vi "数据采集传输系统.vi"() -> ()   [LabVIEW 2016, in "数据传输系统.lvlib"]
uses:
  <vilib>/Utility/miscctls.llb/LVPointTypeDef.ctl
  <vilib>/Utility/config.llb/Read Key (String).vi
  <vilib>/Utility/config.llb/Read Key (Boolean).vi
  <vilib>/Utility/config.llb/Read Key (I32).vi
  <vilib>/Utility/config.llb/Write Key (String).vi
  <vilib>/Utility/config.llb/Write Key (U32).vi
  <vilib>/Utility/config.llb/Write Key (I32).vi
  <vilib>/Utility/config.llb/Write Key (Boolean).vi
  <vilib>/Utility/config.llb/NI_LVConfig.lvlib
  data/FreeMem.dll
  <vilib>/ptbypt/NI_PtbyPt.lvlib
panel:
  in  "实时数据发送时间间隔/min":i32=1
  in  "数据组合发送":bool
  in  "日志、参数发送":bool
  in  "2011发送":bool
  in  "判断数据反馈":bool
  in  "数据发送协议":enum16{"2005-212协议", "2017-212协议"}(ring)=enum."2017-212协议"
  in  "数据发送通道":enum16{"TCP", "VISA"}(ring)
  in  "baud rate":u32=9600 caption="波特率"
  in  "VISA resource name":refnum<visa-resource-name> caption="VISA资源名称"
  in  "查询质控数据起始时间":bool
  in  "返回主界面":bool
  out "零点核查索引起始时间":string
  out "跨度核查索引起始时间":string
  out "加标回收索引起始时间":string
  out "标样核查索引起始时间":string
  out "数据接收超时指示灯":bool
  in  "重发时间":T1(ring)
  in  "重发日期":T2(ring)
  in  "锁":bool
  in  "开机启动":bool
  in  "确定更改起始时间":bool
  in  "更改起始时间":bool
  in  "数据发送起始时间":timestamp format="%<%.3X\n%Y/%m/%d>T"
  in  "每周自动重发":bool=TRUE
  in  "确定":bool
  in  "返回":bool
  in  "PW":string
  in  "MN":string
  in  "PORT":string
  in  "IP":string
  in  "站点设备":string
  in  "站点名称":string
  out "设置超时时间/min":i32=1
  out "空闲时间/s":string
  out "状态信息":T3={"1st Error to Convert "=63, "步骤 "=enum."打开连接", "元素"="实时数据", "TCP服务端掉线计数"=4, "TCP掉线时间节点"="2019/05/08 15:24:17"} {"1st Error to Convert" items=["无错误", "参数错误", "内存已满", "超出区域", "文件结束", "文件已打开", "一般文件IO错误", "未找到文件", "文件权限错误", "磁盘已满", "路径副本", "打开过多文件", "未启用", "未找到资源文件", "无法添加资源", "未找到资源", "未找到图像", "图像内存错误", "画笔不存在", "配置错误类型", "配置未找到解析段", "配置解析错误", "配置内存错误", "错误外部代码格式", "错误外部代码偏移量", "外部代码不存在", "空窗口", "销毁窗口错误", "空菜单", "打印已中止", "错误打印记录", "打印驱动程序错误", "打印时窗口错误", "打印时内存错误", "打印对话框错误", "一般打印错误", "无效设备引用句柄", "设备未找到", "设备参数错误", "设备单位错误", "无法打开设备", "设备调用已中止", "一般错误", "用户已取消", "对象ID过低", "对象ID过高", "对象不在堆中", "未知的堆", "错误DefProc ID", "DefProc不在表格中", "范围外信息", "空方法", "未知信息", "不支持管理器调用", "错误地址", "连接过程中", "连接超时", "连接过程中", "不支持网络属性", "网络错误", "正在使用的地址", "系统缺少内存", "连接已中止", "连接已拒绝", "连接未建立", "连接已建立", "连接已关闭", "初始化错误（交互应用程序管理器）", "错误事件发生", "等待无约束事件发生处理程序", "事件发生队列溢出", "错误路径", "未发出信号量", "未识别类型（交互应用程序管理器）"]}
  out "系统时间":string
  out "实时小时数据上传":bool
  out "系统状态改变":bool
  out "软件版本":string
  out "掉线指示":bool
  out "核查数据上传":bool
  out "通信状态":bool
  out "配置信息":T4
  in  "参数配置":bool
  out "查询数据发送":bool
  out "读取报文显示":string
  out "发送报文显示":string
  out "心跳包":bool
  in  "参数数值":T5={"CODMn"=TRUE, "CODCr"=TRUE, "DO"=TRUE, "铜"=TRUE, "PH"=TRUE, "氨氮"=TRUE, "比电导率"=TRUE, "水温"=TRUE, "盐度(海水)"=TRUE, "浊度"=TRUE, "总氮"=TRUE, "总磷"=TRUE, "叶绿素a"=TRUE, "藻密度"=TRUE, "水位"=TRUE, "流速"=TRUE, "瞬时流量"=TRUE, "累积流量"=TRUE}
  in  "系统编码选择框":string(combo)="地表水质量监测"
  out "主队列输出":refnum<queue>
  in  "TCP掉线时间节点":string
  out "TCP服务端掉线计数":i32
  out "元素":string
  out "步骤":T6(ring)
  out "1st Error to Convert":i32(ring)=56 items=["无错误", "参数错误", "内存已满", "超出区域", "文件结束", "文件已打开", "一般文件IO错误", "未找到文件", "文件权限错误", "磁盘已满", "路径副本", "打开过多文件", "未启用", "未找到资源文件", "无法添加资源", "未找到资源", "未找到图像", "图像内存错误", "画笔不存在", "配置错误类型", "配置未找到解析段", "配置解析错误", "配置内存错误", "错误外部代码格式", "错误外部代码偏移量", "外部代码不存在", "空窗口", "销毁窗口错误", "空菜单", "打印已中止", "错误打印记录", "打印驱动程序错误", "打印时窗口错误", "打印时内存错误", "打印对话框错误", "一般打印错误", "无效设备引用句柄", "设备未找到", "设备参数错误", "设备单位错误", "无法打开设备", "设备调用已中止", "一般错误", "用户已取消", "对象ID过低", "对象ID过高", "对象不在堆中", "未知的堆", "错误DefProc ID", "DefProc不在表格中", "范围外信息", "空方法", "未知信息", "不支持管理器调用", "错误地址", "连接过程中", "连接超时", "连接过程中", "不支持网络属性", "网络错误", "正在使用的地址", "系统缺少内存", "连接已中止", "连接已拒绝", "连接未建立", "连接已建立", "连接已关闭", "初始化错误（交互应用程序管理器）", "错误事件发生", "等待无约束事件发生处理程序", "事件发生队列溢出", "错误路径", "未发出信号量", "未识别类型（交互应用程序管理器）"]
  out "QN":string
  out "时间QN":string
  out "系统编码ST":string
  out "命令编码CN":string
  out "密码PW":string
  out "设备编码MN":string
  out "拆分包及应答Flag":string
  out "数据":string
  in  "实时数据参数选择框":T7={"水样测量数据"=FALSE, "零点核查数据"=TRUE, "跨度核查数据"=TRUE, "加标回收数据"=TRUE, "平行样数据"=FALSE, "标样核查"=TRUE, "集成干预测试"=TRUE}
  out "数据输出":string
  in  "table元素":string
  out "空闲时间":dbl
  out "错误输出":errorcluster
  # "数 据 采 集 传 输 系 统"
  # "读取的参数区"
  # "水样测量数据"
  # "空白测试数据"
  # "跨度核查数据"
  # "加标回收数据"
  # "平行样数据"
  # "标样核查"
  # "集成干预测试"
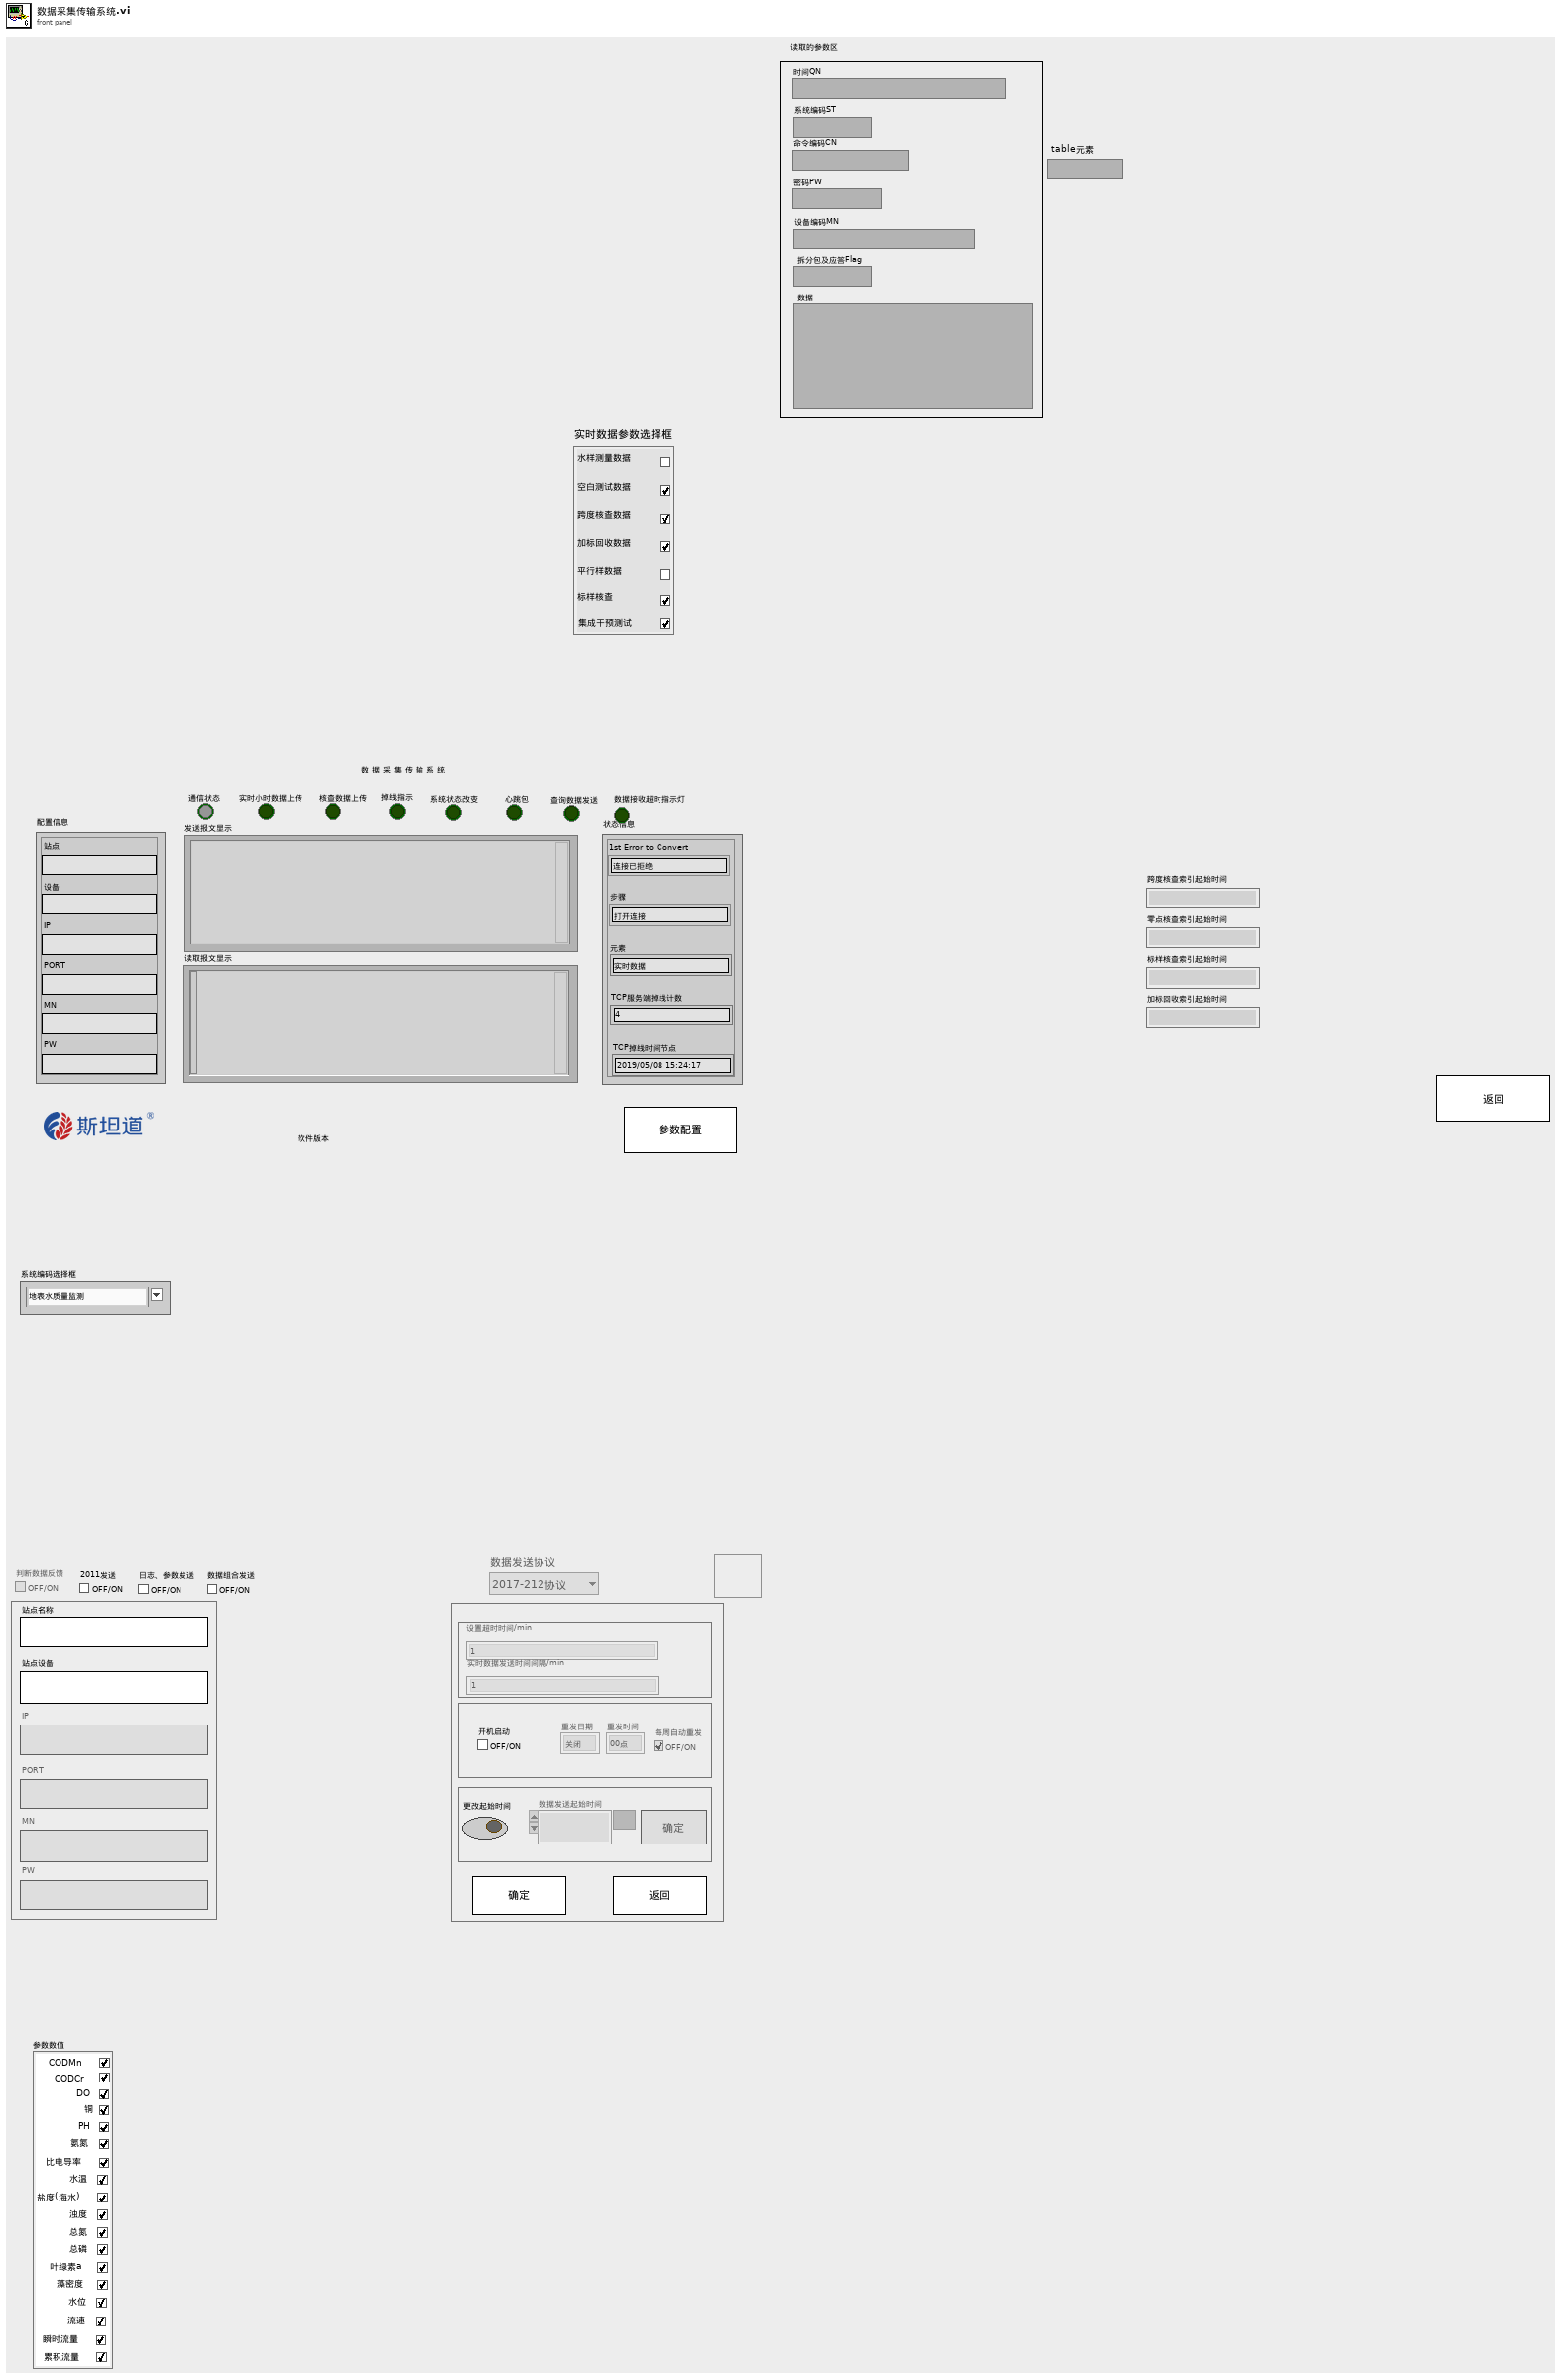
[diagram p1: front panel]
types:
  T1 = enum16{"00点", "01点", "02点", "03点", "04点", "05点", "06点", "07点", "08点", "09点", "10点", "11点", "12点", "13点", "14点", "15点", "16点", "17点", "18点", "19点", "20点", "21点", "22点", "23点"}
  T2 = enum16{"关闭", "星期日", "星期一", "星期二", "星期三", "星期四", "星期五", "星期六"}
  T3 = cluster{"1st Error to Convert ":i32, "步骤 ":enum16{"初始化", "打开连接", "表格比对", "发送数据", "读取数据", "数据处理"}, "元素":string, "TCP服务端掉线计数":i32, "TCP掉线时间节点":string}
  T4 = cluster{"站点":string, "设备":string, "IP":string, "PORT":string, "MN":string, "PW":string}
  T5 = cluster{"CODMn":bool, "CODCr":bool, "DO":bool, "铜":bool, "PH":bool, "氨氮":bool, "比电导率":bool, "水温":bool, "盐度(海水)":bool, "浊度":bool, "总氮":bool, "总磷":bool, "叶绿素a":bool, "藻密度":bool, "水位":bool, "流速":bool, "瞬时流量":bool, "累积流量":bool}
  T6 = enum16{"初始化", "打开连接", "表格比对", "发送数据", "读取数据", "数据处理"}
  T7 = cluster{"水样测量数据":bool, "零点核查数据":bool, "跨度核查数据":bool, "加标回收数据":bool, "平行样数据":bool, "标样核查":bool, "集成干预测试":bool}
  T8 = typedef "NI_LVConfig.lvlib/Config Data RefNum.ctl" = refnum<k1>
  T9 = typedef "LVDateTimeRec.ctl" = cluster{"秒数的小数部分":dbl, "秒":i32, "分":i32, "时":i32, "日":i32, "月":i32, "年":i32, "天数（周）":i32, "天数（年）":i32, "DST":i32}
  T10 = cluster{"PH":string[][], "CODCr":string[][], "氨氮":string[][], "CODMn":string[][], "总氮":string[][], "总磷":string[][], "电导率":string[][], "水温":string[][], "DO":string[][], "浊度":string[][], "叶绿素":string[][], "藻密度":string[][], "铜":string[][], "盐度":string[][], "水位":string[][], "流速":string[][], "瞬时流量":string[][], "累积流量":string[][]}
  T11 = typedef "LVPointTypeDef.ctl" = cluster{"Horizontal":i16, "Vertical":i16}
  T12 = enum8{"Enabled", "Disabled", "Disabled and Grayed Out"}
  T13 = enum16{"水样测试", "小时数据", "日志信息", "报警信息", "零点核查", "标样核查", "平行样", "加标回收"}
  T14 = typedef "imagedata.ctl" = cluster{"image type":i32, "image depth":i32, "image":u8[], "mask":u8[], "colors":u32[], "Rectangle":cluster{"left":i16, "top":i16, "right":i16, "bottom":i16}}
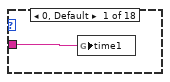
[diagram p6: hidden frame]
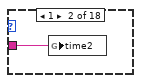
[diagram p7: hidden frame]
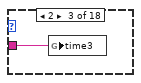
[diagram p8: hidden frame]
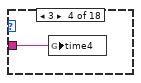
[diagram p9: hidden frame]
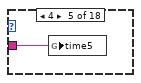
[diagram p10: hidden frame]
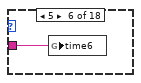
[diagram p11: hidden frame]
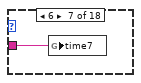
[diagram p12: hidden frame]
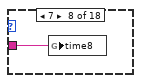
[diagram p13: hidden frame]
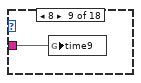
[diagram p14: hidden frame]
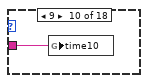
[diagram p15: hidden frame]
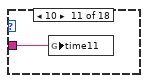
[diagram p16: hidden frame]
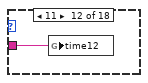
[diagram p17: hidden frame]
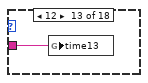
[diagram p18: hidden frame]
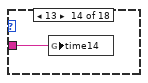
[diagram p19: hidden frame]
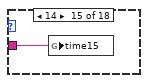
[diagram p20: hidden frame]
diagram:
  w27 = 0 ("索引")
  # "上传本地时间点的实时数据"
  # "目前时间太短，如果掉线了，数据存不了临时表格"
  n1 = Cluster To Array(cluster="参数数值") -> (array=w38:bool[])
  n2 = for {
    tunnel: w38 -> [_] mode=indexing
    tunnel: [w72] -> w37
    i -> [w72]
    w61 = "线程一数据重发功能" ("section")
    # "初始化水样搜索起始时间"
    n3 = case shown="3" w72 {
      tunnel: [w103 w105 w107 w109 w111 w113 w115 w117 w119 w121 w123 w125 w127 w129 w131 w133 w135 w137] -> w76
      frame 0, Default {
        n4 = control-ref of="CODMn"() -> (w104:refnum<vi>)
        n5 = property class="Bool (严格)"(reference=w104) -> ("Label.Text"=w103:string)  [unwired: 1 in, 2 out]
      }
      frame 1 {
        n6 = control-ref of="CODCr"() -> (w106:refnum<vi>)
        n7 = property class="Bool (严格)"(reference=w106) -> ("Label.Text"=w105:string)  [unwired: 1 in, 2 out]
      }
      frame 2 {
        n8 = control-ref of="DO"() -> (w108:refnum<vi>)
        n9 = property class="Bool (严格)"(reference=w108) -> ("Label.Text"=w107:string)  [unwired: 1 in, 2 out]
      }
      frame 3 {
        n10 = control-ref of="铜"() -> (w110:refnum<vi>)
        n11 = property class="Bool (严格)"(reference=w110) -> ("Label.Text"=w109:string)  [unwired: 1 in, 2 out]
      }
      frame 4 {
        n12 = control-ref of="PH"() -> (w112:refnum<vi>)
        n13 = property class="Bool (严格)"(reference=w112) -> ("Label.Text"=w111:string)  [unwired: 1 in, 2 out]
      }
      frame 5 {
        n14 = control-ref of="氨氮"() -> (w114:refnum<vi>)
        n15 = property class="Bool (严格)"(reference=w114) -> ("Label.Text"=w113:string)  [unwired: 1 in, 2 out]
      }
      frame 6 {
        n16 = control-ref of="比电导率"() -> (w116:refnum<vi>)
        n17 = property class="Bool (严格)"(reference=w116) -> ("Label.Text"=w115:string)  [unwired: 1 in, 2 out]
      }
      frame 7 {
        n18 = control-ref of="水温"() -> (w118:refnum<vi>)
        n19 = property class="Bool (严格)"(reference=w118) -> ("Label.Text"=w117:string)  [unwired: 1 in, 2 out]
      }
      frame 8 {
        n20 = control-ref of="盐度(海水)"() -> (w120:refnum<vi>)
        n21 = property class="Bool (严格)"(reference=w120) -> ("Label.Text"=w119:string)  [unwired: 1 in, 2 out]
      }
      frame 9 {
        n22 = control-ref of="浊度"() -> (w122:refnum<vi>)
        n23 = property class="Bool (严格)"(reference=w122) -> ("Label.Text"=w121:string)  [unwired: 1 in, 2 out]
      }
      frame 10 {
        n24 = control-ref of="总氮"() -> (w124:refnum<vi>)
        n25 = property class="Bool (严格)"(reference=w124) -> ("Label.Text"=w123:string)  [unwired: 1 in, 2 out]
      }
      frame 11 {
        n26 = control-ref of="总磷"() -> (w126:refnum<vi>)
        n27 = property class="Bool (严格)"(reference=w126) -> ("Label.Text"=w125:string)  [unwired: 1 in, 2 out]
      }
      frame 12 {
        n28 = control-ref of="叶绿素a"() -> (w128:refnum<vi>)
        n29 = property class="Bool (严格)"(reference=w128) -> ("Label.Text"=w127:string)  [unwired: 1 in, 2 out]
      }
      frame 13 {
        n30 = control-ref of="藻密度"() -> (w130:refnum<vi>)
        n31 = property class="Bool (严格)"(reference=w130) -> ("Label.Text"=w129:string)  [unwired: 1 in, 2 out]
      }
      frame 14 {
        n32 = control-ref of="水位"() -> (w132:refnum<vi>)
        n33 = property class="Bool (严格)"(reference=w132) -> ("Label.Text"=w131:string)  [unwired: 1 in, 2 out]
      }
      frame 15 {
        n34 = control-ref of="流速"() -> (w134:refnum<vi>)
        n35 = property class="Bool (严格)"(reference=w134) -> ("Label.Text"=w133:string)  [unwired: 1 in, 2 out]
      }
      frame 16 {
        n36 = control-ref of="瞬时流量"() -> (w136:refnum<vi>)
        n37 = property class="Bool (严格)"(reference=w136) -> ("Label.Text"=w135:string)  [unwired: 1 in, 2 out]
      }
      frame 17 {
        n38 = control-ref of="累积流量"() -> (w138:refnum<vi>)
        n39 = property class="Bool (严格)"(reference=w138) -> ("Label.Text"=w137:string)  [unwired: 1 in, 2 out]
      }
    }
    n40 = call <vilib>:"Application Directory.vi"() -> ("Application Directory"=w82:path)
    n41 = Build Path(base path=w82, name or relative path="data\\Set.ini" ("名称或相对路径")) -> (appended path=w80:path)
    n42 = call <vilib>:"Open Config Data.vi"("configuration file path"=w80) -> ("error out"=w78:errorcluster, "refnum"=w79:T8)  [unwired: 8 in, 1 out]
    n43 = call-poly <vilib>:"Read Key.vi"("section"="线程一数据搜索起始时间", "error in (no error)"=w78, "key"=w76, "refnum"=w79) -> ("error out"=w70:errorcluster, "value"=w73:string, "refnum out"=w71:T8)  [unwired: 4 in, 1 out]
    n44 = Empty String/Path?(string/path=w73) -> (empty?=w75:bool)
    n45 = case shown="真" w75 {
      tunnel: [w83 "1904/01/01 00:00:00"] -> w74
      tunnel: w73 -> [w83 _]
      frame False {
      }
      frame True {
      }
    }
    n46 = call-poly <vilib>:"Read Key.vi"("section"=w61, "error in (no error)"=w70, "key"="重发功能", "refnum"=w71) -> ("error out"=w64:errorcluster, "value"=w68:bool, "refnum out"=w65:T8)  [unwired: 4 in, 1 out]
    n47 = local write "每周自动重发"(w68) -> ()
    n48 = call-poly <vilib>:"Read Key.vi"("section"=w61, "error in (no error)"=w64, "key"="重发日期", "refnum"=w65) -> ("error out"=w62:errorcluster, "value"=w58:i32, "refnum out"=w63:T8)  [unwired: 4 in, 1 out]
    n49 = local write "重发日期"(w58) -> ()
    n50 = case shown="3" w72 {
      tunnel: w74 -> [w85 w86 w87 w88 w89 w90 w91 w92 w93 w94 w95 w96 w97 w98 w99 w100 w101 w102]
      frame 0, Default {
        n51 = global write "全局 水样时间.vi" "time1"(w85) -> ()
      }
      frame 1 {
        n52 = global write "全局 水样时间.vi" "time2"(w86) -> ()
      }
      frame 2 {
        n53 = global write "全局 水样时间.vi" "time3"(w87) -> ()
      }
      frame 3 {
        n54 = global write "全局 水样时间.vi" "time4"(w88) -> ()
      }
      frame 4 {
        n55 = global write "全局 水样时间.vi" "time5"(w89) -> ()
      }
      frame 5 {
        n56 = global write "全局 水样时间.vi" "time6"(w90) -> ()
      }
      frame 6 {
        n57 = global write "全局 水样时间.vi" "time7"(w91) -> ()
      }
      frame 7 {
        n58 = global write "全局 水样时间.vi" "time8"(w92) -> ()
      }
      frame 8 {
        n59 = global write "全局 水样时间.vi" "time9"(w93) -> ()
      }
      frame 9 {
        n60 = global write "全局 水样时间.vi" "time10"(w94) -> ()
      }
      frame 10 {
        n61 = global write "全局 水样时间.vi" "time11"(w95) -> ()
      }
      frame 11 {
        n62 = global write "全局 水样时间.vi" "time12"(w96) -> ()
      }
      frame 12 {
        n63 = global write "全局 水样时间.vi" "time13"(w97) -> ()
      }
      frame 13 {
        n64 = global write "全局 水样时间.vi" "time14"(w98) -> ()
      }
      frame 14 {
        n65 = global write "全局 水样时间.vi" "time15"(w99) -> ()
      }
      frame 15 {
        n66 = global write "全局 水样时间.vi" "time16"(w100) -> ()
      }
      frame 16 {
        n67 = global write "全局 水样时间.vi" "time17"(w101) -> ()
      }
      frame 17 {
        n68 = global write "全局 水样时间.vi" "time18"(w102) -> ()
      }
    }
    n69 = call-poly <vilib>:"Read Key.vi"("section"=w61, "error in (no error)"=w62, "key"="重发时间", "refnum"=w63) -> ("error out"=w59:errorcluster, "value"=w57:i32, "refnum out"=w60:T8)  [unwired: 4 in, 1 out]
    n70 = local write "重发时间"(w57) -> ()
    n71 = call <vilib>:"Close Config Data.vi"("error in (no error)"=w59, "refnum"=w60) -> ()  [unwired: 8 in, 2 out]
  }
  n72 = vi-ref "数据传输系统.lvlib:主动上传工控机周期和模式 (子VI).vi"() -> (w18:refnum<vi>)
  n73 = property class="VI"(reference=w18) -> ("Name"=w19:string)  [unwired: 1 in, 2 out]
  n74 = vi-ref "数据传输系统.lvlib:核查数据和日志信息入发送队列 (子VI).vi"() -> (w9:refnum<vi>)
  n75 = local read "实时小时数据上传"() -> (w5:bool)
  n76 = Open VI Reference(type specifier VI Refnum (for type only)=refnum<vi> refnum, vi path=w19, options=128 ("选项")) -> (vi reference=w21:refnum<vi>, error out=w23:errorcluster)  [unwired: 3 in]
  n77 = local read "核查数据上传"() -> (w8:bool)
  n78 = local read "查询数据发送"() -> (w7:bool)
  n79 = local read "日志、参数发送"() -> (w3:bool)
  n80 = property class="VI"(reference=w9) -> ("Name"=w16:string)  [unwired: 1 in, 2 out]
  n81 = local read "步骤"() -> (w6:T6)
  n82 = call-by-ref "?"(reference=w21, error in=w23) -> (reference out=w25:refnum<vi>, error out=w24:errorcluster, "系统状态改变"=→"系统状态改变":bool)  [unwired: 11 in]
  n83 = local read "数据发送协议"() -> (w4:enum16{"2005-212协议", "2017-212协议"})
  n84 = Close Reference(reference=w25, error in (no error)=w24) -> ()  [unwired: 1 out]
  n85 = Open VI Reference(type specifier VI Refnum (for type only)=refnum<vi> refnum, vi path=w16, options=128 ("选项")) -> (vi reference=w14:refnum<vi>, error out=w12:errorcluster)  [unwired: 3 in]
  n86 = call-by-ref "?"(reference=w14, error in=w12, "实时数据参数选择框"="实时数据参数选择框", "实时数据发送时间间隔/min"="实时数据发送时间间隔/min", "日志、参数发送输入"=w3, "数据发送协议输入"=w4, "实时小时数据上传输入"=w5, "步骤输入"=w6, "查询数据发送输入"=w7, "核查数据上传输入"=w8) -> (reference out=w10:refnum<vi>, error out=w11:errorcluster)  [unwired: 4 in]
  n87 = Obtain Queue(name (unnamed)="数据发送" ("名称（未命名）"), element data type="") -> (queue out=w26:refnum<queue>, error out=w41:errorcluster)  [unwired: 3 in, 1 out]
  n88 = Obtain Queue(name (unnamed)="实时数据参数选择" ("名称（未命名）"), element data type="") -> (queue out=w42:refnum<queue>, error out=w40:errorcluster)  [unwired: 3 in, 1 out]
  n89 = Close Reference(reference=w10, error in (no error)=w11) -> ()  [unwired: 1 out]
  n90 = while "While循环" {
    tunnel: w26 -> [w149]
    tunnel: w42 -> [w153]
    tunnel: w41 -> [w152]
    tunnel: w40 -> [w151]
    stop <- FALSE stop-if-true
    # "判定数据发送时要发送实时数据"
    # "所有的主动上传数据都是有数据才会上传"
    n91 = Get Queue Status(queue=w149) -> (# elements in queue=w141:i32)  [unwired: 2 in, 7 out]
    n92 = local read "查询数据发送"() -> (w147:bool)
    n93 = global read "全局 数据发送重叠.vi" "主动上报数据中"() -> (w139:bool)
    n94 = Not Equal To 0?(x=w141) -> (x != 0?=w148:bool)
    n95 = And(x=w148, y=w147) -> (x .and. y?=w140:bool)
    n96 = call <vilib>:"Boolean Crossing PtByPt.vi"("direction"=enum16{"either", "false-true", "true-false"}."false-true", "input"=w140) -> ("crossing"=w146:bool)  [unwired: 1 in]
    n97 = Not(x=w139) -> (.not. x?=w143:bool)
    n98 = Not(x=w147) -> (.not. x?=w144:bool)
    n99 = case shown="真" w146 {
      frame False {
      }
      frame True {
        n100 = Get Date/Time In Seconds() -> (seconds since 1Jan1904=w159:timestamp)
        n101 = Seconds To Date/Time(time stamp (now)=w159) -> (date time rec=w156:T9)  [unwired: 1 in]
        n102 = Date/Time To Seconds(2:w156) -> (0:w158:timestamp)  [unwired: 1 in]
        n103 = Format Date/Time String(time format string (%c)="%Y/%m/%d %H:%M:%S" ("时间格式字符串(%c)"), seconds (now)=w158) -> (date/time string=w155:string)  [unwired: 1 in]
        n104 = global write "全局 数据发送重叠.vi" "数据发送重叠开始时间戳"(w155) -> ()
      }
    }
    n105 = Compound Arithmetic op=AND ("复合运算")(w144, w143) -> (w142:bool)
    n106 = Wait (ms)(milliseconds to wait=u32 1000 ("等待时间（毫秒）")) -> ()  [unwired: 1 out]
    n107 = case shown="真" w142 {
      tunnel: w149 -> [_ w169]
      tunnel: w153 -> [_ w168]
      tunnel: w152 -> [_ w167]
      tunnel: w151 -> [_ w166]
      tunnel: w141 -> [_ w162]
      tunnel: w140 -> [_ w161]
      frame False {
        n108 = local write "核查数据上传"(FALSE ("数据上传")) -> ()
      }
      frame True {
        n109 = Equal To 0?(x=w162) -> (x = 0?=w163:bool)
        n110 = global write "全局 数据发送重叠.vi" "数据发送重叠"(w161) -> ()
        n111 = Not(x=w163) -> (.not. x?=w164:bool)
        n112 = local write "核查数据上传"(w164) -> ()
        n113 = Dequeue Element(queue=w169, error in (no error)=w167) -> (element=w165:string)  [unwired: 1 in, 3 out]
        n114 = case shown="\"send\"" w165 {
          tunnel: w168 -> [_ w171 _ _ _ _ _ _ _ _ _]
          tunnel: w166 -> [_ w170 _ _ _ _ _ _ _ _ _]
          frame "假", Default {
          }
          frame "send" {
            # "间隔时间上传"
            n115 = while {
              tunnel: w171 -> [w175]
              tunnel: w170 -> [w172]
              stop <- w176 stop-if-true
              n116 = Dequeue Element(queue=w175, error in (no error)=w172) -> (queue out=w174:refnum<queue>, element=w177:string)  [unwired: 1 in, 2 out]
              n117 = case shown="\"空白测试\"" w177 {
                tunnel: [_ _ _ w343 _ _ _ w550] -> w176
                tunnel: w174 -> [_ _ _ _ _ _ _ w553]
                frame "水样测试" {
                  n118 = flat-sequence {
                    frame #0 {
                      n119 = global write "全局 小时数据发送次数.vi" "小时数据发送次数"(0 ("小时数据发送次数")) -> ()
                      n120 = global write "全局 实时数据参数.vi" "实时数据参数"("水样测试") -> ()
                      n121 = global write "全局1.vi" "枚举"(enum16{"返回请求应答", "上传数据", "返回执行结果"}."上传数据" ("枚举")) -> ()
                    }
                    frame #1 {
                      n122 = call "从数据库获取数据通用可配置(子VI).vi"("table输入"="实时数据" ("新元素/子数组"), "列队名（唯一）"="a") -> ()  [unwired: 8 in, 2 out]
                    }
                    frame #2 {
                      n123 = call "实时小时数据处理整合 (子VI).vi"("枚举"=enum16{"实时数据排序", "小时数据排序"}."实时数据排序") -> ("已排序的数组"=w184:string[])  [unwired: 10 in]
                      n124 = Array Size(array=w184) -> (size(s)=w185:i32)
                      n125 = global write "全局 数据数组大小.vi" "数据数组大小"(w185) -> ()
                    }
                    frame #3 {
                      n126 = while {
                        stop <- w190 stop-if-true
                        n127 = property on="TCP服务端掉线计数" class="DigNum (严格)"() -> ("Value"=w193:i32)  [unwired: 2 in, 2 out]
                        n128 = Greater Or Equal?(x=w193, y=1) -> (x >= y?=w192:bool)
                        n129 = case shown="假" w192 {
                          frame False {
                            n130 = global read "全局 数据数组大小.vi" "数据数组大小"() -> (w195:i32)
                            n131 = Greater Than 0?(x=w195) -> (x > 0?=w196:bool)
                            n132 = case shown="真" w196 {
                              frame False {
                              }
                              frame True {
                                n133 = local read "MN"() -> (w202:string)
                                n134 = local read "PW"() -> (w201:string)
                                n135 = local read "数据发送通道"() -> (w200:enum16{"TCP", "VISA"})
                                n136 = call "数据编码.vi"("table输入"="实时数据" ("新元素/子数组"), "MN"=w202, "PW"=w201) -> ("通讯包字符串"=w197:string)  [unwired: 11 in, 1 out]
                                n137 = local write "发送报文显示"(w197) -> ()
                                n138 = call "VISATCP组合选择发送.vi"("数据发送通道"=w200, "命令"="write", "写入缓冲区"=w197) -> ("错误输出"=→"错误输出":errorcluster)  [unwired: 9 in, 3 out]
                                n139 = Build Array(w197) -> (w204:string[])
                                n140 = call "发送数据记录到文档(子VI).vi"("数组"=w204) -> ()  [unwired: 9 in, 1 out]
                                "核查数据上传" <- TRUE ("主动数据上传")
                              }
                            }
                          }
                          frame True {
                          }
                        }
                        n141 = Wait (ms)(milliseconds to wait=u32 500 ("等待时间（毫秒）")) -> ()  [unwired: 1 out]
                        n142 = global read "全局 数据数组大小.vi" "数据数组大小"() -> (w187:i32)
                        n143 = global read "全局 小时数据发送次数.vi" "小时数据发送次数"() -> (w191:i32)
                        n144 = Decrement(x=w187) -> (x-1=w186:i32)
                        n145 = Greater Or Equal?(x=w191, y=w186) -> (x >= y?=w189:bool)
                        n146 = Compound Arithmetic op=OR ("复合运算")(w189) -> (w190:bool)
                      }
                    }
                  }
                }
                frame "空白测试" {
                  n147 = flat-sequence {
                    frame #0 {
                      n148 = global write "全局 小时数据发送次数.vi" "小时数据发送次数"(0 ("小时数据发送次数")) -> ()
                      n149 = global write "全局 实时数据参数.vi" "实时数据参数"("空白测试") -> ()
                      n150 = global write "全局1.vi" "枚举"(enum16{"返回请求应答", "上传数据", "返回执行结果"}."上传数据" ("枚举")) -> ()
                    }
                    frame #1 {
                      n151 = call "从数据库获取数据通用可配置(子VI).vi"("table输入"="实时数据" ("新元素/子数组"), "列队名（唯一）"="b") -> ()  [unwired: 8 in, 2 out]
                    }
                    frame #2 {
                      n152 = for {
                        N: 5 -> [_]
                        i -> [w213]
                        # "行数大于零"
                        n153 = case shown="3" w213 {
                          tunnel: [w217 w218 w219 w220 w221] -> w212
                          frame 0, Default {
                            n154 = global read "全局 所有参数.vi" "氨氮"() -> (w217:string[][])
                          }
                          frame 1 {
                            n155 = global read "全局 所有参数.vi" "总氮"() -> (w218:string[][])
                          }
                          frame 2 {
                            n156 = global read "全局 所有参数.vi" "总磷"() -> (w219:string[][])
                          }
                          frame 3 {
                            n157 = global read "全局 所有参数.vi" "CODMn"() -> (w220:string[][])
                          }
                          frame 4 {
                            n158 = global read "全局 所有参数.vi" "CODCr"() -> (w221:string[][])
                          }
                        }
                        n159 = Array Size(array=w212) -> (size(s)=w215:i32[])
                        n160 = Index Array(array=w215) -> (element=w214:i32)  [unwired: 1 in]
                        n161 = Greater Than 0?(x=w214) -> (x > 0?=w216:bool)
                        n162 = case shown="真" w216 {
                          tunnel: w213 -> [_ w227]
                          tunnel: w214 -> [_ _]
                          tunnel: w212 -> [_ w225]
                          frame False {
                          }
                          frame True {
                            # "最新时间戳加1分钟"
                            n163 = Index Array(array=w225, index (row)=0 ("禁用的索引 (行)"), index (col)=0 ("禁用的索引 (列)")) -> (element=w224:string)
                            n164 = call "日期时间字符串转换分钟数加一.vi"("data[0]"=w224) -> ("日期/时间字符串"=w223:string)  [unwired: 10 in]
                            n165 = case shown="0, 默认" w227 {
                              tunnel: w223 -> [w228 w229 w230 w231 w232]
                              frame 0, Default {
                                n166 = global write "全局 时间2.vi" "氨氮零点核查索引起始时间"(w228) -> ()
                              }
                              frame 1 {
                                n167 = global write "全局 时间2.vi" "总氮零点核查索引起始时间"(w229) -> ()
                              }
                              frame 2 {
                                n168 = global write "全局 时间2.vi" "总磷零点核查索引起始时间"(w230) -> ()
                              }
                              frame 3 {
                                n169 = global write "全局 时间2.vi" "CODMn零点核查索引起始时间"(w231) -> ()
                              }
                              frame 4 {
                                n170 = global write "全局 时间2.vi" "CODCr零点核查索引起始时间"(w232) -> ()
                              }
                            }
                          }
                        }
                      }
                    }
                    frame #3 {
                      n171 = call <vilib>:"Application Directory.vi"() -> ("Application Directory"=w246:path)
                      n172 = Build Path(base path=w246, name or relative path="data\\hecha.ini" ("名称或相对路径")) -> (appended path=w244:path)
                      n173 = call <vilib>:"Open Config Data.vi"("configuration file path"=w244) -> ("error out"=w240:errorcluster, "refnum"=w243:T8)  [unwired: 8 in, 1 out]
                      n174 = call "数据处理整合 (子VI).vi"("枚举"=enum16{"实时数据排序", "小时数据排序"}."实时数据排序") -> ("已排序的数组"=w249:string[])  [unwired: 10 in]
                      n175 = vi-ref "全局 时间2.vi"() -> (w242:refnum<vi>)
                      n176 = Array Size(array=w249) -> (size(s)=w248:i32)
                      n177 = call <userlib>:"Write Panel to INI__ogtk.vi"("error in (no error)"=w240, "VI ref"=w242, "refnum"=w243) -> ("error out"=w239:errorcluster, "refnum out"=w241:T8)  [unwired: 7 in]
                      n178 = call <vilib>:"Close Config Data.vi"("error in (no error)"=w239, "refnum"=w241) -> ("error out"=w234:errorcluster, "file path"=w233:path)  [unwired: 8 in]
                      n179 = global write "全局 数据数组大小.vi" "数据数组大小"(w248) -> ()
                      n180 = Open/Create/Replace File(file path (use dialog)=w233, error in=w234) -> (refnum out=w237:refnum<file>, error out=w238:errorcluster)  [unwired: 4 in, 1 out]
                      n181 = Flush File(refnum=w237, error in=w238) -> (refnum out=w236:refnum<file>, error out=w235:errorcluster)
                      n182 = Close File(refnum=w236, error in=w235) -> ()  [unwired: 2 out]
                    }
                    frame #4 {
                      n183 = while {
                        stop <- w252 stop-if-true
                        n184 = property on="TCP服务端掉线计数" class="DigNum (严格)"() -> ("Value"=w256:i32)  [unwired: 2 in, 2 out]
                        n185 = Greater Or Equal?(x=w256, y=1) -> (x >= y?=w255:bool)
                        n186 = case shown="假" w255 {
                          frame False {
                            n187 = global read "全局 数据数组大小.vi" "数据数组大小"() -> (w259:i32)
                            n188 = Greater Than 0?(x=w259) -> (x > 0?=w258:bool)
                            n189 = case shown="真" w258 {
                              frame False {
                              }
                              frame True {
                                w260 = 0 ("禁用的索引 (列)")
                                n190 = global read "插值后的新数组.vi" "插值后的数组元素"() -> (w270:T10)
                                n191 = local read "MN"() -> (w266:string)
                                n192 = local read "PW"() -> (w265:string)
                                n193 = local read "数据发送通道"() -> (w264:enum16{"TCP", "VISA"})
                                n194 = call "数据编码.vi"("table输入"="实时数据" ("新元素/子数组"), "MN"=w266, "PW"=w265) -> ("通讯包字符串"=w262:string)  [unwired: 11 in, 1 out]
                                n195 = Unbundle By Name(w270) -> ("氨氮"=w269:string[][])
                                n196 = local write "发送报文显示"(w262) -> ()
                                n197 = Build Array(w262) -> (w272:string[])
                                n198 = call "VISATCP组合选择发送.vi"("数据发送通道"=w264, "命令"="write", "写入缓冲区"=w262) -> ("错误输出"=w261:errorcluster)  [unwired: 9 in, 3 out]
                                n199 = Index Array(array=w269, index (row)=w260, index (col)=w260) -> (element=w268:string)
                                n200 = call "发送数据记录到文档(子VI).vi"("数组"=w272) -> ()  [unwired: 9 in, 1 out]
                                n201 = local write "错误输出"(w261) -> ()
                                n202 = call "日期时间字符串转换分钟数加一.vi"("data[0]"=w268) -> ("日期/时间字符串"=w267:string)  [unwired: 10 in]
                                n203 = global write "全局 时间2.vi" "零点核查索引起始时间"(w267) -> ()
                                n204 = local write "核查数据上传"(TRUE ("数据上传")) -> ()
                              }
                            }
                          }
                          frame True {
                          }
                        }
                        n205 = Wait (ms)(milliseconds to wait=u32 500 ("等待时间（毫秒）")) -> ()  [unwired: 1 out]
                        n206 = global read "全局 数据数组大小.vi" "数据数组大小"() -> (w250:i32)
                        n207 = global read "全局 小时数据发送次数.vi" "小时数据发送次数"() -> (w254:i32)
                        n208 = Greater Or Equal?(x=w254, y=w250) -> (x >= y?=w253:bool)
                        n209 = Compound Arithmetic op=OR ("复合运算")(w253) -> (w252:bool)
                      }
                    }
                  }
                }
                frame "跨度核查" {
                  n210 = flat-sequence {
                    frame #0 {
                      n211 = global write "全局 小时数据发送次数.vi" "小时数据发送次数"(0 ("小时数据发送次数")) -> ()
                      n212 = global write "全局 实时数据参数.vi" "实时数据参数"("跨度核查") -> ()
                      n213 = global write "全局1.vi" "枚举"(enum16{"返回请求应答", "上传数据", "返回执行结果"}."上传数据" ("枚举")) -> ()
                    }
                    frame #1 {
                      n214 = call "从数据库获取数据通用可配置(子VI).vi"("table输入"="实时数据" ("新元素/子数组"), "列队名（唯一）"="c") -> ()  [unwired: 8 in, 2 out]
                    }
                    frame #2 {
                      n215 = for {
                        N: 5 -> [_]
                        i -> [w280]
                        # "行数大于零"
                        n216 = case shown="3" w280 {
                          tunnel: [w285 w286 w287 w288 w289] -> w281
                          frame 0, Default {
                            n217 = global read "全局 所有参数.vi" "氨氮"() -> (w285:string[][])
                          }
                          frame 1 {
                            n218 = global read "全局 所有参数.vi" "总氮"() -> (w286:string[][])
                          }
                          frame 2 {
                            n219 = global read "全局 所有参数.vi" "总磷"() -> (w287:string[][])
                          }
                          frame 3 {
                            n220 = global read "全局 所有参数.vi" "CODMn"() -> (w288:string[][])
                          }
                          frame 4 {
                            n221 = global read "全局 所有参数.vi" "CODCr"() -> (w289:string[][])
                          }
                        }
                        n222 = Array Size(array=w281) -> (size(s)=w283:i32[])
                        n223 = Index Array(array=w283) -> (element=w282:i32)  [unwired: 1 in]
                        n224 = Greater Than 0?(x=w282) -> (x > 0?=w284:bool)
                        n225 = case shown="真" w284 {
                          tunnel: w280 -> [_ w295]
                          tunnel: w282 -> [_ _]
                          tunnel: w281 -> [_ w293]
                          frame False {
                          }
                          frame True {
                            # "最新时间戳加1分钟"
                            n226 = Index Array(array=w293, index (row)=0 ("禁用的索引 (行)"), index (col)=0 ("禁用的索引 (列)")) -> (element=w292:string)
                            n227 = call "日期时间字符串转换分钟数加一.vi"("data[0]"=w292) -> ("日期/时间字符串"=w291:string)  [unwired: 10 in]
                            n228 = case shown="3" w295 {
                              tunnel: w291 -> [w296 w297 w298 w299 w300]
                              frame 0, Default {
                                n229 = global write "全局 时间2.vi" "氨氮跨度核查索引起始时间"(w296) -> ()
                              }
                              frame 1 {
                                n230 = global write "全局 时间2.vi" "总氮跨度核查索引起始时间"(w297) -> ()
                              }
                              frame 2 {
                                n231 = global write "全局 时间2.vi" "总磷跨度核查索引起始时间"(w298) -> ()
                              }
                              frame 3 {
                                n232 = global write "全局 时间2.vi" "CODMn跨度核查索引起始时间"(w299) -> ()
                              }
                              frame 4 {
                                n233 = global write "全局 时间2.vi" "CODCr跨度核查索引起始时间"(w300) -> ()
                              }
                            }
                          }
                        }
                      }
                    }
                    frame #3 {
                      n234 = call <vilib>:"Application Directory.vi"() -> ("Application Directory"=w314:path)
                      n235 = call "数据处理整合 (子VI).vi"("枚举"=enum16{"实时数据排序", "小时数据排序"}."实时数据排序") -> ("已排序的数组"=w317:string[])  [unwired: 10 in]
                      n236 = Build Path(base path=w314, name or relative path="data\\hecha.ini" ("名称或相对路径")) -> (appended path=w312:path)
                      n237 = call <vilib>:"Open Config Data.vi"("configuration file path"=w312) -> ("error out"=w308:errorcluster, "refnum"=w311:T8)  [unwired: 8 in, 1 out]
                      n238 = Array Size(array=w317) -> (size(s)=w316:i32)
                      n239 = vi-ref "全局 时间2.vi"() -> (w310:refnum<vi>)
                      n240 = global write "全局 数据数组大小.vi" "数据数组大小"(w316) -> ()
                      n241 = call <userlib>:"Write Panel to INI__ogtk.vi"("error in (no error)"=w308, "VI ref"=w310, "refnum"=w311) -> ("error out"=w307:errorcluster, "refnum out"=w309:T8)  [unwired: 7 in]
                      n242 = call <vilib>:"Close Config Data.vi"("error in (no error)"=w307, "refnum"=w309) -> ("error out"=w302:errorcluster, "file path"=w301:path)  [unwired: 8 in]
                      n243 = Open/Create/Replace File(file path (use dialog)=w301, error in=w302) -> (refnum out=w305:refnum<file>, error out=w306:errorcluster)  [unwired: 4 in, 1 out]
                      n244 = Flush File(refnum=w305, error in=w306) -> (refnum out=w304:refnum<file>, error out=w303:errorcluster)
                      n245 = Close File(refnum=w304, error in=w303) -> ()  [unwired: 2 out]
                    }
                    frame #4 {
                      n246 = while {
                        stop <- w320 stop-if-true
                        n247 = property on="TCP服务端掉线计数" class="DigNum (严格)"() -> ("Value"=w324:i32)  [unwired: 2 in, 2 out]
                        n248 = property on="TCP服务端掉线计数" class="DigNum (严格)" props=["Value"]() -> ()  [unwired: 2 in, 3 out]
                        n249 = Greater Or Equal?(x=w324, y=1) -> (x >= y?=w323:bool)
                        n250 = case shown="假" w323 {
                          frame False {
                            n251 = global read "全局 数据数组大小.vi" "数据数组大小"() -> (w327:i32)
                            n252 = Greater Than 0?(x=w327) -> (x > 0?=w326:bool)
                            n253 = case shown="真" w326 {
                              frame False {
                              }
                              frame True {
                                w328 = 0 ("禁用的索引 (列)")
                                n254 = global read "插值后的新数组.vi" "插值后的数组元素"() -> (w338:T10)
                                n255 = local read "QN"() -> (w341:string)
                                n256 = local read "MN"() -> (w334:string)
                                n257 = local read "PW"() -> (w333:string)
                                n258 = local read "数据发送通道"() -> (w332:enum16{"TCP", "VISA"})
                                n259 = Unbundle By Name(w338) -> ("氨氮"=w337:string[][])
                                n260 = call "数据编码.vi"("table输入"="实时数据" ("新元素/子数组"), "QN"=w341, "MN"=w334, "PW"=w333) -> ("通讯包字符串"=w330:string)  [unwired: 10 in, 1 out]
                                n261 = local write "发送报文显示"(w330) -> ()
                                n262 = Index Array(array=w337, index (row)=w328, index (col)=w328) -> (element=w336:string)
                                n263 = call "VISATCP组合选择发送.vi"("数据发送通道"=w332, "命令"="write", "写入缓冲区"=w330) -> ("错误输出"=w329:errorcluster)  [unwired: 9 in, 3 out]
                                n264 = Build Array(w330) -> (w340:string[])
                                n265 = local write "核查数据上传"(TRUE ("数据上传")) -> ()
                                n266 = call "日期时间字符串转换分钟数加一.vi"("data[0]"=w336) -> ("日期/时间字符串"=w335:string)  [unwired: 10 in]
                                n267 = local write "错误输出"(w329) -> ()
                                n268 = call "发送数据记录到文档(子VI).vi"("数组"=w340) -> ()  [unwired: 9 in, 1 out]
                                n269 = global write "全局 时间2.vi" "跨度核查索引起始时间"(w335) -> ()
                              }
                            }
                          }
                          frame True {
                          }
                        }
                        n270 = Wait (ms)(milliseconds to wait=u32 500 ("等待时间（毫秒）")) -> ()  [unwired: 1 out]
                        n271 = global read "全局 数据数组大小.vi" "数据数组大小"() -> (w318:i32)
                        n272 = global read "全局 小时数据发送次数.vi" "小时数据发送次数"() -> (w322:i32)
                        n273 = Greater Or Equal?(x=w322, y=w318) -> (x >= y?=w321:bool)
                        n274 = Compound Arithmetic op=OR ("复合运算")(w321) -> (w320:bool)
                      }
                    }
                  }
                }
                frame "标样核查" {
                  n275 = flat-sequence {
                    tunnel: [w352] -> w343
                    frame #0 {
                      n276 = global write "全局 小时数据发送次数.vi" "小时数据发送次数"(0 ("小时数据发送次数")) -> ()
                      n277 = global write "全局 实时数据参数.vi" "实时数据参数"("核查数据") -> ()
                      n278 = global write "全局1.vi" "枚举"(enum16{"返回请求应答", "上传数据", "返回执行结果"}."上传数据" ("枚举")) -> ()
                    }
                    frame #1 {
                      n279 = call "从数据库获取数据通用可配置(子VI).vi"("table输入"="实时数据" ("新元素/子数组"), "列队名（唯一）"="n") -> ()  [unwired: 8 in, 2 out]
                    }
                    frame #2 {
                      n280 = call "数据处理整合 (子VI).vi"("枚举"=enum16{"实时数据排序", "小时数据排序"}."实时数据排序") -> ("已排序的数组"=w351:string[])  [unwired: 10 in]
                      n281 = Array Size(array=w351) -> (size(s)=w350:i32)
                      n282 = global write "全局 数据数组大小.vi" "数据数组大小"(w350) -> ()
                    }
                    frame #3 {
                      n283 = while {
                        tunnel: [w353] -> w352
                        stop <- w353 stop-if-true
                        n284 = property on="TCP服务端掉线计数" class="DigNum (严格)"() -> ("Value"=w359:i32)  [unwired: 2 in, 2 out]
                        n285 = property on="TCP服务端掉线计数" class="DigNum (严格)" props=["Value"]() -> ()  [unwired: 2 in, 3 out]
                        n286 = Greater Or Equal?(x=w359, y=1) -> (x >= y?=w358:bool)
                        n287 = case shown="假" w358 {
                          frame False {
                            n288 = global read "全局 数据数组大小.vi" "数据数组大小"() -> (w362:i32)
                            n289 = Greater Than 0?(x=w362) -> (x > 0?=w361:bool)
                            n290 = case shown="真" w361 {
                              frame False {
                              }
                              frame True {
                                w363 = 0 ("禁用的索引 (列)")
                                n291 = global read "插值后的新数组.vi" "插值后的数组元素"() -> (w373:T10)
                                n292 = local read "QN"() -> (w376:string)
                                n293 = local read "MN"() -> (w369:string)
                                n294 = local read "PW"() -> (w368:string)
                                n295 = local read "数据发送通道"() -> (w367:enum16{"TCP", "VISA"})
                                n296 = Unbundle By Name(w373) -> ("氨氮"=w372:string[][])
                                n297 = call "数据编码.vi"("table输入"="实时数据" ("新元素/子数组"), "QN"=w376, "MN"=w369, "PW"=w368) -> ("通讯包字符串"=w365:string)  [unwired: 10 in, 1 out]
                                n298 = local write "发送报文显示"(w365) -> ()
                                n299 = call "VISATCP组合选择发送.vi"("数据发送通道"=w367, "命令"="write", "写入缓冲区"=w365) -> ("错误输出"=w364:errorcluster)  [unwired: 9 in, 3 out]
                                n300 = Index Array(array=w372, index (row)=w363, index (col)=w363) -> (element=w371:string)
                                n301 = Build Array(w365) -> (w375:string[])
                                n302 = local write "核查数据上传"(TRUE ("数据上传")) -> ()
                                n303 = call "日期时间字符串转换分钟数加一.vi"("data[0]"=w371) -> ("日期/时间字符串"=w370:string)  [unwired: 10 in]
                                n304 = local write "错误输出"(w364) -> ()
                                n305 = call "发送数据记录到文档(子VI).vi"("数组"=w375) -> ()  [unwired: 9 in, 1 out]
                                n306 = global write "全局 时间2.vi" "标样核查索引起始时间"(w370) -> ()
                              }
                            }
                          }
                          frame True {
                          }
                        }
                        n307 = Wait (ms)(milliseconds to wait=u32 500 ("等待时间（毫秒）")) -> ()  [unwired: 1 out]
                        n308 = global read "全局 数据数组大小.vi" "数据数组大小"() -> (w354:i32)
                        n309 = global read "全局 小时数据发送次数.vi" "小时数据发送次数"() -> (w357:i32)
                        n310 = Greater Or Equal?(x=w357, y=w354) -> (x >= y?=w356:bool)
                        n311 = Compound Arithmetic op=OR ("复合运算")(w356) -> (w353:bool)
                      }
                    }
                  }
                }
                frame "加标回收" {
                  n312 = flat-sequence {
                    frame #0 {
                      n313 = global write "全局 小时数据发送次数.vi" "小时数据发送次数"(0 ("小时数据发送次数")) -> ()
                      n314 = global write "全局 实时数据参数.vi" "实时数据参数"("加标回收测试") -> ()
                      n315 = global write "全局1.vi" "枚举"(enum16{"返回请求应答", "上传数据", "返回执行结果"}."上传数据" ("枚举")) -> ()
                    }
                    frame #1 {
                      n316 = call "从数据库获取数据通用可配置(子VI).vi"("table输入"="加标回收" ("新元素/子数组"), "列队名（唯一）"="d") -> ()  [unwired: 8 in, 2 out]
                    }
                    frame #2 {
                      n317 = call "加标回收数据处理整合 (子VI).vi"("枚举"=enum16{"实时数据排序", "小时数据排序"}."实时数据排序") -> ("已排序的数组"=w384:string[])  [unwired: 10 in]
                      n318 = Array Size(array=w384) -> (size(s)=w385:i32)
                      n319 = global write "全局 数据数组大小.vi" "数据数组大小"(w385) -> ()
                    }
                    frame #3 {
                      n320 = while {
                        stop <- w388 stop-if-true
                        n321 = property on="TCP服务端掉线计数" class="DigNum (严格)"() -> ("Value"=w393:i32)  [unwired: 2 in, 2 out]
                        n322 = Greater Or Equal?(x=w393, y=1) -> (x >= y?=w391:bool)
                        n323 = case shown="假" w391 {
                          frame False {
                            n324 = global read "全局 数据数组大小.vi" "数据数组大小"() -> (w395:i32)
                            n325 = Greater Than 0?(x=w395) -> (x > 0?=w394:bool)
                            n326 = case shown="真" w394 {
                              frame False {
                              }
                              frame True {
                                n327 = global read "全局 数据数组大小.vi" "数据数组大小"() -> (w405:i32)
                                n328 = global read "插值后的新数组.vi" "插值后的数组元素"() -> (w408:T10)
                                n329 = local read "MN"() -> (w401:string)
                                n330 = local read "PW"() -> (w400:string)
                                n331 = local read "数据发送通道"() -> (w399:enum16{"TCP", "VISA"})
                                n332 = Decrement(x=w405) -> (x-1=w404:i32)
                                n333 = call "数据编码.vi"("table输入"="实时数据" ("新元素/子数组"), "MN"=w401, "PW"=w400) -> ("通讯包字符串"=w397:string)  [unwired: 11 in, 1 out]
                                n334 = Unbundle By Name(w408) -> ("氨氮"=w407:string[][])
                                n335 = local write "发送报文显示"(w397) -> ()
                                n336 = call "VISATCP组合选择发送.vi"("数据发送通道"=w399, "命令"="write", "写入缓冲区"=w397) -> ("错误输出"=w396:errorcluster)  [unwired: 9 in, 3 out]
                                n337 = Index Array(array=w407, index (row)=w404, index (col)=0 ("禁用的索引 (列)")) -> (element=w403:string)
                                n338 = local write "核查数据上传"(TRUE ("数据上传")) -> ()
                                n339 = Build Array(w397) -> (w410:string[])
                                n340 = call "日期时间字符串转换分钟数加一.vi"("data[0]"=w403) -> ("日期/时间字符串"=w402:string)  [unwired: 10 in]
                                n341 = local write "错误输出"(w396) -> ()
                                n342 = call "发送数据记录到文档(子VI).vi"("数组"=w410) -> ()  [unwired: 9 in, 1 out]
                                n343 = global write "全局 时间2.vi" "加标回收索引起始时间"(w402) -> ()
                              }
                            }
                          }
                          frame True {
                          }
                        }
                        n344 = Wait (ms)(milliseconds to wait=u32 500 ("等待时间（毫秒）")) -> ()  [unwired: 1 out]
                        n345 = global read "全局 数据数组大小.vi" "数据数组大小"() -> (w386:i32)
                        n346 = global read "全局 小时数据发送次数.vi" "小时数据发送次数"() -> (w390:i32)
                        n347 = Greater Or Equal?(x=w390, y=w386) -> (x >= y?=w389:bool)
                        n348 = Compound Arithmetic op=OR ("复合运算")(w389) -> (w388:bool)
                      }
                    }
                  }
                }
                frame "平行样" {
                  n349 = flat-sequence {
                    frame #0 {
                      n350 = global write "全局 小时数据发送次数.vi" "小时数据发送次数"(0 ("小时数据发送次数")) -> ()
                      n351 = global write "全局 实时数据参数.vi" "实时数据参数"("平行样测试") -> ()
                      n352 = global write "全局1.vi" "枚举"(enum16{"返回请求应答", "上传数据", "返回执行结果"}."上传数据" ("枚举")) -> ()
                    }
                    frame #1 {
                      n353 = call "从数据库获取数据通用可配置(子VI).vi"("table输入"="平行样测试" ("新元素/子数组"), "列队名（唯一）"="e") -> ()  [unwired: 8 in, 2 out]
                    }
                    frame #2 {
                      n354 = for {
                        N: 5 -> [_]
                        i -> [w418]
                        # "行数大于零"
                        n355 = case shown="3" w418 {
                          tunnel: [w423 w424 w425 w426 w427] -> w419
                          frame 0, Default {
                            n356 = global read "全局 所有参数.vi" "氨氮"() -> (w423:string[][])
                          }
                          frame 1 {
                            n357 = global read "全局 所有参数.vi" "总氮"() -> (w424:string[][])
                          }
                          frame 2 {
                            n358 = global read "全局 所有参数.vi" "总磷"() -> (w425:string[][])
                          }
                          frame 3 {
                            n359 = global read "全局 所有参数.vi" "CODMn"() -> (w426:string[][])
                          }
                          frame 4 {
                            n360 = global read "全局 所有参数.vi" "CODCr"() -> (w427:string[][])
                          }
                        }
                        n361 = Array Size(array=w419) -> (size(s)=w421:i32[])
                        n362 = Index Array(array=w421) -> (element=w420:i32)  [unwired: 1 in]
                        n363 = Greater Than 0?(x=w420) -> (x > 0?=w422:bool)
                        n364 = case shown="真" w422 {
                          tunnel: w418 -> [_ w433]
                          tunnel: w420 -> [_ _]
                          tunnel: w419 -> [_ w431]
                          frame False {
                          }
                          frame True {
                            # "最新时间戳加1分钟"
                            n365 = Index Array(array=w431, index (row)=0 ("禁用的索引 (行)"), index (col)=0 ("禁用的索引 (列)")) -> (element=w430:string)
                            n366 = call "日期时间字符串转换分钟数加一.vi"("data[0]"=w430) -> ("日期/时间字符串"=w429:string)  [unwired: 10 in]
                            n367 = case shown="0, 默认" w433 {
                              tunnel: w429 -> [w434 w435 w436 w437 w438]
                              frame 0, Default {
                                n368 = global write "全局 时间2.vi" "氨氮平行样索引起始时间"(w434) -> ()
                              }
                              frame 1 {
                                n369 = global write "全局 时间2.vi" "总氮平行样索引起始时间"(w435) -> ()
                              }
                              frame 2 {
                                n370 = global write "全局 时间2.vi" "总磷平行样索引起始时间"(w436) -> ()
                              }
                              frame 3 {
                                n371 = global write "全局 时间2.vi" "CODMn平行样索引起始时间"(w437) -> ()
                              }
                              frame 4 {
                                n372 = global write "全局 时间2.vi" "CODCr平行样索引起始时间"(w438) -> ()
                              }
                            }
                          }
                        }
                      }
                    }
                    frame #3 {
                      n373 = call "数据处理整合 (子VI).vi"("枚举"=enum16{"实时数据排序", "小时数据排序"}."实时数据排序") -> ("已排序的数组"=w455:string[])  [unwired: 10 in]
                      n374 = Array Size(array=w455) -> (size(s)=w454:i32)
                      n375 = call <vilib>:"Application Directory.vi"() -> ("Application Directory"=w452:path)
                      n376 = Build Path(base path=w452, name or relative path="data\\hecha.ini" ("名称或相对路径")) -> (appended path=w450:path)
                      n377 = global write "全局 数据数组大小.vi" "数据数组大小"(w454) -> ()
                      n378 = call <vilib>:"Open Config Data.vi"("configuration file path"=w450) -> ("error out"=w446:errorcluster, "refnum"=w449:T8)  [unwired: 8 in, 1 out]
                      n379 = vi-ref "全局 时间2.vi"() -> (w448:refnum<vi>)
                      n380 = call <userlib>:"Write Panel to INI__ogtk.vi"("error in (no error)"=w446, "VI ref"=w448, "refnum"=w449) -> ("error out"=w445:errorcluster, "refnum out"=w447:T8)  [unwired: 7 in]
                      n381 = call <vilib>:"Close Config Data.vi"("error in (no error)"=w445, "refnum"=w447) -> ("error out"=w440:errorcluster, "file path"=w439:path)  [unwired: 8 in]
                      n382 = Open/Create/Replace File(file path (use dialog)=w439, error in=w440) -> (refnum out=w443:refnum<file>, error out=w444:errorcluster)  [unwired: 4 in, 1 out]
                      n383 = Flush File(refnum=w443, error in=w444) -> (refnum out=w442:refnum<file>, error out=w441:errorcluster)
                      n384 = Close File(refnum=w442, error in=w441) -> ()  [unwired: 2 out]
                    }
                    frame #4 {
                      n385 = while {
                        stop <- w458 stop-if-true
                        n386 = property on="TCP服务端掉线计数" class="DigNum (严格)"() -> ("Value"=w464:i32)  [unwired: 2 in, 2 out]
                        n387 = property on="TCP服务端掉线计数" class="DigNum (严格)" props=["Value"]() -> ()  [unwired: 2 in, 3 out]
                        n388 = Greater Or Equal?(x=w464, y=1) -> (x >= y?=w462:bool)
                        n389 = case shown="假" w462 {
                          frame False {
                            n390 = global read "全局 数据数组大小.vi" "数据数组大小"() -> (w466:i32)
                            n391 = Greater Than 0?(x=w466) -> (x > 0?=w465:bool)
                            n392 = case shown="真" w465 {
                              frame False {
                              }
                              frame True {
                                n393 = local read "MN"() -> (w472:string)
                                n394 = local read "PW"() -> (w471:string)
                                n395 = local read "数据发送通道"() -> (w470:enum16{"TCP", "VISA"})
                                n396 = local write "核查数据上传"(TRUE ("数据上传")) -> ()
                                n397 = call "数据编码.vi"("table输入"="实时数据" ("新元素/子数组"), "MN"=w472, "PW"=w471) -> ("通讯包字符串"=w468:string)  [unwired: 11 in, 1 out]
                                n398 = local write "发送报文显示"(w468) -> ()
                                n399 = call "VISATCP组合选择发送.vi"("数据发送通道"=w470, "命令"="write", "写入缓冲区"=w468) -> ("错误输出"=w467:errorcluster)  [unwired: 9 in, 3 out]
                                n400 = Build Array(w468) -> (w474:string[])
                                n401 = call "发送数据记录到文档(子VI).vi"("数组"=w474) -> ()  [unwired: 9 in, 1 out]
                                n402 = local write "错误输出"(w467) -> ()
                              }
                            }
                          }
                          frame True {
                          }
                        }
                        n403 = Wait (ms)(milliseconds to wait=u32 500 ("等待时间（毫秒）")) -> ()  [unwired: 1 out]
                        n404 = global read "全局 数据数组大小.vi" "数据数组大小"() -> (w461:i32)
                        n405 = global read "全局 小时数据发送次数.vi" "小时数据发送次数"() -> (w460:i32)
                        n406 = Decrement(x=w461) -> (x-1=w457:i32)
                        n407 = Greater Or Equal?(x=w460, y=w457) -> (x >= y?=w459:bool)
                        n408 = Compound Arithmetic op=OR ("复合运算")(w459) -> (w458:bool)
                      }
                    }
                  }
                }
                frame "集成干预" {
                  n409 = flat-sequence {
                    frame #0 {
                      n410 = global write "全局 小时数据发送次数.vi" "小时数据发送次数"(0 ("小时数据发送次数")) -> ()
                      n411 = global write "全局 实时数据参数.vi" "实时数据参数"("集成干预测试") -> ()
                      n412 = global write "全局1.vi" "枚举"(enum16{"返回请求应答", "上传数据", "返回执行结果"}."上传数据" ("枚举")) -> ()
                    }
                    frame #1 {
                      n413 = call "从数据库获取数据通用可配置(子VI).vi"("table输入"="集成干预测试" ("新元素/子数组"), "列队名（唯一）"="f") -> ()  [unwired: 8 in, 2 out]
                    }
                    frame #2 {
                      n414 = for {
                        N: 10 -> [_]
                        i -> [w482]
                        # "行数大于零"
                        n415 = case shown="9" w482 {
                          tunnel: [w487 w488 w489 w490 w491 w492 w493 w494 w495 w496] -> w483
                          frame 0, Default {
                            n416 = global read "全局 所有参数.vi" "氨氮"() -> (w487:string[][])
                          }
                          frame 1 {
                            n417 = global read "全局 所有参数.vi" "总氮"() -> (w488:string[][])
                          }
                          frame 2 {
                            n418 = global read "全局 所有参数.vi" "总磷"() -> (w489:string[][])
                          }
                          frame 3 {
                            n419 = global read "全局 所有参数.vi" "CODMn"() -> (w490:string[][])
                          }
                          frame 4 {
                            n420 = global read "全局 所有参数.vi" "CODCr"() -> (w491:string[][])
                          }
                          frame 5 {
                            n421 = global read "全局 所有参数.vi" "DO"() -> (w492:string[][])
                          }
                          frame 6 {
                            n422 = global read "全局 所有参数.vi" "PH"() -> (w493:string[][])
                          }
                          frame 7 {
                            n423 = global read "全局 所有参数.vi" "电导率"() -> (w494:string[][])
                          }
                          frame 8 {
                            n424 = global read "全局 所有参数.vi" "水温"() -> (w495:string[][])
                          }
                          frame 9 {
                            n425 = global read "全局 所有参数.vi" "浊度"() -> (w496:string[][])
                          }
                        }
                        n426 = Array Size(array=w483) -> (size(s)=w485:i32[])
                        n427 = Index Array(array=w485) -> (element=w484:i32)  [unwired: 1 in]
                        n428 = Greater Than 0?(x=w484) -> (x > 0?=w486:bool)
                        n429 = case shown="真" w486 {
                          tunnel: w482 -> [_ w502]
                          tunnel: w484 -> [_ _]
                          tunnel: w483 -> [_ w500]
                          frame False {
                          }
                          frame True {
                            # "最新时间戳加1分钟"
                            n430 = Index Array(array=w500, index (row)=0 ("禁用的索引 (行)"), index (col)=0 ("禁用的索引 (列)")) -> (element=w499:string)
                            n431 = call "日期时间字符串转换分钟数加一.vi"("data[0]"=w499) -> ("日期/时间字符串"=w498:string)  [unwired: 10 in]
                            n432 = case shown="9" w502 {
                              tunnel: w498 -> [w503 w504 w505 w506 w507 w508 w509 w510 w511 w512]
                              frame 0, Default {
                                n433 = global write "全局 时间2.vi" "氨氮集成干预索引起始时间"(w503) -> ()
                              }
                              frame 1 {
                                n434 = global write "全局 时间2.vi" "总氮集成干预索引起始时间"(w504) -> ()
                              }
                              frame 2 {
                                n435 = global write "全局 时间2.vi" "总磷集成干预索引起始时间"(w505) -> ()
                              }
                              frame 3 {
                                n436 = global write "全局 时间2.vi" "CODMn集成干预索引起始时间"(w506) -> ()
                              }
                              frame 4 {
                                n437 = global write "全局 时间2.vi" "CODCr集成干预索引起始时间"(w507) -> ()
                              }
                              frame 5 {
                                n438 = global write "全局 时间2.vi" "DO集成干预索引起始时间"(w508) -> ()
                              }
                              frame 6 {
                                n439 = global write "全局 时间2.vi" "PH集成干预索引起始时间"(w509) -> ()
                              }
                              frame 7 {
                                n440 = global write "全局 时间2.vi" "比电导率集成干预索引起始时间"(w510) -> ()
                              }
                              frame 8 {
                                n441 = global write "全局 时间2.vi" "水温集成干预索引起始时间"(w511) -> ()
                              }
                              frame 9 {
                                n442 = global write "全局 时间2.vi" "浊度集成干预索引起始时间"(w512) -> ()
                              }
                            }
                          }
                        }
                      }
                    }
                    frame #3 {
                      n443 = call "数据处理整合 (子VI).vi"("枚举"=enum16{"实时数据排序", "小时数据排序"}."实时数据排序") -> ("已排序的数组"=w529:string[])  [unwired: 10 in]
                      n444 = Array Size(array=w529) -> (size(s)=w528:i32)
                      n445 = call <vilib>:"Application Directory.vi"() -> ("Application Directory"=w526:path)
                      n446 = Build Path(base path=w526, name or relative path="data\\hecha.ini" ("名称或相对路径")) -> (appended path=w524:path)
                      n447 = global write "全局 数据数组大小.vi" "数据数组大小"(w528) -> ()
                      n448 = call <vilib>:"Open Config Data.vi"("configuration file path"=w524) -> ("error out"=w520:errorcluster, "refnum"=w523:T8)  [unwired: 8 in, 1 out]
                      n449 = vi-ref "全局 时间2.vi"() -> (w522:refnum<vi>)
                      n450 = call <userlib>:"Write Panel to INI__ogtk.vi"("error in (no error)"=w520, "VI ref"=w522, "refnum"=w523) -> ("error out"=w519:errorcluster, "refnum out"=w521:T8)  [unwired: 7 in]
                      n451 = call <vilib>:"Close Config Data.vi"("error in (no error)"=w519, "refnum"=w521) -> ("error out"=w514:errorcluster, "file path"=w513:path)  [unwired: 8 in]
                      n452 = Open/Create/Replace File(file path (use dialog)=w513, error in=w514) -> (refnum out=w517:refnum<file>, error out=w518:errorcluster)  [unwired: 4 in, 1 out]
                      n453 = Flush File(refnum=w517, error in=w518) -> (refnum out=w516:refnum<file>, error out=w515:errorcluster)
                      n454 = Close File(refnum=w516, error in=w515) -> ()  [unwired: 2 out]
                    }
                    frame #4 {
                      n455 = while {
                        stop <- w532 stop-if-true
                        n456 = property on="TCP服务端掉线计数" class="DigNum (严格)"() -> ("Value"=w538:i32)  [unwired: 2 in, 2 out]
                        n457 = property on="TCP服务端掉线计数" class="DigNum (严格)" props=["Value"]() -> ()  [unwired: 2 in, 3 out]
                        n458 = Greater Or Equal?(x=w538, y=1) -> (x >= y?=w536:bool)
                        n459 = case shown="假" w536 {
                          frame False {
                            n460 = global read "全局 数据数组大小.vi" "数据数组大小"() -> (w540:i32)
                            n461 = Greater Than 0?(x=w540) -> (x > 0?=w539:bool)
                            n462 = case shown="真" w539 {
                              frame False {
                              }
                              frame True {
                                n463 = local read "MN"() -> (w546:string)
                                n464 = local read "PW"() -> (w545:string)
                                n465 = local read "数据发送通道"() -> (w544:enum16{"TCP", "VISA"})
                                n466 = local write "核查数据上传"(TRUE ("数据上传")) -> ()
                                n467 = call "数据编码.vi"("table输入"="实时数据" ("新元素/子数组"), "MN"=w546, "PW"=w545) -> ("通讯包字符串"=w542:string)  [unwired: 11 in, 1 out]
                                n468 = local write "发送报文显示"(w542) -> ()
                                n469 = call "VISATCP组合选择发送.vi"("数据发送通道"=w544, "命令"="write", "写入缓冲区"=w542) -> ("错误输出"=w541:errorcluster)  [unwired: 9 in, 3 out]
                                n470 = Build Array(w542) -> (w548:string[])
                                n471 = call "发送数据记录到文档(子VI).vi"("数组"=w548) -> ()  [unwired: 9 in, 1 out]
                                n472 = local write "错误输出"(w541) -> ()
                              }
                            }
                          }
                          frame True {
                          }
                        }
                        n473 = Wait (ms)(milliseconds to wait=u32 500 ("等待时间（毫秒）")) -> ()  [unwired: 1 out]
                        n474 = global read "全局 数据数组大小.vi" "数据数组大小"() -> (w535:i32)
                        n475 = global read "全局 小时数据发送次数.vi" "小时数据发送次数"() -> (w534:i32)
                        n476 = Decrement(x=w535) -> (x-1=w531:i32)
                        n477 = Greater Or Equal?(x=w534, y=w531) -> (x >= y?=w533:bool)
                        n478 = Compound Arithmetic op=OR ("复合运算")(w533) -> (w532:bool)
                      }
                    }
                  }
                }
                frame "", Default {
                  n479 = Get Queue Status(queue=w553) -> (# elements in queue=w552:i32)  [unwired: 2 in, 7 out]
                  n480 = Equal To 0?(x=w552) -> (x = 0?=w551:bool)
                  n481 = case shown="真" w551 {
                    tunnel: [_ TRUE] -> w550
                    frame False {
                    }
                    frame True {
                    }
                  }
                }
              }
              n482 = Wait (ms)(milliseconds to wait=u32 1000 ("等待时间（毫秒）")) -> ()  [unwired: 1 out]
            }
          }
          frame "小时数据" {
            # "间隔时间上传"
            n483 = flat-sequence {
              frame #0 {
                # "发送前2小时的数据"
                n484 = global write "全局 小时数据发送次数.vi" "小时数据发送次数"(1 ("小时数据发送次数")) -> ()
                n485 = global write "全局1.vi" "枚举"(enum16{"返回请求应答", "上传数据", "返回执行结果"}."上传数据" ("枚举")) -> ()
              }
              frame #1 {
                n486 = call "从数据库获取数据通用可配置(子VI).vi"("table输入"="小时数据" ("新元素/子数组"), "列队名（唯一）"="XS" ("名称（未命名）")) -> ()  [unwired: 8 in, 2 out]
              }
              frame #2 {
                n487 = property on="TCP服务端掉线计数" class="DigNum (严格)"() -> ("Value"=w560:i32)  [unwired: 2 in, 2 out]
                n488 = Greater Or Equal?(x=w560, y=1) -> (x >= y?=w559:bool)
                n489 = case shown="假" w559 {
                  frame False {
                    # "数据处理整合"
                    n490 = call "实时小时数据处理整合 (子VI).vi"("枚举"=enum16{"实时数据排序", "小时数据排序"}."小时数据排序") -> ("已排序的数组"=w562:string[])  [unwired: 10 in]
                    n491 = Array Size(array=w562) -> (size(s)=w565:i32)
                    n492 = global write "全局 数据数组大小.vi" "数据数组大小"(1 ("数据数组大小")) -> ()
                    n493 = Greater Than 0?(x=w565) -> (x > 0?=w566:bool)
                    n494 = case shown="真" w566 {
                      frame False {
                      }
                      frame True {
                        n495 = local write "核查数据上传"(TRUE ("数据上传")) -> ()
                        n496 = Get Date/Time In Seconds() -> (seconds since 1Jan1904=w577:timestamp)
                        n497 = Format Date/Time String(time format string (%c)="%Y%m%d%H%M%S%3u" ("时间格式字符串(%c)"), seconds (now)=w577) -> (date/time string=w578:string)  [unwired: 1 in]
                        n498 = local read "MN"() -> (w572:string)
                        n499 = local read "PW"() -> (w571:string)
                        n500 = Search and Replace String(input string=w578, search string="." ("搜索字符串")) -> (result string=w580:string)  [unwired: 6 in, 3 out]
                        n501 = local read "数据发送通道"() -> (w570:enum16{"TCP", "VISA"})
                        n502 = call "数据编码.vi"("table输入"="小时数据" ("新元素/子数组"), "QN"=w580, "MN"=w572, "PW"=w571) -> ("通讯包字符串"=w568:string)  [unwired: 10 in, 1 out]
                        n503 = local write "发送报文显示"(w568) -> ()
                        n504 = call "VISATCP组合选择发送.vi"("数据发送通道"=w570, "命令"="write", "写入缓冲区"=w568) -> ("错误输出"=w567:errorcluster)  [unwired: 9 in, 3 out]
                        n505 = Build Array(w568) -> (w574:string[])
                        n506 = local write "错误输出"(w567) -> ()
                        n507 = call "发送数据记录到文档(子VI).vi"("数组"=w574) -> ()  [unwired: 9 in, 1 out]
                      }
                    }
                  }
                  frame True {
                  }
                }
              }
            }
          }
          frame "操作日志" {
            # "间隔时间上传"
            # "直接1分钟查询 一次,有数据就按数据上传,没数据就不上传,在数据发送那边有做处理"
            n508 = flat-sequence {
              frame #0 {
                # "时间"
                n509 = global read "全局 数据发送重叠.vi" "数据发送重叠开始时间戳"() -> (w582:string)
                n510 = global read "全局 数据发送重叠.vi" "数据发送重叠"() -> (w581:bool)
                n511 = global write "全局 小时数据发送次数.vi" "小时数据发送次数"(0 ("小时数据发送次数")) -> ()
                n512 = global write "全局1.vi" "枚举"(enum16{"返回请求应答", "上传数据", "返回执行结果"}."上传数据" ("枚举")) -> ()
                n513 = call "日志信息主动发送(子VI).vi"("是否正在查询数据"=w581, "查询数据发送时间节点"=w582) -> ()  [unwired: 10 in]
              }
              frame #1 {
                n514 = call "获取操作日志 (子VI).vi"("table输入"="操作日志") -> ()  [unwired: 11 in]
              }
              frame #2 {
                n515 = call "数据处理整合 (子VI).vi"("枚举"=enum16{"实时数据排序", "小时数据排序"}."实时数据排序") -> ("已排序的数组"=w588:string[])  [unwired: 10 in]
                n516 = Array Size(array=w588) -> (size(s)=w587:i32)
                n517 = global write "全局 数据数组大小.vi" "数据数组大小"(w587) -> ()
              }
              frame #3 {
                n518 = while {
                  stop <- w589 stop-if-true
                  # "判定是否存表"
                  n519 = property on="TCP服务端掉线计数" class="DigNum (严格)"() -> ("Value"=w595:i32)  [unwired: 2 in, 2 out]
                  n520 = Greater Or Equal?(x=w595, y=1) -> (x >= y?=w594:bool)
                  n521 = case shown="假" w594 {
                    frame False {
                      n522 = global read "全局 数据数组大小.vi" "数据数组大小"() -> (w597:i32)
                      n523 = Greater Than 0?(x=w597) -> (x > 0?=w598:bool)
                      n524 = case shown="真" w598 {
                        frame False {
                        }
                        frame True {
                          n525 = global read "全局 小时数据发送次数.vi" "小时数据发送次数"() -> (w607:i32)
                          n526 = local write "核查数据上传"(TRUE ("数据上传")) -> ()
                          n527 = Get Date/Time In Seconds() -> (seconds since 1Jan1904=w612:timestamp)
                          n528 = Increment(x=w607) -> (x+1=w606:i32)
                          n529 = Format Date/Time String(time format string (%c)="%Y%m%d%H%M%S%3u" ("时间格式字符串(%c)"), seconds (now)=w612) -> (date/time string=w611:string)  [unwired: 1 in]
                          n530 = global write "全局 小时数据发送次数.vi" "小时数据发送次数"(w606) -> ()
                          n531 = Search and Replace String(input string=w611, search string="." ("搜索字符串")) -> (result string=w609:string)  [unwired: 6 in, 3 out]
                          n532 = local read "MN"() -> (w604:string)
                          n533 = local read "PW"() -> (w603:string)
                          n534 = call "数据编码.vi"("table输入"="操作日志" ("新元素/子数组"), "QN"=w609, "MN"=w604, "PW"=w603) -> ("通讯包字符串"=w600:string)  [unwired: 10 in, 1 out]
                          n535 = local read "数据发送通道"() -> (w602:enum16{"TCP", "VISA"})
                          n536 = local write "发送报文显示"(w600) -> ()
                          n537 = call "VISATCP组合选择发送.vi"("数据发送通道"=w602, "命令"="write", "写入缓冲区"=w600) -> ("错误输出"=w599:errorcluster)  [unwired: 9 in, 3 out]
                          n538 = Build Array(w600) -> (w608:string[])
                          n539 = local write "错误输出"(w599) -> ()
                          n540 = call "发送数据记录到文档(子VI).vi"("数组"=w608) -> ()  [unwired: 9 in, 1 out]
                        }
                      }
                    }
                    frame True {
                    }
                  }
                  n541 = Wait (ms)(milliseconds to wait=u32 500 ("等待时间（毫秒）")) -> ()  [unwired: 1 out]
                  n542 = global read "全局 数据数组大小.vi" "数据数组大小"() -> (w591:i32)
                  n543 = global read "全局 小时数据发送次数.vi" "小时数据发送次数"() -> (w593:i32)
                  n544 = Decrement(x=w591) -> (x-1=w590:i32)
                  n545 = Greater Or Equal?(x=w593, y=w590) -> (x >= y?=w589:bool)
                }
              }
            }
          }
          frame "仪器参数" {
            # "间隔时间上传"
            # "直接1分钟查询 一次,有数据就按数据上传,没数据就不上传,在数据发送那边有做处理"
            n546 = flat-sequence {
              frame #0 {
                # "时间"
                n547 = global read "全局 数据发送重叠.vi" "数据发送重叠开始时间戳"() -> (w616:string)
                n548 = global read "全局 数据发送重叠.vi" "数据发送重叠"() -> (w615:bool)
                n549 = global write "全局 小时数据发送次数.vi" "小时数据发送次数"(0 ("小时数据发送次数")) -> ()
                n550 = global write "全局1.vi" "枚举"(enum16{"返回请求应答", "上传数据", "返回执行结果"}."上传数据" ("枚举")) -> ()
                n551 = call "日志信息主动发送(子VI).vi"("是否正在查询数据"=w615, "查询数据发送时间节点"=w616) -> ()  [unwired: 10 in]
              }
              frame #1 {
                n552 = call "获取操作日志 (子VI).vi"("table输入"="仪器参数") -> ()  [unwired: 11 in]
              }
              frame #2 {
                n553 = call "数据处理整合 (子VI).vi"("枚举"=enum16{"实时数据排序", "小时数据排序"}."实时数据排序") -> ("已排序的数组"=w622:string[])  [unwired: 10 in]
                n554 = Array Size(array=w622) -> (size(s)=w621:i32)
                n555 = global write "全局 数据数组大小.vi" "数据数组大小"(w621) -> ()
              }
              frame #3 {
                n556 = while {
                  stop <- w623 stop-if-true
                  # "判定是否存表"
                  n557 = property on="TCP服务端掉线计数" class="DigNum (严格)"() -> ("Value"=w629:i32)  [unwired: 2 in, 2 out]
                  n558 = Greater Or Equal?(x=w629, y=1) -> (x >= y?=w628:bool)
                  n559 = case shown="假" w628 {
                    frame False {
                      n560 = global read "全局 数据数组大小.vi" "数据数组大小"() -> (w631:i32)
                      n561 = Greater Than 0?(x=w631) -> (x > 0?=w632:bool)
                      n562 = case shown="真" w632 {
                        frame False {
                        }
                        frame True {
                          n563 = global read "全局 小时数据发送次数.vi" "小时数据发送次数"() -> (w641:i32)
                          n564 = local write "核查数据上传"(TRUE ("数据上传")) -> ()
                          n565 = Get Date/Time In Seconds() -> (seconds since 1Jan1904=w646:timestamp)
                          n566 = Increment(x=w641) -> (x+1=w640:i32)
                          n567 = Format Date/Time String(time format string (%c)="%Y%m%d%H%M%S%3u" ("时间格式字符串(%c)"), seconds (now)=w646) -> (date/time string=w645:string)  [unwired: 1 in]
                          n568 = global write "全局 小时数据发送次数.vi" "小时数据发送次数"(w640) -> ()
                          n569 = Search and Replace String(input string=w645, search string="." ("搜索字符串")) -> (result string=w643:string)  [unwired: 6 in, 3 out]
                          n570 = local read "MN"() -> (w638:string)
                          n571 = local read "PW"() -> (w637:string)
                          n572 = call "数据编码.vi"("table输入"="仪器参数" ("新元素/子数组"), "QN"=w643, "MN"=w638, "PW"=w637) -> ("通讯包字符串"=w634:string)  [unwired: 10 in, 1 out]
                          n573 = local read "数据发送通道"() -> (w636:enum16{"TCP", "VISA"})
                          n574 = local write "发送报文显示"(w634) -> ()
                          n575 = call "VISATCP组合选择发送.vi"("数据发送通道"=w636, "命令"="write", "写入缓冲区"=w634) -> ("错误输出"=w633:errorcluster)  [unwired: 9 in, 3 out]
                          n576 = Build Array(w634) -> (w642:string[])
                          n577 = local write "错误输出"(w633) -> ()
                          n578 = call "发送数据记录到文档(子VI).vi"("数组"=w642) -> ()  [unwired: 9 in, 1 out]
                        }
                      }
                    }
                    frame True {
                    }
                  }
                  n579 = Wait (ms)(milliseconds to wait=u32 500 ("等待时间（毫秒）")) -> ()  [unwired: 1 out]
                  n580 = global read "全局 数据数组大小.vi" "数据数组大小"() -> (w625:i32)
                  n581 = global read "全局 小时数据发送次数.vi" "小时数据发送次数"() -> (w627:i32)
                  n582 = Decrement(x=w625) -> (x-1=w624:i32)
                  n583 = Greater Or Equal?(x=w627, y=w624) -> (x >= y?=w623:bool)
                }
              }
            }
          }
          frame "系统状态" {
            # "直接1分钟查询 一次,有变化就按上传,没变化就不上传"
            n584 = flat-sequence {
              frame #0 {
                # "时间"
                n585 = global write "全局 小时数据发送次数.vi" "小时数据发送次数"(0 ("小时数据发送次数")) -> ()
                n586 = global write "全局 数据数组大小.vi" "数据数组大小"(1 ("数据数组大小")) -> ()
                n587 = global write "全局1.vi" "枚举"(enum16{"返回请求应答", "上传数据", "返回执行结果"}."上传数据" ("枚举")) -> ()
              }
              frame #1 {
                # "判定是否存表"
                n588 = property on="TCP服务端掉线计数" class="DigNum (严格)"() -> ("Value"=w653:i32)  [unwired: 2 in, 2 out]
                n589 = Greater Or Equal?(x=w653, y=1) -> (x >= y?=w652:bool)
                n590 = case shown="假" w652 {
                  frame False {
                    n591 = global read "全局 数据数组大小.vi" "数据数组大小"() -> (w655:i32)
                    n592 = Greater Than 0?(x=w655) -> (x > 0?=w656:bool)
                    n593 = case shown="真" w656 {
                      frame False {
                      }
                      frame True {
                        n594 = global read "全局 小时数据发送次数.vi" "小时数据发送次数"() -> (w665:i32)
                        n595 = local write "核查数据上传"(TRUE ("数据上传")) -> ()
                        n596 = Get Date/Time In Seconds() -> (seconds since 1Jan1904=w670:timestamp)
                        n597 = Increment(x=w665) -> (x+1=w664:i32)
                        n598 = Format Date/Time String(time format string (%c)="%Y%m%d%H%M%S%3u" ("时间格式字符串(%c)"), seconds (now)=w670) -> (date/time string=w669:string)  [unwired: 1 in]
                        n599 = global write "全局 小时数据发送次数.vi" "小时数据发送次数"(w664) -> ()
                        n600 = Search and Replace String(input string=w669, search string="." ("搜索字符串")) -> (result string=w667:string)  [unwired: 6 in, 3 out]
                        n601 = local read "MN"() -> (w662:string)
                        n602 = local read "PW"() -> (w661:string)
                        n603 = call "数据编码.vi"("table输入"="系统状态" ("新元素/子数组"), "QN"=w667, "MN"=w662, "PW"=w661) -> ("通讯包字符串"=w658:string)  [unwired: 10 in, 1 out]
                        n604 = local read "数据发送通道"() -> (w660:enum16{"TCP", "VISA"})
                        n605 = local write "发送报文显示"(w658) -> ()
                        n606 = call "VISATCP组合选择发送.vi"("数据发送通道"=w660, "命令"="write", "写入缓冲区"=w658) -> ("错误输出"=w657:errorcluster)  [unwired: 9 in, 3 out]
                        n607 = Build Array(w658) -> (w666:string[])
                        n608 = local write "错误输出"(w657) -> ()
                        n609 = call "发送数据记录到文档(子VI).vi"("数组"=w666) -> ()  [unwired: 9 in, 1 out]
                      }
                    }
                  }
                  frame True {
                  }
                }
              }
            }
          }
          frame "运行模式" {
            # "直接1分钟查询 一次,有变化就按上传,没变化就不上传"
            n610 = flat-sequence {
              frame #0 {
                # "时间"
                n611 = global write "全局 小时数据发送次数.vi" "小时数据发送次数"(0 ("小时数据发送次数")) -> ()
                n612 = global write "全局 数据数组大小.vi" "数据数组大小"(1 ("数据数组大小")) -> ()
                n613 = global write "全局1.vi" "枚举"(enum16{"返回请求应答", "上传数据", "返回执行结果"}."上传数据" ("枚举")) -> ()
              }
              frame #1 {
                # "判定是否存表"
                n614 = property on="TCP服务端掉线计数" class="DigNum (严格)"() -> ("Value"=w677:i32)  [unwired: 2 in, 2 out]
                n615 = Greater Or Equal?(x=w677, y=1) -> (x >= y?=w676:bool)
                n616 = case shown="假" w676 {
                  frame False {
                    n617 = global read "全局 数据数组大小.vi" "数据数组大小"() -> (w679:i32)
                    n618 = Greater Than 0?(x=w679) -> (x > 0?=w680:bool)
                    n619 = case shown="真" w680 {
                      frame False {
                      }
                      frame True {
                        n620 = global read "全局 小时数据发送次数.vi" "小时数据发送次数"() -> (w689:i32)
                        n621 = local write "核查数据上传"(TRUE ("数据上传")) -> ()
                        n622 = Get Date/Time In Seconds() -> (seconds since 1Jan1904=w694:timestamp)
                        n623 = Increment(x=w689) -> (x+1=w688:i32)
                        n624 = Format Date/Time String(time format string (%c)="%Y%m%d%H%M%S%3u" ("时间格式字符串(%c)"), seconds (now)=w694) -> (date/time string=w693:string)  [unwired: 1 in]
                        n625 = global write "全局 小时数据发送次数.vi" "小时数据发送次数"(w688) -> ()
                        n626 = Search and Replace String(input string=w693, search string="." ("搜索字符串")) -> (result string=w691:string)  [unwired: 6 in, 3 out]
                        n627 = local read "MN"() -> (w685:string)
                        n628 = local read "PW"() -> (w686:string)
                        n629 = local read "数据发送通道"() -> (w684:enum16{"TCP", "VISA"})
                        n630 = call "数据编码.vi"("table输入"="运行模式" ("新元素/子数组"), "QN"=w691, "MN"=w685, "PW"=w686) -> ("通讯包字符串"=w681:string)  [unwired: 10 in, 1 out]
                        n631 = local write "发送报文显示"(w681) -> ()
                        n632 = call "VISATCP组合选择发送.vi"("数据发送通道"=w684, "命令"="write", "写入缓冲区"=w681) -> ("错误输出"=w682:errorcluster)  [unwired: 9 in, 3 out]
                        n633 = Build Array(w681) -> (w690:string[])
                        n634 = local write "错误输出"(w682) -> ()
                        n635 = call "发送数据记录到文档(子VI).vi"("数组"=w690) -> ()  [unwired: 9 in, 1 out]
                      }
                    }
                  }
                  frame True {
                  }
                }
              }
            }
          }
          frame "测量周期" {
            # "直接1分钟查询 一次,有变化就按上传,没变化就不上传"
            n636 = flat-sequence {
              frame #0 {
                # "时间"
                n637 = global write "全局 小时数据发送次数.vi" "小时数据发送次数"(0 ("小时数据发送次数")) -> ()
                n638 = global write "全局 数据数组大小.vi" "数据数组大小"(1 ("数据数组大小")) -> ()
                n639 = global write "全局1.vi" "枚举"(enum16{"返回请求应答", "上传数据", "返回执行结果"}."上传数据" ("枚举")) -> ()
              }
              frame #1 {
                # "判定是否存表"
                n640 = property on="TCP服务端掉线计数" class="DigNum (严格)"() -> ("Value"=w701:i32)  [unwired: 2 in, 2 out]
                n641 = Greater Or Equal?(x=w701, y=1) -> (x >= y?=w700:bool)
                n642 = case shown="假" w700 {
                  frame False {
                    n643 = global read "全局 数据数组大小.vi" "数据数组大小"() -> (w703:i32)
                    n644 = Greater Than 0?(x=w703) -> (x > 0?=w704:bool)
                    n645 = case shown="真" w704 {
                      frame False {
                      }
                      frame True {
                        n646 = global read "全局 小时数据发送次数.vi" "小时数据发送次数"() -> (w713:i32)
                        n647 = local write "核查数据上传"(TRUE ("数据上传")) -> ()
                        n648 = Get Date/Time In Seconds() -> (seconds since 1Jan1904=w718:timestamp)
                        n649 = Increment(x=w713) -> (x+1=w712:i32)
                        n650 = Format Date/Time String(time format string (%c)="%Y%m%d%H%M%S%3u" ("时间格式字符串(%c)"), seconds (now)=w718) -> (date/time string=w717:string)  [unwired: 1 in]
                        n651 = global write "全局 小时数据发送次数.vi" "小时数据发送次数"(w712) -> ()
                        n652 = Search and Replace String(input string=w717, search string="." ("搜索字符串")) -> (result string=w715:string)  [unwired: 6 in, 3 out]
                        n653 = local read "MN"() -> (w710:string)
                        n654 = local read "PW"() -> (w709:string)
                        n655 = call "数据编码.vi"("table输入"="测量周期" ("新元素/子数组"), "QN"=w715, "MN"=w710, "PW"=w709) -> ("通讯包字符串"=w706:string)  [unwired: 10 in, 1 out]
                        n656 = local read "数据发送通道"() -> (w708:enum16{"TCP", "VISA"})
                        n657 = local write "发送报文显示"(w706) -> ()
                        n658 = call "VISATCP组合选择发送.vi"("数据发送通道"=w708, "命令"="write", "写入缓冲区"=w706) -> ("错误输出"=w705:errorcluster)  [unwired: 9 in, 3 out]
                        n659 = Build Array(w706) -> (w714:string[])
                        n660 = local write "错误输出"(w705) -> ()
                        n661 = call "发送数据记录到文档(子VI).vi"("数组"=w714) -> ()  [unwired: 9 in, 1 out]
                      }
                    }
                  }
                  frame True {
                  }
                }
              }
            }
          }
          frame "超标留样" {
            # "直接1分钟查询 一次,有变化就按上传,没变化就不上传"
            n662 = flat-sequence {
              frame #0 {
                # "时间"
                n663 = global write "全局 小时数据发送次数.vi" "小时数据发送次数"(0 ("小时数据发送次数")) -> ()
                n664 = global write "全局 数据数组大小.vi" "数据数组大小"(1 ("数据数组大小")) -> ()
                n665 = global write "全局1.vi" "枚举"(enum16{"返回请求应答", "上传数据", "返回执行结果"}."上传数据" ("枚举")) -> ()
              }
              frame #1 {
                # "判定是否存表"
                n666 = property on="TCP服务端掉线计数" class="DigNum (严格)"() -> ("Value"=w725:i32)  [unwired: 2 in, 2 out]
                n667 = Greater Or Equal?(x=w725, y=1) -> (x >= y?=w724:bool)
                n668 = case shown="假" w724 {
                  frame False {
                    n669 = global read "全局 数据数组大小.vi" "数据数组大小"() -> (w727:i32)
                    n670 = Greater Than 0?(x=w727) -> (x > 0?=w728:bool)
                    n671 = case shown="真" w728 {
                      frame False {
                      }
                      frame True {
                        n672 = global read "全局 小时数据发送次数.vi" "小时数据发送次数"() -> (w737:i32)
                        n673 = local write "核查数据上传"(TRUE ("数据上传")) -> ()
                        n674 = Get Date/Time In Seconds() -> (seconds since 1Jan1904=w742:timestamp)
                        n675 = Increment(x=w737) -> (x+1=w736:i32)
                        n676 = Format Date/Time String(time format string (%c)="%Y%m%d%H%M%S%3u" ("时间格式字符串(%c)"), seconds (now)=w742) -> (date/time string=w741:string)  [unwired: 1 in]
                        n677 = global write "全局 小时数据发送次数.vi" "小时数据发送次数"(w736) -> ()
                        n678 = Search and Replace String(input string=w741, search string="." ("搜索字符串")) -> (result string=w739:string)  [unwired: 6 in, 3 out]
                        n679 = local read "MN"() -> (w734:string)
                        n680 = local read "PW"() -> (w733:string)
                        n681 = call "数据编码.vi"("table输入"="超标留样" ("新元素/子数组"), "QN"=w739, "MN"=w734, "PW"=w733) -> ("通讯包字符串"=w730:string)  [unwired: 10 in, 1 out]
                        n682 = local read "数据发送通道"() -> (w732:enum16{"TCP", "VISA"})
                        n683 = local write "发送报文显示"(w730) -> ()
                        n684 = call "VISATCP组合选择发送.vi"("数据发送通道"=w732, "命令"="write", "写入缓冲区"=w730) -> ("错误输出"=w729:errorcluster)  [unwired: 9 in, 3 out]
                        n685 = Build Array(w730) -> (w738:string[])
                        n686 = local write "错误输出"(w729) -> ()
                        n687 = call "发送数据记录到文档(子VI).vi"("数组"=w738) -> ()  [unwired: 9 in, 1 out]
                      }
                    }
                  }
                  frame True {
                  }
                }
              }
            }
          }
          frame "报警信息" {
            # "间隔时间上传"
            # "直接1分钟查询 一次,有数据就按数据上传,没数据为空的不传,在数据发送那边有做处理"
            n688 = flat-sequence {
              frame #0 {
                # "分钟时间间隔"
                n689 = global read "全局 数据发送重叠.vi" "数据发送重叠开始时间戳"() -> (w746:string)
                n690 = global read "全局 数据发送重叠.vi" "数据发送重叠"() -> (w745:bool)
                n691 = global write "全局 小时数据发送次数.vi" "小时数据发送次数"(0 ("小时数据发送次数")) -> ()
                n692 = global write "全局1.vi" "枚举"(enum16{"返回请求应答", "上传数据", "返回执行结果"}."上传数据" ("枚举")) -> ()
                n693 = call "日志信息主动发送(子VI).vi"("是否正在查询数据"=w745, "查询数据发送时间节点"=w746) -> ()  [unwired: 10 in]
              }
              frame #1 {
                n694 = call "获取报警信息 (子VI).vi"() -> ()  [unwired: 12 in]
              }
              frame #2 {
                n695 = call "数据处理整合 (子VI).vi"("枚举"=enum16{"实时数据排序", "小时数据排序"}."实时数据排序") -> ("已排序的数组"=w751:string[])  [unwired: 10 in]
                n696 = Array Size(array=w751) -> (size(s)=w750:i32)
                n697 = global write "全局 数据数组大小.vi" "数据数组大小"(w750) -> ()
              }
              frame #3 {
                n698 = while {
                  stop <- w752 stop-if-true
                  # "判定是否存表"
                  n699 = property on="TCP服务端掉线计数" class="DigNum (严格)"() -> ("Value"=w758:i32)  [unwired: 2 in, 2 out]
                  n700 = Greater Or Equal?(x=w758, y=1) -> (x >= y?=w757:bool)
                  n701 = case shown="假" w757 {
                    frame False {
                      # "判定数据不为空才发"
                      n702 = global read "全局 数据数组大小.vi" "数据数组大小"() -> (w760:i32)
                      n703 = Greater Than 0?(x=w760) -> (x > 0?=w761:bool)
                      n704 = case shown="真" w761 {
                        frame False {
                          n705 = local write "核查数据上传"(FALSE ("数据上传")) -> ()
                        }
                        frame True {
                          n706 = global read "全局 小时数据发送次数.vi" "小时数据发送次数"() -> (w770:i32)
                          n707 = Get Date/Time In Seconds() -> (seconds since 1Jan1904=w775:timestamp)
                          n708 = Increment(x=w770) -> (x+1=w769:i32)
                          n709 = Format Date/Time String(time format string (%c)="%Y%m%d%H%M%S%3u" ("时间格式字符串(%c)"), seconds (now)=w775) -> (date/time string=w774:string)  [unwired: 1 in]
                          n710 = global write "全局 小时数据发送次数.vi" "小时数据发送次数"(w769) -> ()
                          n711 = Search and Replace String(input string=w774, search string="." ("搜索字符串")) -> (result string=w772:string)  [unwired: 6 in, 3 out]
                          n712 = local read "MN"() -> (w768:string)
                          n713 = local read "PW"() -> (w767:string)
                          n714 = local read "数据发送通道"() -> (w766:enum16{"TCP", "VISA"})
                          n715 = call "数据编码.vi"("table输入"="报警信息" ("新元素/子数组"), "QN"=w772, "MN"=w768, "PW"=w767) -> ("通讯包字符串"=w764:string)  [unwired: 10 in, 1 out]
                          n716 = local write "发送报文显示"(w764) -> ()
                          n717 = Build Array(w764) -> (w771:string[])
                          n718 = call "VISATCP组合选择发送.vi"("数据发送通道"=w766, "命令"="write", "写入缓冲区"=w764) -> ("错误输出"=w763:errorcluster)  [unwired: 9 in, 3 out]
                          n719 = local write "错误输出"(w763) -> ()
                          n720 = call "发送数据记录到文档(子VI).vi"("数组"=w771) -> ()  [unwired: 9 in, 1 out]
                        }
                      }
                    }
                    frame True {
                    }
                  }
                  n721 = Wait (ms)(milliseconds to wait=u32 500 ("等待时间（毫秒）")) -> ()  [unwired: 1 out]
                  n722 = global read "全局 数据数组大小.vi" "数据数组大小"() -> (w754:i32)
                  n723 = global read "全局 小时数据发送次数.vi" "小时数据发送次数"() -> (w756:i32)
                  n724 = Decrement(x=w754) -> (x-1=w753:i32)
                  n725 = Greater Or Equal?(x=w756, y=w753) -> (x >= y?=w752:bool)
                }
              }
            }
          }
          frame "环境参数" {
            # "间隔时间上传"
            # "直接1分钟查询 一次,有数据就按数据上传,没数据为空的不传,在数据发送那边有做处理"
            n726 = disable-structure shown="禁用" {
              frame Disabled {
                n727 = flat-sequence {
                  frame #0 {
                    # "分钟时间间隔"
                    n728 = global read "全局 数据发送重叠.vi" "数据发送重叠开始时间戳"() -> (w779:string)
                    n729 = global read "全局 数据发送重叠.vi" "数据发送重叠"() -> (w778:bool)
                    n730 = global write "全局 小时数据发送次数.vi" "小时数据发送次数"(0 ("小时数据发送次数")) -> ()
                    n731 = global write "全局1.vi" "枚举"(enum16{"返回请求应答", "上传数据", "返回执行结果"}."上传数据" ("枚举")) -> ()
                    n732 = call "日志信息主动发送(子VI).vi"("是否正在查询数据"=w778, "查询数据发送时间节点"=w779) -> ()  [unwired: 10 in]
                  }
                  frame #1 {
                    n733 = call "获取环境参数 (子VI).vi"() -> ()  [unwired: 12 in]
                  }
                  frame #2 {
                    n734 = call "数据处理整合 (子VI).vi"("枚举"=enum16{"实时数据排序", "小时数据排序"}."实时数据排序") -> ("已排序的数组"=w784:string[])  [unwired: 10 in]
                    n735 = Array Size(array=w784) -> (size(s)=w783:i32)
                    n736 = global write "全局 数据数组大小.vi" "数据数组大小"(w783) -> ()
                  }
                  frame #3 {
                    n737 = while {
                      stop <- w785 stop-if-true
                      # "判定是否存表"
                      n738 = property on="TCP服务端掉线计数" class="DigNum (严格)"() -> ("Value"=w791:i32)  [unwired: 2 in, 2 out]
                      n739 = Greater Or Equal?(x=w791, y=1) -> (x >= y?=w790:bool)
                      n740 = case shown="假" w790 {
                        frame False {
                          # "判定数据不为空才发"
                          n741 = global read "全局 数据数组大小.vi" "数据数组大小"() -> (w793:i32)
                          n742 = Greater Than 0?(x=w793) -> (x > 0?=w794:bool)
                          n743 = case shown="真" w794 {
                            frame False {
                            }
                            frame True {
                              n744 = global read "全局 小时数据发送次数.vi" "小时数据发送次数"() -> (w801:i32)
                              n745 = local write "核查数据上传"(TRUE ("数据上传")) -> ()
                              n746 = Get Date/Time In Seconds() -> (seconds since 1Jan1904=w806:timestamp)
                              n747 = Increment(x=w801) -> (x+1=w800:i32)
                              n748 = Format Date/Time String(time format string (%c)="%Y%m%d%H%M%S%3u" ("时间格式字符串(%c)"), seconds (now)=w806) -> (date/time string=w805:string)  [unwired: 1 in]
                              n749 = global write "全局 小时数据发送次数.vi" "小时数据发送次数"(w800) -> ()
                              n750 = Search and Replace String(input string=w805, search string="." ("搜索字符串")) -> (result string=w803:string)  [unwired: 6 in, 3 out]
                              n751 = local read "MN"() -> (w809:string)
                              n752 = local read "PW"() -> (w808:string)
                              n753 = local read "数据发送通道"() -> (w797:enum16{"TCP", "VISA"})
                              n754 = call "数据编码.vi"("table输入"="报警信息" ("新元素/子数组"), "QN"=w803, "MN"=w809, "PW"=w808) -> ("通讯包字符串"=w796:string)  [unwired: 10 in, 1 out]
                              n755 = local write "发送报文显示"(w796) -> ()
                              n756 = call "VISATCP组合选择发送.vi"("数据发送通道"=w797, "命令"="write", "写入缓冲区"=w796) -> ("错误输出"=w795:errorcluster)  [unwired: 9 in, 3 out]
                              n757 = Build Array(w796) -> (w802:string[])
                              n758 = local write "错误输出"(w795) -> ()
                              n759 = call "发送数据记录到文档(子VI).vi"("数组"=w802) -> ()  [unwired: 9 in, 1 out]
                            }
                          }
                        }
                        frame True {
                        }
                      }
                      n760 = Wait (ms)(milliseconds to wait=u32 500 ("等待时间（毫秒）")) -> ()  [unwired: 1 out]
                      n761 = global read "全局 数据数组大小.vi" "数据数组大小"() -> (w787:i32)
                      n762 = global read "全局 小时数据发送次数.vi" "小时数据发送次数"() -> (w789:i32)
                      n763 = Decrement(x=w787) -> (x-1=w786:i32)
                      n764 = Greater Or Equal?(x=w789, y=w786) -> (x >= y?=w785:bool)
                    }
                  }
                }
              }
              frame Enabled {
              }
            }
          }
        }
      }
    }
  }
  n765 = while "While循环" {
    tunnel: [w825] -> _
    tunnel: w37 -> [w819]
    stop <- FALSE stop-if-true
    w813 = FALSE ("小时数据上传")
    # "实时、小时数据出数据就上传"
    n766 = property on="TCP服务端掉线计数" class="DigNum (严格)"() -> ("Value"=w822:i32)  [unwired: 2 in, 2 out]
    n767 = local read "查询数据发送"() -> (w815:bool)
    n768 = local read "核查数据上传"() -> (w814:bool)
    n769 = local read "步骤"() -> (w824:T6)
    n770 = local write "实时小时数据上传"(w813) -> ()
    n771 = global write "全局 数据发送重叠.vi" "主动上报数据中"(w813) -> ()
    n772 = Greater Or Equal?(x=w819, y=17) -> (x >= y?=w818:bool)
    n773 = Equal To 0?(x=w822) -> (x = 0?=w820:bool)
    n774 = Not(x=w815) -> (.not. x?=w812:bool)
    n775 = Not(x=w814) -> (.not. x?=w811:bool)
    n776 = Equal?(x=w824, y=T6."读取数据" ("步骤")) -> (x = y?=w821:bool)
    n777 = Wait (ms)(milliseconds to wait=u32 75430 ("等待时间（毫秒）")) -> ()  [unwired: 1 out]
    n778 = Compound Arithmetic op=AND ("复合运算")(w821, w820, w818, w812, w811) -> (w816:bool)
    n779 = case shown="真" w816 {
      tunnel: [_ w830] -> w825
      frame False {
        w828 = FALSE ("小时数据上传")
        n780 = local write "实时小时数据上传"(w828) -> ()
        n781 = global write "全局 数据发送重叠.vi" "主动上报数据中"(w828) -> ()
      }
      frame True {
        n782 = global read "断电保存全局.vi" "数据组合发送"() -> (w829:bool)
        n783 = case shown="假" w829 {
          tunnel: [w831 _] -> w830
          frame False {
            # "数据非整点触发，而是实时触发，分条发送"
            n784 = flat-sequence {
              tunnel: [w835] -> w832
              tunnel: [w1201] -> w831
              tunnel: w832 -> [w1201]
              frame #0 {
                w833 = TRUE ("小时数据上传")
                n785 = global write "全局 数据发送重叠.vi" "主动上报数据中"(w833) -> ()
                n786 = local read "数据发送协议"() -> (w834:enum16{"2005-212协议", "2017-212协议"})
                n787 = case shown="\"2017-212协议\", 默认" w834 {
                  tunnel: [_ w971] -> w835
                  frame "2005-212协议" {
                    n788 = local read "参数数值"() -> (w839:T5)
                    n789 = Cluster To Array(cluster=w839) -> (array=w838:bool[])
                    n790 = for {
                      tunnel: w838 -> [_] mode=indexing
                      tunnel: [w883] -> w837
                      i -> [w877]
                      w878 = "1904/01/01 00:00:00"
                      (unwired) " where 时间 between #"
                      w881 = "database1.mdb" ("database")
                      (unwired) "'and 数据类型 ='N' and 时间 between "
                      w885 = 0 ("索引 (行)")
                      n791 = case shown="12" w877 {
                        tunnel: [w935 w937 w939 w941 w943 w945 w947 w949 w951 w953 w955 w957 w959 w961 w963 w965 w967 w969] -> w880
                        frame 0, Default {
                          n792 = control-ref of="CODMn"() -> (w936:refnum<vi>)
                          n793 = property class="Bool (严格)"(reference=w936) -> ("Label.Text"=w935:string)  [unwired: 1 in, 2 out]
                        }
                        frame 1 {
                          n794 = control-ref of="CODCr"() -> (w938:refnum<vi>)
                          n795 = property class="Bool (严格)"(reference=w938) -> ("Label.Text"=w937:string)  [unwired: 1 in, 2 out]
                        }
                        frame 2 {
                          n796 = control-ref of="DO"() -> (w940:refnum<vi>)
                          n797 = property class="Bool (严格)"(reference=w940) -> ("Label.Text"=w939:string)  [unwired: 1 in, 2 out]
                        }
                        frame 3 {
                          n798 = control-ref of="铜"() -> (w942:refnum<vi>)
                          n799 = property class="Bool (严格)"(reference=w942) -> ("Label.Text"=w941:string)  [unwired: 1 in, 2 out]
                        }
                        frame 4 {
                          n800 = control-ref of="PH"() -> (w944:refnum<vi>)
                          n801 = property class="Bool (严格)"(reference=w944) -> ("Label.Text"=w943:string)  [unwired: 1 in, 2 out]
                        }
                        frame 5 {
                          n802 = control-ref of="氨氮"() -> (w946:refnum<vi>)
                          n803 = property class="Bool (严格)"(reference=w946) -> ("Label.Text"=w945:string)  [unwired: 1 in, 2 out]
                        }
                        frame 6 {
                          n804 = control-ref of="比电导率"() -> (w948:refnum<vi>)
                          n805 = property class="Bool (严格)"(reference=w948) -> ("Label.Text"=w947:string)  [unwired: 1 in, 2 out]
                        }
                        frame 7 {
                          n806 = control-ref of="水温"() -> (w950:refnum<vi>)
                          n807 = property class="Bool (严格)"(reference=w950) -> ("Label.Text"=w949:string)  [unwired: 1 in, 2 out]
                        }
                        frame 8 {
                          n808 = control-ref of="盐度(海水)"() -> (w952:refnum<vi>)
                          n809 = property class="Bool (严格)"(reference=w952) -> ("Label.Text"=w951:string)  [unwired: 1 in, 2 out]
                        }
                        frame 9 {
                          n810 = control-ref of="浊度"() -> (w954:refnum<vi>)
                          n811 = property class="Bool (严格)"(reference=w954) -> ("Label.Text"=w953:string)  [unwired: 1 in, 2 out]
                        }
                        frame 10 {
                          n812 = control-ref of="总氮"() -> (w956:refnum<vi>)
                          n813 = property class="Bool (严格)"(reference=w956) -> ("Label.Text"=w955:string)  [unwired: 1 in, 2 out]
                        }
                        frame 11 {
                          n814 = control-ref of="总磷"() -> (w958:refnum<vi>)
                          n815 = property class="Bool (严格)"(reference=w958) -> ("Label.Text"=w957:string)  [unwired: 1 in, 2 out]
                        }
                        frame 12 {
                          n816 = control-ref of="叶绿素a"() -> (w960:refnum<vi>)
                          n817 = property class="Bool (严格)"(reference=w960) -> ("Label.Text"=w959:string)  [unwired: 1 in, 2 out]
                        }
                        frame 13 {
                          n818 = control-ref of="藻密度"() -> (w962:refnum<vi>)
                          n819 = property class="Bool (严格)"(reference=w962) -> ("Label.Text"=w961:string)  [unwired: 1 in, 2 out]
                        }
                        frame 14 {
                          n820 = control-ref of="水位"() -> (w964:refnum<vi>)
                          n821 = property class="Bool (严格)"(reference=w964) -> ("Label.Text"=w963:string)  [unwired: 1 in, 2 out]
                        }
                        frame 15 {
                          n822 = control-ref of="流速"() -> (w966:refnum<vi>)
                          n823 = property class="Bool (严格)"(reference=w966) -> ("Label.Text"=w965:string)  [unwired: 1 in, 2 out]
                        }
                        frame 16 {
                          n824 = control-ref of="瞬时流量"() -> (w968:refnum<vi>)
                          n825 = property class="Bool (严格)"(reference=w968) -> ("Label.Text"=w967:string)  [unwired: 1 in, 2 out]
                        }
                        frame 17 {
                          n826 = control-ref of="累积流量"() -> (w970:refnum<vi>)
                          n827 = property class="Bool (严格)"(reference=w970) -> ("Label.Text"=w969:string)  [unwired: 1 in, 2 out]
                        }
                      }
                      n828 = Get Date/Time In Seconds() -> (seconds since 1Jan1904=w889:timestamp)
                      n829 = Format Date/Time String(time format string (%c)="%Y/%m/%d %H:%M:%S" ("时间格式字符串(%c)"), seconds (now)=w889) -> (date/time string=w879:string)  [unwired: 1 in]
                      n830 = Format Into String(format string="#%s#" ("初始字符串"), w878) -> (resulting string=w887:string)  [unwired: 2 in, 1 out]
                      n831 = Format Into String(format string="#%s#" ("初始字符串"), w879) -> (resulting string=w882:string)  [unwired: 2 in, 1 out]
                      n832 = case shown="0, 默认" w877 {
                        selector: w877 -> [_ w921]
                        tunnel: w887 -> [w916 w926]
                        tunnel: [w915 w927] -> w886
                        tunnel: w882 -> [w912 w925]
                        tunnel: w881 -> [_ w924]
                        tunnel: w880 -> [_ w923]
                        tunnel: w878 -> [_ w918]
                        tunnel: w879 -> [_ w920]
                        frame 0, Default {
                          n833 = Concatenate Strings("where 测量模式 ='水样测试" ("condition"), "'and 时间 between ", w916, "and" ("字符串"), w912, " order by 时间 desc" ("字符串")) -> (w915:string)
                        }
                        frame 14..17 {
                          n834 = call "流量数据规范小时时间戳.vi"("字符串"=w918) -> ("result string"=w917:string)  [unwired: 10 in]
                          n835 = call "database1查询.vi"("时间2"=w920, "table"=w923, "时间1"=w917, "database"=w924) -> ("error out"=w919:errorcluster, "data"=w922:string[][])  [unwired: 4 in, 1 out]
                          n836 = call <vilib>:"Clear Errors.vi"("error in (no error)"=w919) -> ()  [unwired: 5 in, 2 out]
                          n837 = case shown="14" w921 {
                            tunnel: w922 -> [_ w931 w932 w933 w934]
                            frame 0, Default {
                            }
                            frame 14 {
                              n838 = global write "全局流量数据小时.vi" "水位"(w931) -> ()
                            }
                            frame 15 {
                              n839 = global write "全局流量数据小时.vi" "流速"(w932) -> ()
                            }
                            frame 16 {
                              n840 = global write "全局流量数据小时.vi" "瞬时流量"(w933) -> ()
                            }
                            frame 17 {
                              n841 = global write "全局流量数据小时.vi" "累积流量"(w934) -> ()
                            }
                          }
                          n842 = Concatenate Strings(" where 时间 between ", w926, "and" ("字符串"), w925, " order by 时间 desc" ("字符串")) -> (w927:string)
                        }
                      }
                      n843 = call "SQL查询.vi"("condition"=w886, "table输入"=w880, "database"=w881) -> ("error out"=w883:errorcluster, "data"=w876:string[][])  [unwired: 7 in]
                      n844 = call "短日期时间转长日期格式.vi"("data"=w876) -> ("输出数组"=w884:string[][])  [unwired: 10 in]
                      n845 = case shown="3" w877 {
                        tunnel: w876 -> [w892 w893 w894 w895 w896 w897 w898 w899 w900 w901 w902 w903 w904 w905 w906 w907 w908 w909]
                        frame 0, Default {
                          n846 = global write "全局 所有参数.vi" "CODMn"(w892) -> ()
                        }
                        frame 1 {
                          n847 = global write "全局 所有参数.vi" "CODCr"(w893) -> ()
                        }
                        frame 2 {
                          n848 = global write "全局 所有参数.vi" "DO"(w894) -> ()
                        }
                        frame 3 {
                          n849 = global write "全局 所有参数.vi" "铜"(w895) -> ()
                        }
                        frame 4 {
                          n850 = global write "全局 所有参数.vi" "PH"(w896) -> ()
                        }
                        frame 5 {
                          n851 = global write "全局 所有参数.vi" "氨氮"(w897) -> ()
                        }
                        frame 6 {
                          n852 = global write "全局 所有参数.vi" "电导率"(w898) -> ()
                        }
                        frame 7 {
                          n853 = global write "全局 所有参数.vi" "水温"(w899) -> ()
                        }
                        frame 8 {
                          n854 = global write "全局 所有参数.vi" "盐度"(w900) -> ()
                        }
                        frame 9 {
                          n855 = global write "全局 所有参数.vi" "浊度"(w901) -> ()
                        }
                        frame 10 {
                          n856 = global write "全局 所有参数.vi" "总氮"(w902) -> ()
                        }
                        frame 11 {
                          n857 = global write "全局 所有参数.vi" "总磷"(w903) -> ()
                        }
                        frame 12 {
                          n858 = global write "全局 所有参数.vi" "叶绿素"(w904) -> ()
                        }
                        frame 13 {
                          n859 = global write "全局 所有参数.vi" "藻密度"(w905) -> ()
                        }
                        frame 14 {
                          n860 = global write "全局 所有参数.vi" "水位"(w906) -> ()
                        }
                        frame 15 {
                          n861 = global write "全局 所有参数.vi" "流速"(w907) -> ()
                        }
                        frame 16 {
                          n862 = global write "全局 所有参数.vi" "瞬时流量"(w908) -> ()
                        }
                        frame 17 {
                          n863 = global write "全局 所有参数.vi" "累积流量"(w909) -> ()
                        }
                      }
                      n864 = Index Array(array=w884, index (row)=w885, index (col)=w885) -> ()  [unwired: 1 out]
                    }
                    n865 = flat-sequence {
                      tunnel: w837 -> [w840]
                      tunnel: [w840] -> w836
                      tunnel: w836 -> [w846]
                      tunnel: [w845] -> _
                      frame #0 {
                        n866 = global write "全局 小时数据发送次数.vi" "小时数据发送次数"(0 ("小时数据发送次数")) -> ()
                        n867 = call "数据处理直接插入整合 (子VI).vi"() -> ()  [unwired: 12 in]
                        n868 = global write "全局1.vi" "枚举"(enum16{"返回请求应答", "上传数据", "返回执行结果"}."上传数据" ("枚举")) -> ()
                        n869 = global write "全局 实时数据参数.vi" "实时数据参数"("水样测试" ("实时数据参数")) -> ()
                        n870 = global write "全局 水样时间.vi" "选择发送的参数"("氨氮" ("选择发送的参数")) -> ()
                      }
                      frame #1 {
                        # "实时数据的大小"
                        n871 = flat-sequence {
                          tunnel: [w852] -> w849
                          tunnel: [w851] -> w847
                          tunnel: w846 -> [w850]
                          tunnel: w849 -> [_]
                          tunnel: [w865] -> w848
                          tunnel: w847 -> [w865]
                          tunnel: w848 -> [w873]
                          tunnel: [w867] -> w845
                          frame #0 {
                            n872 = Get Date/Time In Seconds() -> (seconds since 1Jan1904=w860:timestamp)
                            n873 = Format Date/Time String(time format string (%c)="%Y%m%d%H%M%S%3u" ("时间格式字符串(%c)"), seconds (now)=w860) -> (date/time string=w861:string)  [unwired: 1 in]
                            n874 = Search and Replace String(input string=w861, search string="." ("搜索字符串")) -> (result string=w863:string)  [unwired: 6 in, 3 out]
                            n875 = local read "MN"() -> (w856:string)
                            n876 = local read "PW"() -> (w855:string)
                            n877 = local read "数据发送通道"() -> (w854:enum16{"TCP", "VISA"})
                            n878 = call "数据编码.vi"("table输入"="小时数据" ("新元素/子数组"), "QN"=w863, "MN"=w856, "PW"=w855) -> ("通讯包字符串"=w852:string)  [unwired: 10 in, 1 out]
                            n879 = Build Array(w852) -> (w857:string[])
                            n880 = local write "发送报文显示"(w852) -> ()
                            n881 = call "VISATCP组合选择发送.vi"("数据发送通道"=w854, "命令"="write", "写入缓冲区"=w852) -> ()  [unwired: 9 in, 4 out]
                            n882 = call "发送数据记录到文档(子VI).vi"("错误输入"=w850, "数组"=w857) -> ("错误输出"=w851:errorcluster)  [unwired: 8 in]
                          }
                          frame #1 {
                            n883 = global write "全局 小时数据发送次数.vi" "小时数据发送次数"(0 ("小时数据发送次数")) -> ()
                            n884 = Wait (ms)(milliseconds to wait=u32 500 ("等待时间（毫秒）")) -> ()  [unwired: 1 out]
                          }
                          frame #2 {
                            n885 = local read "MN"() -> (w872:string)
                            n886 = local read "PW"() -> (w871:string)
                            n887 = call "数据编码.vi"("table输入"="实时数据" ("新元素/子数组"), "错误常量 2"=w873, "MN"=w872, "PW"=w871) -> ("通讯包字符串"=w868:string)  [unwired: 10 in, 1 out]
                            n888 = Build Array(w868) -> (w875:string[])
                            n889 = local read "数据发送通道"() -> (w870:enum16{"TCP", "VISA"})
                            n890 = local write "发送报文显示"(w868) -> ()
                            n891 = call "发送数据记录到文档(子VI).vi"("数组"=w875) -> ()  [unwired: 9 in, 1 out]
                            n892 = call "VISATCP组合选择发送.vi"("数据发送通道"=w870, "命令"="write", "写入缓冲区"=w868) -> ("错误输出"=w867:errorcluster)  [unwired: 9 in, 3 out]
                          }
                        }
                      }
                    }
                  }
                  frame "2017-212协议", Default {
                    n893 = local read "参数数值"() -> (w973:T5)
                    n894 = Cluster To Array(cluster=w973) -> (array=w972:bool[])
                    n895 = for {
                      tunnel: w972 -> [_] mode=indexing
                      tunnel: [w980] -> w971 mode=indexing
                      tunnel: [w980] -> _
                      i -> [w978]
                      (unwired) " where 时间 between #"
                      w977 = "database1.mdb" ("database")
                      (unwired) "'and 数据类型 ='N' and 时间 between "
                      w994 = 0 ("索引 (行)")
                      n896 = case shown="3" w978 {
                        tunnel: [w1164 w1166 w1168 w1170 w1172 w1174 w1176 w1178 w1180 w1182 w1184 w1186 w1188 w1190 w1192 w1194 w1196 w1198] -> w976
                        frame 0, Default {
                          n897 = control-ref of="CODMn"() -> (w1165:refnum<vi>)
                          n898 = property class="Bool (严格)"(reference=w1165) -> ("Label.Text"=w1164:string)  [unwired: 1 in, 2 out]
                        }
                        frame 1 {
                          n899 = control-ref of="CODCr"() -> (w1167:refnum<vi>)
                          n900 = property class="Bool (严格)"(reference=w1167) -> ("Label.Text"=w1166:string)  [unwired: 1 in, 2 out]
                        }
                        frame 2 {
                          n901 = control-ref of="DO"() -> (w1169:refnum<vi>)
                          n902 = property class="Bool (严格)"(reference=w1169) -> ("Label.Text"=w1168:string)  [unwired: 1 in, 2 out]
                        }
                        frame 3 {
                          n903 = control-ref of="铜"() -> (w1171:refnum<vi>)
                          n904 = property class="Bool (严格)"(reference=w1171) -> ("Label.Text"=w1170:string)  [unwired: 1 in, 2 out]
                        }
                        frame 4 {
                          n905 = control-ref of="PH"() -> (w1173:refnum<vi>)
                          n906 = property class="Bool (严格)"(reference=w1173) -> ("Label.Text"=w1172:string)  [unwired: 1 in, 2 out]
                        }
                        frame 5 {
                          n907 = control-ref of="氨氮"() -> (w1175:refnum<vi>)
                          n908 = property class="Bool (严格)"(reference=w1175) -> ("Label.Text"=w1174:string)  [unwired: 1 in, 2 out]
                        }
                        frame 6 {
                          n909 = control-ref of="比电导率"() -> (w1177:refnum<vi>)
                          n910 = property class="Bool (严格)"(reference=w1177) -> ("Label.Text"=w1176:string)  [unwired: 1 in, 2 out]
                        }
                        frame 7 {
                          n911 = control-ref of="水温"() -> (w1179:refnum<vi>)
                          n912 = property class="Bool (严格)"(reference=w1179) -> ("Label.Text"=w1178:string)  [unwired: 1 in, 2 out]
                        }
                        frame 8 {
                          n913 = control-ref of="盐度(海水)"() -> (w1181:refnum<vi>)
                          n914 = property class="Bool (严格)"(reference=w1181) -> ("Label.Text"=w1180:string)  [unwired: 1 in, 2 out]
                        }
                        frame 9 {
                          n915 = control-ref of="浊度"() -> (w1183:refnum<vi>)
                          n916 = property class="Bool (严格)"(reference=w1183) -> ("Label.Text"=w1182:string)  [unwired: 1 in, 2 out]
                        }
                        frame 10 {
                          n917 = control-ref of="总氮"() -> (w1185:refnum<vi>)
                          n918 = property class="Bool (严格)"(reference=w1185) -> ("Label.Text"=w1184:string)  [unwired: 1 in, 2 out]
                        }
                        frame 11 {
                          n919 = control-ref of="总磷"() -> (w1187:refnum<vi>)
                          n920 = property class="Bool (严格)"(reference=w1187) -> ("Label.Text"=w1186:string)  [unwired: 1 in, 2 out]
                        }
                        frame 12 {
                          n921 = control-ref of="叶绿素a"() -> (w1189:refnum<vi>)
                          n922 = property class="Bool (严格)"(reference=w1189) -> ("Label.Text"=w1188:string)  [unwired: 1 in, 2 out]
                        }
                        frame 13 {
                          n923 = control-ref of="藻密度"() -> (w1191:refnum<vi>)
                          n924 = property class="Bool (严格)"(reference=w1191) -> ("Label.Text"=w1190:string)  [unwired: 1 in, 2 out]
                        }
                        frame 14 {
                          n925 = control-ref of="水位"() -> (w1193:refnum<vi>)
                          n926 = property class="Bool (严格)"(reference=w1193) -> ("Label.Text"=w1192:string)  [unwired: 1 in, 2 out]
                        }
                        frame 15 {
                          n927 = control-ref of="流速"() -> (w1195:refnum<vi>)
                          n928 = property class="Bool (严格)"(reference=w1195) -> ("Label.Text"=w1194:string)  [unwired: 1 in, 2 out]
                        }
                        frame 16 {
                          n929 = control-ref of="瞬时流量"() -> (w1197:refnum<vi>)
                          n930 = property class="Bool (严格)"(reference=w1197) -> ("Label.Text"=w1196:string)  [unwired: 1 in, 2 out]
                        }
                        frame 17 {
                          n931 = control-ref of="累积流量"() -> (w1199:refnum<vi>)
                          n932 = property class="Bool (严格)"(reference=w1199) -> ("Label.Text"=w1198:string)  [unwired: 1 in, 2 out]
                        }
                      }
                      n933 = case shown="12" w978 {
                        tunnel: [w1146 w1147 w1148 w1149 w1150 w1151 w1152 w1153 w1154 w1155 w1156 w1157 w1158 w1159 w1160 w1161 w1162 w1163] -> w975
                        frame 0, Default {
                          n934 = global read "全局 水样时间.vi" "time1"() -> (w1146:string)
                        }
                        frame 1 {
                          n935 = global read "全局 水样时间.vi" "time2"() -> (w1147:string)
                        }
                        frame 2 {
                          n936 = global read "全局 水样时间.vi" "time3"() -> (w1148:string)
                        }
                        frame 3 {
                          n937 = global read "全局 水样时间.vi" "time4"() -> (w1149:string)
                        }
                        frame 4 {
                          n938 = global read "全局 水样时间.vi" "time5"() -> (w1150:string)
                        }
                        frame 5 {
                          n939 = global read "全局 水样时间.vi" "time6"() -> (w1151:string)
                        }
                        frame 6 {
                          n940 = global read "全局 水样时间.vi" "time7"() -> (w1152:string)
                        }
                        frame 7 {
                          n941 = global read "全局 水样时间.vi" "time8"() -> (w1153:string)
                        }
                        frame 8 {
                          n942 = global read "全局 水样时间.vi" "time9"() -> (w1154:string)
                        }
                        frame 9 {
                          n943 = global read "全局 水样时间.vi" "time10"() -> (w1155:string)
                        }
                        frame 10 {
                          n944 = global read "全局 水样时间.vi" "time11"() -> (w1156:string)
                        }
                        frame 11 {
                          n945 = global read "全局 水样时间.vi" "time12"() -> (w1157:string)
                        }
                        frame 12 {
                          n946 = global read "全局 水样时间.vi" "time13"() -> (w1158:string)
                        }
                        frame 13 {
                          n947 = global read "全局 水样时间.vi" "time14"() -> (w1159:string)
                        }
                        frame 14 {
                          n948 = global read "全局 水样时间.vi" "time15"() -> (w1160:string)
                        }
                        frame 15 {
                          n949 = global read "全局 水样时间.vi" "time16"() -> (w1161:string)
                        }
                        frame 16 {
                          n950 = global read "全局 水样时间.vi" "time17"() -> (w1162:string)
                        }
                        frame 17 {
                          n951 = global read "全局 水样时间.vi" "time18"() -> (w1163:string)
                        }
                      }
                      n952 = Get Date/Time In Seconds() -> (seconds since 1Jan1904=w999:timestamp)
                      n953 = Format Date/Time String(time format string (%c)="%Y/%m/%d %H:%M:%S" ("时间格式字符串(%c)"), seconds (now)=w999) -> (date/time string=w974:string)  [unwired: 1 in]
                      n954 = Format Into String(format string="#%s#" ("初始字符串"), w975) -> (resulting string=w997:string)  [unwired: 2 in, 1 out]
                      n955 = Format Into String(format string="#%s#" ("初始字符串"), w974) -> (resulting string=w979:string)  [unwired: 2 in, 1 out]
                      n956 = case shown="0, 默认" w978 {
                        selector: w978 -> [_ w1013]
                        tunnel: w997 -> [w1008 w1018]
                        tunnel: [w1007 w1019] -> w996
                        tunnel: w979 -> [w1004 w1017]
                        tunnel: w977 -> [_ w1016]
                        tunnel: w976 -> [_ w1015]
                        tunnel: w975 -> [_ w1010]
                        tunnel: w974 -> [_ w1012]
                        frame 0, Default {
                          n957 = Concatenate Strings("where 测量模式 ='水样测试" ("condition"), "'and 时间 between ", w1008, "and" ("字符串"), w1004, " order by 时间 desc" ("字符串")) -> (w1007:string)
                        }
                        frame 14..17 {
                          n958 = call "流量数据规范小时时间戳.vi"("字符串"=w1010) -> ("result string"=w1009:string)  [unwired: 10 in]
                          n959 = call "database1查询.vi"("时间2"=w1012, "table"=w1015, "时间1"=w1009, "database"=w1016) -> ("error out"=w1011:errorcluster, "data"=w1014:string[][])  [unwired: 4 in, 1 out]
                          n960 = call <vilib>:"Clear Errors.vi"("error in (no error)"=w1011) -> ()  [unwired: 5 in, 2 out]
                          n961 = case shown="14" w1013 {
                            tunnel: w1014 -> [_ w1023 w1024 w1025 w1026]
                            frame 0, Default {
                            }
                            frame 14 {
                              n962 = global write "全局流量数据小时.vi" "水位"(w1023) -> ()
                            }
                            frame 15 {
                              n963 = global write "全局流量数据小时.vi" "流速"(w1024) -> ()
                            }
                            frame 16 {
                              n964 = global write "全局流量数据小时.vi" "瞬时流量"(w1025) -> ()
                            }
                            frame 17 {
                              n965 = global write "全局流量数据小时.vi" "累积流量"(w1026) -> ()
                            }
                          }
                          n966 = Concatenate Strings(" where 时间 between ", w1018, "and" ("字符串"), w1017, " order by 时间 desc" ("字符串")) -> (w1019:string)
                        }
                      }
                      n967 = call "SQL查询.vi"("condition"=w996, "table输入"=w976, "database"=w977) -> ("error out"=w980:errorcluster, "data"=w992:string[][])  [unwired: 7 in]
                      n968 = Empty Array?(array=w992) -> (empty?=w995:bool)
                      n969 = call "短日期时间转长日期格式.vi"("data"=w992) -> ("输出数组"=w993:string[][])  [unwired: 10 in]
                      n970 = Not(x=w995) -> (.not. x?=w989:bool)
                      n971 = Index Array(array=w993, index (row)=w994, index (col)=w994) -> (element=w986:string)
                      n972 = global write "全局 水样时间.vi" "选择发送的参数"(w976) -> ()
                      n973 = flat-sequence {
                        tunnel: [w1034] -> w991
                        tunnel: [w1033] -> w990
                        tunnel: w989 -> [w1034]
                        tunnel: w992 -> [w1033]
                        tunnel: w978 -> [w1028]
                        tunnel: w976 -> [w1030]
                        tunnel: [w1030] -> w987
                        tunnel: w986 -> [w1029]
                        tunnel: [w1029] -> w984
                        tunnel: [w1028] -> w981
                        tunnel: w991 -> [w1054]
                        tunnel: w990 -> [w1057]
                        tunnel: [w1056] -> w988
                        tunnel: w987 -> [w1056]
                        tunnel: [w1055] -> w985
                        tunnel: w984 -> [w1055]
                        tunnel: [w1054] -> w983
                        tunnel: [w1053] -> w982
                        tunnel: w981 -> [w1053]
                        tunnel: w988 -> [w1114]
                        tunnel: w985 -> [w1113]
                        tunnel: w983 -> [w1111]
                        tunnel: w982 -> [w1112]
                        frame #0 {
                          n974 = case shown="3" w1028 {
                            tunnel: w1033 -> [w1035 w1036 w1037 w1038 w1039 w1040 w1041 w1042 w1043 w1044 w1045 w1046 w1047 w1048 w1049 w1050 w1051 w1052]
                            frame 0, Default {
                              n975 = global write "全局 所有参数.vi" "CODMn"(w1035) -> ()
                            }
                            frame 1 {
                              n976 = global write "全局 所有参数.vi" "CODCr"(w1036) -> ()
                            }
                            frame 2 {
                              n977 = global write "全局 所有参数.vi" "DO"(w1037) -> ()
                            }
                            frame 3 {
                              n978 = global write "全局 所有参数.vi" "铜"(w1038) -> ()
                            }
                            frame 4 {
                              n979 = global write "全局 所有参数.vi" "PH"(w1039) -> ()
                            }
                            frame 5 {
                              n980 = global write "全局 所有参数.vi" "氨氮"(w1040) -> ()
                            }
                            frame 6 {
                              n981 = global write "全局 所有参数.vi" "电导率"(w1041) -> ()
                            }
                            frame 7 {
                              n982 = global write "全局 所有参数.vi" "水温"(w1042) -> ()
                            }
                            frame 8 {
                              n983 = global write "全局 所有参数.vi" "盐度"(w1043) -> ()
                            }
                            frame 9 {
                              n984 = global write "全局 所有参数.vi" "浊度"(w1044) -> ()
                            }
                            frame 10 {
                              n985 = global write "全局 所有参数.vi" "总氮"(w1045) -> ()
                            }
                            frame 11 {
                              n986 = global write "全局 所有参数.vi" "总磷"(w1046) -> ()
                            }
                            frame 12 {
                              n987 = global write "全局 所有参数.vi" "叶绿素"(w1047) -> ()
                            }
                            frame 13 {
                              n988 = global write "全局 所有参数.vi" "藻密度"(w1048) -> ()
                            }
                            frame 14 {
                              n989 = global write "全局 所有参数.vi" "水位"(w1049) -> ()
                            }
                            frame 15 {
                              n990 = global write "全局 所有参数.vi" "流速"(w1050) -> ()
                            }
                            frame 16 {
                              n991 = global write "全局 所有参数.vi" "瞬时流量"(w1051) -> ()
                            }
                            frame 17 {
                              n992 = global write "全局 所有参数.vi" "累积流量"(w1052) -> ()
                            }
                          }
                          n993 = global write "全局 小时数据发送次数.vi" "小时数据发送次数"(0 ("小时数据发送次数")) -> ()
                          n994 = global write "全局 数据发送重叠.vi" "数据接收超时指示灯"(FALSE ("数据接收超时指示灯")) -> ()
                          n995 = global write "全局1.vi" "枚举"(enum16{"返回请求应答", "上传数据", "返回执行结果"}."上传数据" ("枚举")) -> ()
                        }
                        frame #1 {
                          n996 = case shown="真" w1054 {
                            tunnel: w1057 -> [_ w1060]
                            tunnel: w1053 -> [_ w1059]
                            tunnel: w1053 -> [_ w1058]
                            frame False {
                            }
                            frame True {
                              n997 = for {
                                tunnel: w1060 -> [_] mode=indexing
                                tunnel: w1059 -> [w1078]
                                tunnel: w1058 -> [w1077]
                                # "实时数据的大小"
                                n998 = Wait (ms)(milliseconds to wait=u32 500 ("等待时间（毫秒）")) -> ()  [unwired: 1 out]
                                n999 = global write "全局 实时数据参数.vi" "实时数据参数"("水样测试" ("实时数据参数")) -> ()
                                n1000 = Get Date/Time In Seconds() -> (seconds since 1Jan1904=w1071:timestamp)
                                n1001 = Format Date/Time String(time format string (%c)="%Y%m%d%H%M%S%3u" ("时间格式字符串(%c)"), seconds (now)=w1071) -> (date/time string=w1072:string)  [unwired: 1 in]
                                n1002 = Search and Replace String(input string=w1072, search string="." ("搜索字符串")) -> (result string=w1074:string)  [unwired: 6 in, 3 out]
                                n1003 = local read "MN"() -> (w1066:string)
                                n1004 = local read "PW"() -> (w1065:string)
                                n1005 = local read "数据发送通道"() -> (w1064:enum16{"TCP", "VISA"})
                                n1006 = call "数据编码.vi"("table输入"="小时数据" ("新元素/子数组"), "QN"=w1074, "MN"=w1066, "PW"=w1065) -> ("通讯包字符串"=w1076:string)  [unwired: 10 in, 1 out]
                                n1007 = Build Array(w1076) -> (w1068:string[])
                                n1008 = local write "发送报文显示"(w1076) -> ()
                                n1009 = call "VISATCP组合选择发送.vi"("数据发送通道"=w1064, "命令"="write", "写入缓冲区"=w1076) -> ()  [unwired: 9 in, 4 out]
                                n1010 = call "发送数据记录到文档(子VI).vi"("数组"=w1068) -> ()  [unwired: 9 in, 1 out]
                                n1011 = local read "判断数据反馈"() -> (w1062:bool)
                                n1012 = case shown="真" w1062 {
                                tunnel: [_ w1101] -> w1075
                                tunnel: w1076 -> [_ w1100]
                                tunnel: w1078 -> [_ w1099]
                                frame False {
                                }
                                frame True {
                                n1013 = case shown="0, 默认" w1099 {
                                tunnel: [w1103 _] -> w1101
                                tunnel: w1100 -> [w1102 _]
                                frame 0, Default {
                                n1014 = Empty String/Path?(string/path=w1102) -> (empty?=w1104:bool)
                                n1015 = case shown="假" w1104 {
                                tunnel: [w1107 _] -> w1103
                                tunnel: w1102 -> [w1106 _]
                                frame False {
                                n1016 = local read "数据发送通道"() -> (w1105:enum16{"TCP", "VISA"})
                                n1017 = call "数据补发判定有限循环.vi"("数据输入"=w1106, "数据发送通道"=w1105) -> ("error out"=w1107:errorcluster)  [unwired: 9 in]
                                }
                                frame True {
                                }
                                }
                                }
                                frame 14..17 {
                                }
                                }
                                }
                                }
                                n1018 = local read "2011发送"() -> (w1061:bool)
                                n1019 = case shown="真" w1061 {
                                tunnel: w1077 -> [_ w1091]
                                tunnel: w1075 -> [_ w1090]
                                frame False {
                                }
                                frame True {
                                n1020 = local read "MN"() -> (w1085:string)
                                n1021 = local read "PW"() -> (w1084:string)
                                n1022 = global write "全局 实时数据参数.vi" "实时数据参数"("水样测试" ("实时数据参数")) -> ()
                                n1023 = call "数据编码.vi"("table输入"="实时数据" ("新元素/子数组"), "错误常量 2"=w1090, "MN"=w1085, "PW"=w1084) -> ("通讯包字符串"=w1089:string)  [unwired: 10 in, 1 out]
                                n1024 = Build Array(w1089) -> (w1087:string[])
                                n1025 = local read "数据发送通道"() -> (w1083:enum16{"TCP", "VISA"})
                                n1026 = local write "发送报文显示"(w1089) -> ()
                                n1027 = call "发送数据记录到文档(子VI).vi"("数组"=w1087) -> ()  [unwired: 9 in, 1 out]
                                n1028 = call "VISATCP组合选择发送.vi"("数据发送通道"=w1083, "命令"="write", "写入缓冲区"=w1089) -> ("错误输出"=w1088:errorcluster)  [unwired: 9 in, 3 out]
                                n1029 = local read "判断数据反馈"() -> (w1080:bool)
                                n1030 = case shown="真" w1080 {
                                tunnel: w1089 -> [_ w1094]
                                tunnel: w1088 -> [_ w1093]
                                tunnel: w1091 -> [_ w1092]
                                frame False {
                                }
                                frame True {
                                n1031 = case shown="0, 默认" w1092 {
                                tunnel: w1094 -> [w1098 _]
                                tunnel: w1093 -> [w1097 _]
                                frame 0, Default {
                                n1032 = local read "数据发送通道"() -> (w1095:enum16{"TCP", "VISA"})
                                n1033 = call "数据补发判定有限循环.vi"("错误输入（无错误）"=w1097, "数据输入"=w1098, "数据发送通道"=w1095) -> ("error out"=w1096:errorcluster)  [unwired: 8 in]
                                n1034 = local write "错误输出"(w1096) -> ()
                                }
                                frame 14..17 {
                                }
                                }
                                }
                                }
                                }
                                }
                              }
                            }
                          }
                        }
                        frame #2 {
                          n1035 = global read "全局 数据发送重叠.vi" "数据接收超时指示灯"() -> (w1108:bool)
                          n1036 = Not(x=w1108) -> (.not. x?=w1109:bool)
                          n1037 = Compound Arithmetic op=AND ("复合运算")(w1109, w1111) -> (w1110:bool)
                          n1038 = case shown="真" w1110 {
                            tunnel: w1113 -> [_ w1117]
                            tunnel: w1112 -> [_ w1127]
                            tunnel: w1114 -> [_ w1118]
                            frame False {
                            }
                            frame True {
                              n1039 = call "日期时间字符串转换分钟数加一.vi"("data[0]"=w1117) -> ("日期/时间字符串"=w1115:string)  [unwired: 10 in]
                              n1040 = call "时间日期字符串至时间标识转换.vi"("时间日期字符串"=w1115) -> ("时间标识"=w1116:timestamp)  [unwired: 10 in]
                              n1041 = call <vilib>:"Application Directory.vi"() -> ("Application Directory"=w1119:path)
                              n1042 = case shown="3" w1127 {
                                tunnel: w1115 -> [w1128 w1129 w1130 w1131 w1132 w1133 w1134 w1135 w1136 w1137 w1138 w1139 w1140 w1141 w1142 w1143 w1144 w1145]
                                frame 0, Default {
                                n1043 = global write "全局 水样时间.vi" "time1"(w1128) -> ()
                                }
                                frame 1 {
                                n1044 = global write "全局 水样时间.vi" "time2"(w1129) -> ()
                                }
                                frame 2 {
                                n1045 = global write "全局 水样时间.vi" "time3"(w1130) -> ()
                                }
                                frame 3 {
                                n1046 = global write "全局 水样时间.vi" "time4"(w1131) -> ()
                                }
                                frame 4 {
                                n1047 = global write "全局 水样时间.vi" "time5"(w1132) -> ()
                                }
                                frame 5 {
                                n1048 = global write "全局 水样时间.vi" "time6"(w1133) -> ()
                                }
                                frame 6 {
                                n1049 = global write "全局 水样时间.vi" "time7"(w1134) -> ()
                                }
                                frame 7 {
                                n1050 = global write "全局 水样时间.vi" "time8"(w1135) -> ()
                                }
                                frame 8 {
                                n1051 = global write "全局 水样时间.vi" "time9"(w1136) -> ()
                                }
                                frame 9 {
                                n1052 = global write "全局 水样时间.vi" "time10"(w1137) -> ()
                                }
                                frame 10 {
                                n1053 = global write "全局 水样时间.vi" "time11"(w1138) -> ()
                                }
                                frame 11 {
                                n1054 = global write "全局 水样时间.vi" "time12"(w1139) -> ()
                                }
                                frame 12 {
                                n1055 = global write "全局 水样时间.vi" "time13"(w1140) -> ()
                                }
                                frame 13 {
                                n1056 = global write "全局 水样时间.vi" "time14"(w1141) -> ()
                                }
                                frame 14 {
                                n1057 = global write "全局 水样时间.vi" "time15"(w1142) -> ()
                                }
                                frame 15 {
                                n1058 = global write "全局 水样时间.vi" "time16"(w1143) -> ()
                                }
                                frame 16 {
                                n1059 = global write "全局 水样时间.vi" "time17"(w1144) -> ()
                                }
                                frame 17 {
                                n1060 = global write "全局 水样时间.vi" "time18"(w1145) -> ()
                                }
                              }
                              n1061 = Build Path(base path=w1119, name or relative path="data\\Set.ini" ("名称或相对路径")) -> (appended path=w1121:path)
                              n1062 = call <vilib>:"Open Config Data.vi"("configuration file path"=w1121) -> ("error out"=w1123:errorcluster, "refnum"=w1122:T8)  [unwired: 8 in, 1 out]
                              n1063 = local write "数据发送起始时间"(w1116) -> ()
                              n1064 = call-poly <vilib>:"Write Key.vi"("section"="线程一数据搜索起始时间", "error in (no error)"=w1123, "value"=w1115, "key"=w1118, "refnum"=w1122) -> ("error out"=w1125:errorcluster, "refnum out"=w1124:T8)  [unwired: 4 in, 1 out]
                              n1065 = call <vilib>:"Close Config Data.vi"("error in (no error)"=w1125, "refnum"=w1124) -> ()  [unwired: 8 in, 2 out]
                            }
                          }
                        }
                      }
                    }
                  }
                }
                "实时小时数据上传" <- w833
              }
              frame #1 {
                w1200 = FALSE ("小时数据上传")
                n1066 = local write "实时小时数据上传"(w1200) -> ()
                n1067 = global write "全局 数据发送重叠.vi" "主动上报数据中"(w1200) -> ()
              }
            }
          }
          frame True {
            # "数据整点触发，整条发送"
          }
        }
      }
    }
  }
  n1068 = while {
    stop <- FALSE stop-if-true
    # "数据整点触发，整条发送；数据自动重发设置"
    n1069 = global read "断电保存全局.vi" "数据组合发送"() -> (w1203:bool)
    n1070 = case shown="真" "每周自动重发" {
      frame False {
      }
      frame True {
        (unwired) T1."00点"
        (unwired) T2."关闭"
        # "自动重发水样数据"
        n1071 = Get Date/Time In Seconds() -> (seconds since 1Jan1904=w1218:timestamp)
        n1072 = Seconds To Date/Time(time stamp (now)=w1218) -> (date time rec=w1212:T9)  [unwired: 1 in]
        n1073 = Unbundle By Name(w1212) -> ("天数（周）"=w1217:i32, "时"=w1207:i32, "分"=w1216:i32)
        n1074 = Equal To 0?(x=w1216) -> (x = 0?=w1213:bool)
        n1075 = Equal?(x=w1217, y="重发日期") -> (x = y?=w1215:bool)
        n1076 = Equal?(x=w1207, y="重发时间") -> (x = y?=w1214:bool)
        n1077 = Compound Arithmetic op=AND ("复合运算")(w1215, w1214, w1213) -> (w1211:bool)
        n1078 = call <vilib>:"Boolean Crossing PtByPt.vi"("direction"=enum16{"either", "false-true", "true-false"}."false-true", "input"=w1211) -> ("crossing"=w1210:bool)  [unwired: 1 in]
        n1079 = case shown="真" w1210 {
          tunnel: w1212 -> [_ w1221]
          frame False {
          }
          frame True {
            n1080 = local read "参数数值"() -> (w1219:T5)
            n1081 = Unbundle By Name(w1221) -> ("日"=w1224:i32)
            n1082 = Cluster To Array(cluster=w1219) -> (array=w1226:bool[])
            n1083 = Subtract(x=w1224, y=7) -> (x-y=w1222:i32)
            n1084 = Bundle By Name(cluster=w1221, "日"=w1222) -> (w1225:T9)
            n1085 = Date/Time To Seconds(2:w1225) -> (0:w1220:timestamp)  [unwired: 1 in]
            n1086 = for {
              tunnel: w1226 -> [_] mode=indexing
              tunnel: w1220 -> [w1227]
              i -> [w1228]
              n1087 = Format Date/Time String(time format string (%c)="%Y/%m/%d %H:%M:%S" ("时间格式字符串(%c)"), seconds (now)=w1227) -> (date/time string=w1229:string)  [unwired: 1 in]
              n1088 = case shown="16" w1228 {
                tunnel: w1229 -> [w1231 w1232 w1233 w1234 w1235 w1236 w1237 w1238 w1239 w1240 w1241 w1242 w1243 w1244 w1245 w1246 w1247 w1248]
                frame 0, Default {
                  n1089 = global write "全局 水样时间.vi" "time1"(w1231) -> ()
                }
                frame 1 {
                  n1090 = global write "全局 水样时间.vi" "time2"(w1232) -> ()
                }
                frame 2 {
                  n1091 = global write "全局 水样时间.vi" "time3"(w1233) -> ()
                }
                frame 3 {
                  n1092 = global write "全局 水样时间.vi" "time4"(w1234) -> ()
                }
                frame 4 {
                  n1093 = global write "全局 水样时间.vi" "time5"(w1235) -> ()
                }
                frame 5 {
                  n1094 = global write "全局 水样时间.vi" "time6"(w1236) -> ()
                }
                frame 6 {
                  n1095 = global write "全局 水样时间.vi" "time7"(w1237) -> ()
                }
                frame 7 {
                  n1096 = global write "全局 水样时间.vi" "time8"(w1238) -> ()
                }
                frame 8 {
                  n1097 = global write "全局 水样时间.vi" "time9"(w1239) -> ()
                }
                frame 9 {
                  n1098 = global write "全局 水样时间.vi" "time10"(w1240) -> ()
                }
                frame 10 {
                  n1099 = global write "全局 水样时间.vi" "time11"(w1241) -> ()
                }
                frame 11 {
                  n1100 = global write "全局 水样时间.vi" "time12"(w1242) -> ()
                }
                frame 12 {
                  n1101 = global write "全局 水样时间.vi" "time13"(w1243) -> ()
                }
                frame 13 {
                  n1102 = global write "全局 水样时间.vi" "time14"(w1244) -> ()
                }
                frame 14 {
                  n1103 = global write "全局 水样时间.vi" "time15"(w1245) -> ()
                }
                frame 15 {
                  n1104 = global write "全局 水样时间.vi" "time16"(w1246) -> ()
                }
                frame 16 {
                  n1105 = global write "全局 水样时间.vi" "time17"(w1247) -> ()
                }
                frame 17 {
                  n1106 = global write "全局 水样时间.vi" "time18"(w1248) -> ()
                }
              }
            }
          }
        }
      }
    }
    n1107 = case shown="真" w1203 {
      frame False {
      }
      frame True {
        n1108 = Get Date/Time In Seconds() -> (seconds since 1Jan1904=w1256:timestamp)
        n1109 = Seconds To Date/Time(time stamp (now)=w1256) -> (date time rec=w1257:T9)  [unwired: 1 in]
        n1110 = global read "断电保存全局.vi" "数据重发"() -> (w1249:bool)
        n1111 = Unbundle By Name(w1257) -> ("分"=w1255:i32)
        n1112 = Equal?(x=w1255, y=0) -> (x = y?=w1253:bool)
        n1113 = call <vilib>:"Boolean Crossing PtByPt.vi"("direction"=enum16{"either", "false-true", "true-false"}."false-true", "input"=w1253) -> ("crossing"=w1251:bool)  [unwired: 1 in]
        n1114 = Or(x=w1249, y=w1251) -> (x .or. y?=w1250:bool)
        n1115 = case shown="真" w1250 {
          frame False {
            n1116 = global write "全局 数据发送重叠.vi" "主动上报数据中"(FALSE ("主动上报数据中")) -> ()
          }
          frame True {
            n1117 = local read "数据发送通道"() -> (w1261:enum16{"TCP", "VISA"})
            n1118 = local read "MN"() -> (w1260:string)
            n1119 = local read "PW"() -> (w1259:string)
            n1120 = call "数据全参数一起发送整点触发.vi"("数据发送通道"=w1261, "PW"=w1259, "MN"=w1260) -> ()  [unwired: 8 in]
          }
        }
      }
    }
    n1121 = Wait (ms)(milliseconds to wait=u32 1000 ("等待时间（毫秒）")) -> ()  [unwired: 1 out]
  }
  n1122 = Obtain Queue(name (unnamed)="STEP" ("名称（未命名）"), element data type=T6."初始化" ("枚举")) -> (queue out=w49:refnum<queue>)  [unwired: 3 in, 2 out]
  n1123 = Insert Into Array(array=string[] [] ("tables"), index=0 ("索引"), new element="实时数据" ("新元素/子数组")) -> (w52:string[])
  n1124 = Enqueue Element(queue=w49, element=T6."初始化" ("元素")) -> (queue out=w54:refnum<queue>)  [unwired: 2 in, 2 out]
  "主队列输出" <- w54
  n1125 = Array Size(array=w52) -> (size(s)=w50:i32)
  n1126 = vi-ref "数据传输系统.lvlib:最小窗口后台运行(子VI).vi"() -> (w29:refnum<vi>)
  n1127 = while {
    stop <- FALSE stop-if-true
    # "定期释放缓存"
    n1128 = Wait (ms)(milliseconds to wait=u32 600000 ("等待时间（毫秒）")) -> ()  [unwired: 1 out]
    n1129 = dll-call lib="PTH2gabs F\tgitkrakenCC<平台数采程序 - 通用（小时数据单参数传）XINdataFreeMem.dll" fn="FreeMem"() -> ()  [unwired: 4 in, 2 out]
  }
  n1130 = while {
    stop <- FALSE stop-if-true
    n1131 = event shown="[1] \"站点名称\", \"站点设备\", \"IP\", \"PORT\", \"MN\", \"PW\", \"VISA resource name\", \"baud rate\": 值改变" {
      selector: _ -> [_ _ _ _ _ _ _ _ _ _ _ _ _ _ _ _ _ _]
      dyn-events: _ -> [_ _ _ _ _ _ _ _ _ _ _ _ _ _ _ _ _ _]
      timeout: _ -> [_ _ _ _ _ _ _ _ _ _ _ _ _ _ _ _ _ _]
      event Timeout {
        n1132 = event-data() -> ()  [unwired: 1 in, 2 out]
      }
      event "站点名称", "站点设备", "IP", "PORT", "MN", "PW", "VISA resource name", "baud rate": Value Change {
        w1267 = "线程一自主部署站点保存"
        # "TCP服务器端口掉线"
        n1133 = event-data() -> ()  [unwired: 1 in, 6 out]
        n1134 = call <vilib>:"Application Directory.vi"() -> ("Application Directory"=w1309:path)
        n1135 = local read "站点名称"() -> (w1288:string)
        n1136 = Build Path(base path=w1309, name or relative path="data\\Set.ini" ("名称或相对路径")) -> (appended path=w1307:path)
        n1137 = call <vilib>:"Open Config Data.vi"("configuration file path"=w1307) -> ("error out"=w1305:errorcluster, "refnum"=w1306:T8)  [unwired: 8 in, 1 out]
        n1138 = local read "站点设备"() -> (w1287:string)
        n1139 = call-poly <vilib>:"Write Key.vi"("section"=w1267, "error in (no error)"=w1305, "value"=w1288, "key"="站点名称", "refnum"=w1306) -> ("error out"=w1302:errorcluster, "refnum out"=w1303:T8)  [unwired: 4 in, 1 out]
        n1140 = call-poly <vilib>:"Write Key.vi"("section"=w1267, "error in (no error)"=w1302, "value"=w1287, "key"="站点设备", "refnum"=w1303) -> ("error out"=w1299:errorcluster, "refnum out"=w1300:T8)  [unwired: 4 in, 1 out]
        n1141 = local read "IP"() -> (w1286:string)
        n1142 = call-poly <vilib>:"Write Key.vi"("section"=w1267, "error in (no error)"=w1299, "value"=w1286, "key"="IP", "refnum"=w1300) -> ("error out"=w1297:errorcluster, "refnum out"=w1298:T8)  [unwired: 4 in, 1 out]
        n1143 = local read "PORT"() -> (w1285:string)
        n1144 = call-poly <vilib>:"Write Key.vi"("section"=w1267, "error in (no error)"=w1297, "value"=w1285, "key"="PORT", "refnum"=w1298) -> ("error out"=w1295:errorcluster, "refnum out"=w1296:T8)  [unwired: 4 in, 1 out]
        n1145 = local read "MN"() -> (w1279:string)
        n1146 = call-poly <vilib>:"Write Key.vi"("section"=w1267, "error in (no error)"=w1295, "value"=w1279, "key"="MN", "refnum"=w1296) -> ("error out"=w1280:errorcluster, "refnum out"=w1283:T8)  [unwired: 4 in, 1 out]
        n1147 = local read "PW"() -> (w1281:string)
        n1148 = call-poly <vilib>:"Write Key.vi"("section"=w1267, "error in (no error)"=w1280, "value"=w1281, "key"="PW", "refnum"=w1283) -> ("error out"=w1268:errorcluster, "refnum out"=w1269:T8)  [unwired: 4 in, 1 out]
        n1149 = local read "VISA resource name"() -> (w1275:refnum<visa-resource-name>)
        n1150 = local read "主队列输出"() -> (w1294:refnum<queue>)
        n1151 = call-poly <vilib>:"Write Key.vi"("section"=w1267, "error in (no error)"=w1268, "value"=w1275, "key"="VISA", "refnum"=w1269) -> ("error out"=w1274:errorcluster, "refnum out"=w1271:T8)  [unwired: 4 in, 1 out]
        n1152 = local read "baud rate"() -> (w1273:u32)
        n1153 = Flush Queue(queue=w1294) -> (queue out=w1293:refnum<queue>)  [unwired: 1 in, 2 out]
        n1154 = call-poly <vilib>:"Write Key.vi"("section"=w1267, "error in (no error)"=w1274, "value"=w1273, "key"="BAUDRATE", "refnum"=w1271) -> ("error out"=w1265:errorcluster, "refnum out"=w1266:T8)  [unwired: 4 in, 1 out]
        n1155 = local read "数据发送通道"() -> (w1278:enum16{"TCP", "VISA"})
        n1156 = call <vilib>:"Close Config Data.vi"("error in (no error)"=w1265, "refnum"=w1266) -> ()  [unwired: 8 in, 2 out]
        n1157 = call "VISATCP组合选择发送.vi"("数据发送通道"=w1278, "命令"="close") -> ("错误输出"=w1276:errorcluster)  [unwired: 10 in, 3 out]
        n1158 = Enqueue Element(queue=w1293, element=T6."初始化" ("元素"), timeout in ms (-1)=1000 ("超时毫秒(-1)")) -> ()  [unwired: 1 in, 3 out]
        n1159 = call <vilib>:"Clear Errors.vi"("error in (no error)"=w1276) -> ()  [unwired: 5 in, 2 out]
      }
      event "确定": Value Change {
        w1314 = "线程一自主部署站点保存"
        # "TCP服务器端口掉线"
        n1160 = event-data() -> ()  [unwired: 1 in, 6 out]
        n1161 = call <vilib>:"Application Directory.vi"() -> ("Application Directory"=w1347:path)
        n1162 = local read "站点名称"() -> (w1342:string)
        n1163 = Build Path(base path=w1347, name or relative path="data\\Set.ini" ("名称或相对路径")) -> (appended path=w1345:path)
        n1164 = call <vilib>:"Open Config Data.vi"("configuration file path"=w1345) -> ("error out"=w1343:errorcluster, "refnum"=w1344:T8)  [unwired: 8 in, 1 out]
        n1165 = local read "站点设备"() -> (w1337:string)
        n1166 = call-poly <vilib>:"Write Key.vi"("section"=w1314, "error in (no error)"=w1343, "value"=w1342, "key"="站点名称", "refnum"=w1344) -> ("error out"=w1339:errorcluster, "refnum out"=w1340:T8)  [unwired: 4 in, 1 out]
        n1167 = call-poly <vilib>:"Write Key.vi"("section"=w1314, "error in (no error)"=w1339, "value"=w1337, "key"="站点设备", "refnum"=w1340) -> ("error out"=w1335:errorcluster, "refnum out"=w1336:T8)  [unwired: 4 in, 1 out]
        n1168 = local read "IP"() -> (w1330:string)
        n1169 = local read "PORT"() -> (w1329:string)
        n1170 = call-poly <vilib>:"Write Key.vi"("section"=w1314, "error in (no error)"=w1335, "value"=w1330, "key"="IP", "refnum"=w1336) -> ("error out"=w1333:errorcluster, "refnum out"=w1334:T8)  [unwired: 4 in, 1 out]
        n1171 = call-poly <vilib>:"Write Key.vi"("section"=w1314, "error in (no error)"=w1333, "value"=w1329, "key"="PORT", "refnum"=w1334) -> ("error out"=w1325:errorcluster, "refnum out"=w1326:T8)  [unwired: 4 in, 1 out]
        n1172 = local read "MN"() -> (w1322:string)
        n1173 = call-poly <vilib>:"Write Key.vi"("section"=w1314, "error in (no error)"=w1325, "value"=w1322, "key"="MN", "refnum"=w1326) -> ("error out"=w1323:errorcluster, "refnum out"=w1324:T8)  [unwired: 4 in, 1 out]
        n1174 = local read "PW"() -> (w1321:string)
        n1175 = call-poly <vilib>:"Write Key.vi"("section"=w1314, "error in (no error)"=w1323, "value"=w1321, "key"="PW", "refnum"=w1324) -> ("error out"=w1319:errorcluster, "refnum out"=w1320:T8)  [unwired: 4 in, 1 out]
        n1176 = call <vilib>:"Close Config Data.vi"("error in (no error)"=w1319, "refnum"=w1320) -> ("error out"=w1313:errorcluster)  [unwired: 8 in, 1 out]
        n1177 = local read "主队列输出"() -> (w1318:refnum<queue>)
        n1178 = local read "数据发送通道"() -> (w1312:enum16{"TCP", "VISA"})
        n1179 = call "VISATCP组合选择发送.vi"("数据发送通道"=w1312, "命令"="close") -> ("错误输出"=w1310:errorcluster)  [unwired: 10 in, 3 out]
        n1180 = Flush Queue(queue=w1318) -> (queue out=w1317:refnum<queue>)  [unwired: 1 in, 2 out]
        n1181 = case shown="错误" w1313 {
          frame No Error {
            n1182 = One Button Dialog(message="保存成功" ("消息"), button name ("OK")="确定" ("按钮名称（“确定”）")) -> ()  [unwired: 1 out]
          }
          frame Error {
            n1183 = One Button Dialog(message="保存失败" ("消息"), button name ("OK")="确定" ("按钮名称（“确定”）")) -> ()  [unwired: 1 out]
          }
        }
        n1184 = call <vilib>:"Clear Errors.vi"("error in (no error)"=w1310) -> ()  [unwired: 5 in, 2 out]
        n1185 = Enqueue Element(queue=w1317, element=T6."初始化" ("元素"), timeout in ms (-1)=1000 ("超时毫秒(-1)")) -> ()  [unwired: 1 in, 3 out]
      }
      event "参数配置": Value Change {
        n1186 = event-data() -> ()  [unwired: 1 in, 6 out]
        n1187 = property on="窗格" class="Pane"("Origin"=T11 {"Horizontal"=0, "Vertical"=1000} ("原点")) -> ()  [unwired: 2 in, 2 out]
      }
      event "返回": Value Change {
        n1188 = event-data() -> ()  [unwired: 1 in, 6 out]
        n1189 = property on="窗格" class="Pane"("Origin"=T11 {"Horizontal"=0, "Vertical"=0} ("原点")) -> ()  [unwired: 2 in, 2 out]
      }
      event "系统编码选择框": Value Change {
        n1190 = event-data() -> ()  [unwired: 1 in, 6 out]
        n1191 = call <vilib>:"Application Directory.vi"() -> ("Application Directory"=w1362:path)
        n1192 = Build Path(base path=w1362, name or relative path="data\\Set.ini" ("名称或相对路径")) -> (appended path=w1363:path)
        n1193 = call <vilib>:"Open Config Data.vi"("configuration file path"=w1363) -> ("error out"=w1359:errorcluster, "refnum"=w1360:T8)  [unwired: 8 in, 1 out]
        n1194 = call-poly <vilib>:"Write Key.vi"("section"="系统编码选择", "error in (no error)"=w1359, "value"="系统编码选择框", "key"="系统编码", "refnum"=w1360) -> ("error out"=w1357:errorcluster, "refnum out"=w1358:T8)  [unwired: 4 in, 1 out]
        n1195 = call <vilib>:"Close Config Data.vi"("error in (no error)"=w1357, "refnum"=w1358) -> ()  [unwired: 8 in, 2 out]
      }
      event "数据发送通道": Value Change {
        w1364 = "数据发送通道"
        n1196 = event-data() -> ()  [unwired: 1 in, 6 out]
        n1197 = local read "数据发送通道"() -> (w1365:enum16{"TCP", "VISA"})
        n1198 = call <vilib>:"Application Directory.vi"() -> ("Application Directory"=w1371:path)
        n1199 = Build Path(base path=w1371, name or relative path="data\\Set.ini" ("名称或相对路径")) -> (appended path=w1372:path)
        n1200 = call <vilib>:"Open Config Data.vi"("configuration file path"=w1372) -> ("error out"=w1368:errorcluster, "refnum"=w1369:T8)  [unwired: 8 in, 1 out]
        n1201 = call-poly <vilib>:"Write Key.vi"("section"=w1364, "error in (no error)"=w1368, "value"=w1365, "key"=w1364, "refnum"=w1369) -> ("error out"=w1366:errorcluster, "refnum out"=w1367:T8)  [unwired: 4 in, 1 out]
        n1202 = call <vilib>:"Close Config Data.vi"("error in (no error)"=w1366, "refnum"=w1367) -> ()  [unwired: 8 in, 2 out]
      }
      event "数据发送协议": Value Change {
        w1374 = "数据发送协议"
        n1203 = event-data() -> ()  [unwired: 1 in, 6 out]
        n1204 = call <vilib>:"Application Directory.vi"() -> ("Application Directory"=w1380:path)
        n1205 = Build Path(base path=w1380, name or relative path="data\\Set.ini" ("名称或相对路径")) -> (appended path=w1381:path)
        n1206 = call <vilib>:"Open Config Data.vi"("configuration file path"=w1381) -> ("error out"=w1377:errorcluster, "refnum"=w1378:T8)  [unwired: 8 in, 1 out]
        n1207 = call-poly <vilib>:"Write Key.vi"("section"=w1374, "error in (no error)"=w1377, "value"="数据发送协议", "key"=w1374, "refnum"=w1378) -> ("error out"=w1375:errorcluster, "refnum out"=w1376:T8)  [unwired: 4 in, 1 out]
        n1208 = call <vilib>:"Close Config Data.vi"("error in (no error)"=w1375, "refnum"=w1376) -> ()  [unwired: 8 in, 2 out]
      }
      event "判断数据反馈", "2011发送", "日志、参数发送", "数据组合发送": Value Change {
        n1209 = event-data() -> ()  [unwired: 1 in, 6 out]
        n1210 = flat-sequence {
          frame #0 {
            n1211 = global write "断电保存全局.vi" "日志、参数发送"("日志、参数发送") -> ()
            n1212 = global write "断电保存全局.vi" "判断数据反馈"("判断数据反馈") -> ()
            n1213 = global write "断电保存全局.vi" "2011发送"("2011发送") -> ()
            n1214 = global write "断电保存全局.vi" "数据组合发送"("数据组合发送") -> ()
          }
          frame #1 {
            n1215 = call <vilib>:"Application Directory.vi"() -> ("Application Directory"=w1386:path)
            n1216 = Build Path(base path=w1386, name or relative path="data\\sys.ini" ("名称或相对路径")) -> (appended path=w1388:path)
            n1217 = call <vilib>:"Open Config Data.vi"("configuration file path"=w1388) -> ("error out"=w1392:errorcluster, "refnum"=w1389:T8)  [unwired: 8 in, 1 out]
            n1218 = vi-ref "断电保存全局.vi"() -> (w1390:refnum<vi>)
            n1219 = call <userlib>:"Write Panel to INI__ogtk.vi"("error in (no error)"=w1392, "VI ref"=w1390, "refnum"=w1389) -> ("error out"=w1393:errorcluster, "refnum out"=w1391:T8)  [unwired: 7 in]
            n1220 = call <vilib>:"Close Config Data.vi"("error in (no error)"=w1393, "refnum"=w1391) -> ("error out"=w1398:errorcluster, "file path"=w1399:path)  [unwired: 8 in]
            n1221 = Open/Create/Replace File(file path (use dialog)=w1399, error in=w1398) -> (refnum out=w1395:refnum<file>, error out=w1394:errorcluster)  [unwired: 4 in, 1 out]
            n1222 = Flush File(refnum=w1395, error in=w1394) -> (refnum out=w1396:refnum<file>, error out=w1397:errorcluster)
            n1223 = Close File(refnum=w1396, error in=w1397) -> ()  [unwired: 2 out]
          }
        }
      }
      event "每周自动重发": Value Change {
        n1224 = event-data() -> ()  [unwired: 1 in, 6 out]
        n1225 = call <vilib>:"Application Directory.vi"() -> ("Application Directory"=w1408:path)
        n1226 = Build Path(base path=w1408, name or relative path="data\\Set.ini" ("名称或相对路径")) -> (appended path=w1409:path)
        n1227 = local read "每周自动重发"() -> (w1400:bool)
        n1228 = call <vilib>:"Open Config Data.vi"("configuration file path"=w1409) -> ("error out"=w1405:errorcluster, "refnum"=w1406:T8)  [unwired: 8 in, 1 out]
        n1229 = call-poly <vilib>:"Write Key.vi"("section"="线程一数据重发功能", "error in (no error)"=w1405, "value"=w1400, "key"="重发功能", "refnum"=w1406) -> ("error out"=w1403:errorcluster, "refnum out"=w1404:T8)  [unwired: 4 in, 1 out]
        n1230 = call <vilib>:"Close Config Data.vi"("error in (no error)"=w1403, "refnum"=w1404) -> ()  [unwired: 8 in, 2 out]
      }
      event "重发日期": Value Change {
        n1231 = event-data() -> ()  [unwired: 1 in, 6 out]
        n1232 = call <vilib>:"Application Directory.vi"() -> ("Application Directory"=w1418:path)
        n1233 = Build Path(base path=w1418, name or relative path="data\\Set.ini" ("名称或相对路径")) -> (appended path=w1419:path)
        n1234 = local read "重发日期"() -> (w1410:T2)
        n1235 = call <vilib>:"Open Config Data.vi"("configuration file path"=w1419) -> ("error out"=w1415:errorcluster, "refnum"=w1416:T8)  [unwired: 8 in, 1 out]
        n1236 = call-poly <vilib>:"Write Key.vi"("section"="线程一数据重发功能", "error in (no error)"=w1415, "value"=w1410, "key"="重发日期", "refnum"=w1416) -> ("error out"=w1413:errorcluster, "refnum out"=w1414:T8)  [unwired: 4 in, 1 out]
        n1237 = call <vilib>:"Close Config Data.vi"("error in (no error)"=w1413, "refnum"=w1414) -> ()  [unwired: 8 in, 2 out]
      }
      event "重发时间": Value Change {
        n1238 = event-data() -> ()  [unwired: 1 in, 6 out]
        n1239 = call <vilib>:"Application Directory.vi"() -> ("Application Directory"=w1428:path)
        n1240 = Build Path(base path=w1428, name or relative path="data\\Set.ini" ("名称或相对路径")) -> (appended path=w1429:path)
        n1241 = local read "重发时间"() -> (w1420:T1)
        n1242 = call <vilib>:"Open Config Data.vi"("configuration file path"=w1429) -> ("error out"=w1425:errorcluster, "refnum"=w1426:T8)  [unwired: 8 in, 1 out]
        n1243 = call-poly <vilib>:"Write Key.vi"("section"="线程一数据重发功能", "error in (no error)"=w1425, "value"=w1420, "key"="重发时间", "refnum"=w1426) -> ("error out"=w1423:errorcluster, "refnum out"=w1424:T8)  [unwired: 4 in, 1 out]
        n1244 = call <vilib>:"Close Config Data.vi"("error in (no error)"=w1423, "refnum"=w1424) -> ()  [unwired: 8 in, 2 out]
      }
      event "确定更改起始时间": Value Change {
        n1245 = event-data() -> ()  [unwired: 1 in, 6 out]
        n1246 = local write "更改起始时间"(FALSE ("更改起始时间")) -> ()
        n1247 = Two Button Dialog(message="确定以当前设置时间作为数据索引起始时间？" ("消息")) -> (T button?=w1431:bool)  [unwired: 2 in]
        n1248 = case shown="真" w1431 {
          frame False {
          }
          frame True {
            n1249 = local read "参数数值"() -> (w1436:T5)
            n1250 = global write "断电保存全局.vi" "数据重发"(TRUE ("数据重发")) -> ()
            n1251 = Cluster To Array(cluster=w1436) -> (array=w1437:bool[])
            n1252 = for {
              tunnel: w1437 -> [_] mode=indexing
              tunnel: [w1447] -> w1435
              i -> [w1448]
              n1253 = Format Date/Time String(time format string (%c)="%Y/%m/%d %H:%M:%S" ("时间格式字符串(%c)"), seconds (now)="数据发送起始时间") -> (date/time string=w1447:string)  [unwired: 1 in]
              n1254 = global write "断电保存全局.vi" "数据重发时间戳"(w1447) -> ()
              n1255 = case shown="0, 默认" w1448 {
                tunnel: w1447 -> [w1451 w1452 w1453 w1454 w1455 w1456 w1457 w1458 w1459 w1460 w1461 w1462 w1463 w1464 w1465 w1466 w1467 w1468]
                frame 0, Default {
                  n1256 = global write "全局 水样时间.vi" "time1"(w1451) -> ()
                }
                frame 1 {
                  n1257 = global write "全局 水样时间.vi" "time2"(w1452) -> ()
                }
                frame 2 {
                  n1258 = global write "全局 水样时间.vi" "time3"(w1453) -> ()
                }
                frame 3 {
                  n1259 = global write "全局 水样时间.vi" "time4"(w1454) -> ()
                }
                frame 4 {
                  n1260 = global write "全局 水样时间.vi" "time5"(w1455) -> ()
                }
                frame 5 {
                  n1261 = global write "全局 水样时间.vi" "time6"(w1456) -> ()
                }
                frame 6 {
                  n1262 = global write "全局 水样时间.vi" "time7"(w1457) -> ()
                }
                frame 7 {
                  n1263 = global write "全局 水样时间.vi" "time8"(w1458) -> ()
                }
                frame 8 {
                  n1264 = global write "全局 水样时间.vi" "time9"(w1459) -> ()
                }
                frame 9 {
                  n1265 = global write "全局 水样时间.vi" "time10"(w1460) -> ()
                }
                frame 10 {
                  n1266 = global write "全局 水样时间.vi" "time11"(w1461) -> ()
                }
                frame 11 {
                  n1267 = global write "全局 水样时间.vi" "time12"(w1462) -> ()
                }
                frame 12 {
                  n1268 = global write "全局 水样时间.vi" "time13"(w1463) -> ()
                }
                frame 13 {
                  n1269 = global write "全局 水样时间.vi" "time14"(w1464) -> ()
                }
                frame 14 {
                  n1270 = global write "全局 水样时间.vi" "time15"(w1465) -> ()
                }
                frame 15 {
                  n1271 = global write "全局 水样时间.vi" "time16"(w1466) -> ()
                }
                frame 16 {
                  n1272 = global write "全局 水样时间.vi" "time17"(w1467) -> ()
                }
                frame 17 {
                  n1273 = global write "全局 水样时间.vi" "time18"(w1468) -> ()
                }
              }
            }
            n1274 = global read "断电保存全局.vi" "数据组合发送"() -> (w1433:bool)
            n1275 = case shown="假" w1433 {
              tunnel: w1435 -> [w1438 _]
              frame False {
                n1276 = global write "全局 时间2.vi" "跨度核查索引起始时间"(w1438) -> ()
                n1277 = global write "全局 时间2.vi" "标样核查索引起始时间"(w1438) -> ()
                n1278 = global write "全局 时间2.vi" "零点核查索引起始时间"(w1438) -> ()
                n1279 = global write "全局 时间2.vi" "加标回收索引起始时间"(w1438) -> ()
                n1280 = for {
                  N: 5 -> [_]
                  tunnel: w1438 -> [w1440]
                  i -> [w1441]
                  n1281 = case shown="4" w1441 {
                    tunnel: w1440 -> [w1442 w1443 w1444 w1445 w1446]
                    frame 0, Default {
                      n1282 = global write "全局 时间2.vi" "氨氮跨度核查索引起始时间"(w1442) -> ()
                      n1283 = global write "全局 时间2.vi" "氨氮零点核查索引起始时间"(w1442) -> ()
                    }
                    frame 1 {
                      n1284 = global write "全局 时间2.vi" "总氮跨度核查索引起始时间"(w1443) -> ()
                      n1285 = global write "全局 时间2.vi" "总氮零点核查索引起始时间"(w1443) -> ()
                    }
                    frame 2 {
                      n1286 = global write "全局 时间2.vi" "总磷跨度核查索引起始时间"(w1444) -> ()
                      n1287 = global write "全局 时间2.vi" "总磷零点核查索引起始时间"(w1444) -> ()
                    }
                    frame 3 {
                      n1288 = global write "全局 时间2.vi" "CODMn跨度核查索引起始时间"(w1445) -> ()
                      n1289 = global write "全局 时间2.vi" "CODMn零点核查索引起始时间"(w1445) -> ()
                    }
                    frame 4 {
                      n1290 = global write "全局 时间2.vi" "CODCr跨度核查索引起始时间"(w1446) -> ()
                      n1291 = global write "全局 时间2.vi" "CODCr零点核查索引起始时间"(w1446) -> ()
                    }
                  }
                }
              }
              frame True {
              }
            }
          }
        }
      }
      event "开机启动": Value Change {
        n1292 = event-data() -> ("NewVal"=w1469:bool)  [unwired: 1 in, 5 out]
        n1293 = case shown="假" w1469 {
          frame False {
            n1294 = Two Button Dialog(message="是否删除开机启动" ("消息"), 1:"否" ("F按钮名称（“取消”）"), 2:"是" ("T按钮名称（“确定”）")) -> (T button?=w1470:bool)
            n1295 = case shown="真" w1470 {
              frame False {
              }
              frame True {
                n1296 = call <vilib>:"Application Directory.vi"() -> ("Application Directory"=w1475:path)
                n1297 = call "删除启动项.vi"("启动文件路径"=w1475) -> ("删除标记"=w1474:bool)  [unwired: 9 in, 1 out]
                n1298 = case shown="假" w1474 {
                  tunnel: ["删除开机启动失败" ("T按钮名称（“确定”）") "删除开机启动成功" ("T按钮名称（“确定”）")] -> w1476
                  frame False {
                  }
                  frame True {
                  }
                }
                n1299 = One Button Dialog(message=w1476) -> ()  [unwired: 1 in, 1 out]
              }
            }
          }
          frame True {
            n1300 = Two Button Dialog(message="是否添加开机启动" ("消息"), 1:"否" ("F按钮名称（“取消”）"), 2:"是" ("T按钮名称（“确定”）")) -> (T button?=w1479:bool)
            n1301 = case shown="真" w1479 {
              frame False {
              }
              frame True {
                n1302 = call <vilib>:"Application Directory.vi"() -> ("Application Directory"=w1485:path)
                n1303 = call "添加启动项.vi"("启动文件路径"=w1485) -> ("添加成功标记"=w1484:bool)  [unwired: 9 in, 1 out]
                n1304 = case shown="真" w1484 {
                  tunnel: ["添加开机启动失败" ("T按钮名称（“确定”）") "添加开机启动成功" ("T按钮名称（“确定”）")] -> w1483
                  frame False {
                  }
                  frame True {
                  }
                }
                n1305 = One Button Dialog(message=w1483) -> ()  [unwired: 1 in, 1 out]
              }
            }
          }
        }
      }
      event "IP": Mouse Down {
        n1306 = event-data() -> ("CtlRef"=w1488:refnum<vi>)  [unwired: 1 in, 5 out]
        n1307 = property class="Str" props=["Value"](reference=w1488) -> ()  [unwired: 1 in, 3 out]
        n1308 = local read "IP"() -> (w1490:string)
        n1309 = call "IP键盘.vi"("OldNumber"=w1490) -> ("NewNumber"=w1489:string)
        n1310 = local write "IP"(w1489) -> ()
      }
      event "PORT": Mouse Down {
        n1311 = event-data() -> ()  [unwired: 1 in, 6 out]
        n1312 = local read "PORT"() -> (w1492:string)
        n1313 = call "IP键盘.vi"("OldNumber"=w1492) -> ("NewNumber"=w1491:string)
        n1314 = local write "PORT"(w1491) -> ()
      }
      event "查询质控数据起始时间": Value Change {
        n1315 = event-data() -> ()  [unwired: 1 in, 6 out]
        n1316 = property on="窗格" class="Pane"("Origin"=T11 {"Horizontal"=1000, "Vertical"=0} ("原点")) -> ()  [unwired: 2 in, 2 out]
      }
      event "返回主界面": Value Change {
        n1317 = event-data() -> ()  [unwired: 1 in, 6 out]
        n1318 = property on="窗格" class="Pane"("Origin"=T11 {"Horizontal"=0, "Vertical"=0} ("原点")) -> ()  [unwired: 2 in, 2 out]
      }
    }
  }
  n1319 = while {
    stop <- FALSE stop-if-true
    # "心跳包"
    n1320 = global read "全局 数据发送重叠.vi" "掉线指示灯"() -> (→"掉线指示":bool)
    n1321 = Get Date/Time In Seconds() -> (seconds since 1Jan1904=w1536:timestamp)
    n1322 = local read "数据发送通道"() -> (w1511:enum16{"TCP", "VISA"})
    n1323 = local read "空闲时间"() -> (w1528:dbl)
    n1324 = case shown="\"VISA\"" "数据发送通道" {
      tunnel: [w1568 w1571] -> w1515
      tunnel: [w1567 w1569] -> w1514
      frame "TCP", Default {
        n1325 = local read "PORT"() -> (w1567:string)
        n1326 = local read "IP"() -> (w1568:string)
      }
      frame "VISA" {
        n1327 = local read "baud rate"() -> (w1570:u32)
        n1328 = local read "VISA resource name"() -> (w1571:refnum<visa-resource-name>)
        n1329 = Number To Decimal String(number=w1570) -> (decimal integer string=w1569:string)  [unwired: 1 in]
      }
    }
    n1330 = Wait (ms)(milliseconds to wait=u32 1000 ("等待时间（毫秒）")) -> ()  [unwired: 1 out]
    n1331 = global read "全局 数据发送重叠.vi" "主动上报数据中"() -> (w1495:bool)
    n1332 = local read "核查数据上传"() -> (w1523:bool)
    n1333 = local read "空闲时间"() -> (w1559:dbl)
    n1334 = local read "查询数据发送"() -> (w1526:bool)
    n1335 = Number To Decimal String(number=w1528) -> (decimal integer string=→"空闲时间/s":string)  [unwired: 1 in]
    n1336 = local read "站点设备"() -> (w1516:string)
    n1337 = local read "站点名称"() -> (w1517:string)
    n1338 = global read "全局 数据发送重叠.vi" "数据接收超时指示灯"() -> (→"数据接收超时指示灯":bool)
    n1339 = local read "MN"() -> (w1513:string)
    n1340 = Format Date/Time String(time format string (%c)="%Y/%m/%d %H:%M:%S" ("时间格式字符串(%c)"), seconds (now)=w1536) -> (date/time string=→"系统时间":string)  [unwired: 1 in]
    n1341 = local read "PW"() -> (w1512:string)
    n1342 = local read "步骤"() -> (w1553:T6)
    n1343 = case shown="\"TCP\", 默认" w1511 {
      frame "TCP", Default {
        w1572 = TRUE ("可见")
        w1573 = FALSE ("可见")
        n1344 = property on="VISA resource name" class="VISAName"("Visible"=w1573) -> ()  [unwired: 2 in, 2 out]
        n1345 = property on="baud rate" class="DigNum (严格)"("Visible"=w1573) -> ()  [unwired: 2 in, 2 out]
        n1346 = property on="IP" class="Str"("Visible"=w1572) -> ()  [unwired: 2 in, 2 out]
        n1347 = property on="PORT" class="Str"("Visible"=w1572) -> ()  [unwired: 2 in, 2 out]
      }
      frame "VISA" {
        w1574 = TRUE ("可见")
        w1575 = FALSE ("可见")
        n1348 = property on="baud rate" class="DigNum (严格)"("Visible"=w1574) -> ()  [unwired: 2 in, 2 out]
        n1349 = property on="VISA resource name" class="VISAName"("Visible"=w1574) -> ()  [unwired: 2 in, 2 out]
        n1350 = property on="IP" class="Str"("Visible"=w1575) -> ()  [unwired: 2 in, 2 out]
        n1351 = property on="PORT" class="Str"("Visible"=w1575) -> ()  [unwired: 2 in, 2 out]
      }
    }
    n1352 = local read "数据发送协议"() -> (w1508:enum16{"2005-212协议", "2017-212协议"})
    n1353 = Not(x=w1523) -> (.not. x?=w1524:bool)
    n1354 = Greater?(x=w1559, y=30.0) -> (0:w1557:bool)
    n1355 = Not(x=w1495) -> (.not. x?=w1525:bool)
    n1356 = property on="数据发送通道" class="Enum (严格)"("Visible"="锁") -> ()  [unwired: 2 in, 2 out]
    n1357 = Not(x=w1526) -> (.not. x?=w1547:bool)
    n1358 = Equal?(x=w1553, y=T6."读取数据" ("步骤")) -> (x = y?=w1551:bool)
    n1359 = Bundle By Name(cluster=T4 {"站点"="", "设备"="", "IP"="", "PORT"="", "MN"="", "PW"=""} ("配置信息"), "站点"=w1517, "设备"=w1516, "IP"=w1515, "PORT"=w1514, "MN"=w1513, "PW"=w1512) -> (→"配置信息":T4)
    n1360 = Select(t=T12."Enabled" ("禁用"), s="更改起始时间", f=T12."Disabled and Grayed Out" ("禁用")) -> (s? t:f=w1539:T12)
    n1361 = case shown="真" w1557 {
      tunnel: w1557 -> [_ w1585]
      tunnel: [FALSE w1585] -> w1554
      frame False {
      }
      frame True {
        n1362 = local read "QN"() -> (w1583:string)
        n1363 = local write "空闲时间"(0.0 ("空闲时间")) -> ()
        n1364 = local read "MN"() -> (w1582:string)
        n1365 = local read "PW"() -> (w1581:string)
        n1366 = local read "数据发送通道"() -> (w1580:enum16{"TCP", "VISA"})
        n1367 = call "数据编码.vi"("table输入"="心跳包", "QN"=w1583, "MN"=w1582, "PW"=w1581) -> ("通讯包字符串"=w1578:string)  [unwired: 10 in, 1 out]
        n1368 = local write "发送报文显示"(w1578) -> ()
        n1369 = call "VISATCP组合选择发送.vi"("数据发送通道"=w1580, "命令"="write", "写入缓冲区"=w1578) -> ("错误输出"=w1577:errorcluster)  [unwired: 9 in, 3 out]
        n1370 = call <vilib>:"Clear Errors.vi"("error in (no error)"=w1577) -> ()  [unwired: 5 in, 2 out]
      }
    }
    "心跳包" <- w1554
    n1371 = Select(t=T12."Enabled" ("禁用"), s="锁", f=T12."Disabled and Grayed Out" ("禁用")) -> (s? t:f=w1500:T12)
    n1372 = property on="数据发送起始时间" class="AbsTime (严格)"("DisabledEnum"=w1539) -> ()  [unwired: 2 in, 2 out]
    n1373 = global read "全局 时间2.vi" "跨度核查索引起始时间"() -> (→"跨度核查索引起始时间":string)
    n1374 = case shown="\"2017-212协议\", 默认" w1508 {
      tunnel: ["32" ("设备编码MN") w1562] -> w1545
      frame "2005-212协议" {
      }
      frame "2017-212协议", Default {
        n1375 = local read "系统编码选择框"() -> (w1563:string)
        n1376 = case shown="\"地表水质量监测\", 默认" w1563 {
          tunnel: ["52" ("设备编码MN") "32" ("设备编码MN") "21" ("设备编码MN")] -> w1562
          frame "污水排放过程监测" {
          }
          frame "地表水体污染源" {
          }
          frame "地表水质量监测", Default {
          }
        }
      }
    }
    n1377 = global read "全局 时间2.vi" "标样核查索引起始时间"() -> (→"标样核查索引起始时间":string)
    n1378 = global read "全局 时间2.vi" "零点核查索引起始时间"() -> (→"零点核查索引起始时间":string)
    n1379 = global read "全局 时间2.vi" "加标回收索引起始时间"() -> (→"加标回收索引起始时间":string)
    n1380 = property on="设置超时时间/min" class="DigNum (严格)"("DisabledEnum"=w1500) -> ()  [unwired: 2 in, 2 out]
    n1381 = property on="IP" class="Str"("DisabledEnum"=w1500) -> ()  [unwired: 2 in, 2 out]
    n1382 = property on="每周自动重发" class="Bool (严格)"("DisabledEnum"=w1500) -> ()  [unwired: 2 in, 2 out]
    n1383 = property on="PORT" class="Str"("DisabledEnum"=w1500) -> ()  [unwired: 2 in, 2 out]
    n1384 = local read "数据发送协议"() -> (w1507:enum16{"2005-212协议", "2017-212协议"})
    n1385 = local read "TCP服务端掉线计数"() -> (w1531:i32)
    n1386 = local read "1st Error to Convert"() -> (w1534:i32)
    n1387 = local read "TCP掉线时间节点"() -> (w1530:string)
    n1388 = property on="确定更改起始时间" class="Bool"("DisabledEnum"=w1539) -> ()  [unwired: 2 in, 2 out]
    n1389 = property on="MN" class="Str"("DisabledEnum"=w1500) -> ()  [unwired: 2 in, 2 out]
    n1390 = property on="PW" class="Str"("DisabledEnum"=w1500) -> ()  [unwired: 2 in, 2 out]
    n1391 = local read "元素"() -> (w1532:string)
    n1392 = local read "步骤"() -> (w1533:T6)
    n1393 = Equal?(x=w1507, y=enum16{"2005-212协议", "2017-212协议"}."2017-212协议" ("数据发送协议")) -> (x = y?=w1505:bool)
    n1394 = Compound Arithmetic op=AND ("复合运算")(w1505, w1551, w1547, w1525, w1524) -> (w1548:bool)
    n1395 = case shown="真" w1548 {
      frame False {
      }
      frame True {
        n1396 = local read "空闲时间"() -> (w1588:dbl)
        n1397 = Increment(x=w1588) -> (x+1=→"空闲时间":dbl)
      }
    }
    n1398 = property on="数据发送通道" class="Enum (严格)"("DisabledEnum"=w1500) -> ()  [unwired: 2 in, 2 out]
    n1399 = Bundle By Name(cluster=T3 {"1st Error to Convert "=54, "步骤 "=enum."打开连接", "元素"="实时数据", "TCP服务端掉线计数"=4, "TCP掉线时间节点"="2019/05/08 15:24:17"} ("状态信息"), "1st Error to Convert"=w1534, "步骤"=w1533, "元素"=w1532, "TCP服务端掉线计数"=w1531, "TCP掉线时间节点"=w1530) -> (→"状态信息":T3)
    n1400 = global read "全局1.vi" "通讯包字符串"() -> (w1496:string)
    n1401 = property on="重发时间" class="Enum (严格)"("DisabledEnum"=w1500) -> ()  [unwired: 2 in, 2 out]
    n1402 = property on="重发日期" class="Enum (严格)"("DisabledEnum"=w1500) -> ()  [unwired: 2 in, 2 out]
    n1403 = property on="VISA resource name" class="VISAName"("DisabledEnum"=w1500) -> ()  [unwired: 2 in, 2 out]
    n1404 = property on="判断数据反馈" class="Bool (严格)"("DisabledEnum"=w1500) -> ()  [unwired: 2 in, 2 out]
    n1405 = property on="baud rate" class="DigNum (严格)"("DisabledEnum"=w1500) -> ()  [unwired: 2 in, 2 out]
    n1406 = property on="数据发送协议" class="Enum (严格)"("DisabledEnum"=w1500) -> ()  [unwired: 2 in, 2 out]
    n1407 = property on="2011发送" class="Bool (严格)"("DisabledEnum"=w1500) -> ()  [unwired: 2 in, 2 out]
    n1408 = feedback #1(w1496) -> (w1497:string)
    n1409 = feedback-in #1(w1496) -> ()
    n1410 = global write "全局1.vi" "系统编码ST"(w1545) -> ()
    n1411 = property on="日志、参数发送" class="Bool (严格)"("DisabledEnum"=w1500) -> ()  [unwired: 2 in, 2 out]
    n1412 = property on="数据组合发送" class="Bool (严格)"("DisabledEnum"=w1500) -> ()  [unwired: 2 in, 2 out]
    n1413 = Not Equal?(x=w1496, y=w1497) -> (x != y?=w1498:bool)
    n1414 = case shown="真" w1498 {
      tunnel: w1496 -> [_ w1560]
      frame False {
      }
      frame True {
        n1415 = local write "发送报文显示"(w1560) -> ()
      }
    }
    n1416 = global read "断电保存全局.vi" "日志、参数发送"() -> (w1501:bool)
    n1417 = global read "断电保存全局.vi" "数据组合发送"() -> (w1499:bool)
    n1418 = global read "断电保存全局.vi" "判断数据反馈"() -> (w1503:bool)
    n1419 = local read "数据发送协议"() -> (w1504:enum16{"2005-212协议", "2017-212协议"})
    n1420 = global read "断电保存全局.vi" "2011发送"() -> (w1502:bool)
    n1421 = local write "日志、参数发送"(w1501) -> ()
    n1422 = local write "数据组合发送"(w1499) -> ()
    n1423 = local write "判断数据反馈"(w1503) -> ()
    n1424 = global write "全局1.vi" "数据发送版本"(w1504) -> ()
    n1425 = local write "2011发送"(w1502) -> ()
  }
  n1426 = while {
    shift-right: [w1589] -> _
    shift-left: errorcluster {"status"=FALSE, "code"=0, "source"=""} ("error out") -> [w1601]
    shift-right: [w1598] -> _
    shift-left: _ -> [w1597]
    tunnel: w54 -> [w1600]
    tunnel: w52 -> [w1596]
    shift-right: [w1594] -> _
    shift-left: w27 -> [w1595]
    tunnel: w50 -> [w1593]
    shift-right: [w1591] -> _
    shift-left: w27 -> [w1592]
    stop <- FALSE stop-if-true
    n1427 = case shown="无错误" w1601 {
      selector: w1601 -> [w1619 w1792]
      tunnel: [w1602 w1795] -> w1589
      tunnel: w1600 -> [w1618 w1790]
      tunnel: [w1603 w1794] -> w1598
      tunnel: w1597 -> [w1615 w1794]
      tunnel: w1596 -> [w1614 _]
      tunnel: w1595 -> [w1609 w1793]
      tunnel: [w1612 w1793] -> w1594
      tunnel: w1593 -> [w1611 _]
      tunnel: w1592 -> [w1606 w1789]
      tunnel: [w1605 w1789] -> w1591
      frame No Error {
        n1428 = Less?(x=w1609, y=w1611) -> (x < y?=w1610:bool)
        n1429 = Dequeue Element(queue=w1618) -> (queue out=w1616:refnum<queue>, element=w1617:T6)  [unwired: 2 in, 2 out]
        "步骤" <- w1617
        n1430 = Select(t=w1609, s=w1610, f=0) -> (s? t:f=w1608:i32)
        n1431 = local read "元素"() -> (w1604:string)
        n1432 = Index Array(array=w1614, index=w1608) -> (element=→"元素":string)
        n1433 = case shown="\"读取数据\"" w1617 {
          tunnel: w1619 -> [w1626 _ w1649 w1657 w1704 w1786]
          tunnel: w1616 -> [w1623 w1640 w1644 w1671 w1702 w1784]
          tunnel: [w1626 w1628 w1649 w1655 w1701 w1786] -> w1602
          tunnel: [string[] [] ("待发送第一条数据") w1642 _ w1684 w1705 _] -> w1603
          tunnel: w1615 -> [_ w1642 _ w1684 w1705 w1785]
          tunnel: w1604 -> [_ _ _ _ _ w1779]
          tunnel: w1608 -> [w1624 w1639 w1648 w1685 w1706 w1775]
          tunnel: [w1624 w1639 w1647 w1685 w1706 w1776] -> w1612
          tunnel: w1606 -> [w1621 w1637 w1646 _ w1697 w1773]
          tunnel: [w1621 w1637 w1646 0 ("索引") w1700 w1773] -> w1605
          frame "初始化", Default {
            n1434 = Enqueue Element(queue=w1623, element=T6."打开连接" ("元素"), timeout in ms (-1)=1000 ("超时毫秒(-1)")) -> ()  [unwired: 1 in, 3 out]
          }
          frame "打开连接" {
            (unwired) "47.98.43.76"
            # "和时通数据接入平台端接收IP端口号，61.191.22.195:10003。"
            # "47.98.43.76:6666"
            n1435 = Enqueue Element(queue=w1640, element=T6."表格比对" ("元素"), timeout in ms (-1)=1000 ("超时毫秒(-1)")) -> ()  [unwired: 1 in, 3 out]
            n1436 = local read "数据发送通道"() -> (w1627:enum16{"TCP", "VISA"})
            n1437 = call "VISATCP组合选择发送.vi"("IP"="IP", "数据发送通道"=w1627, "命令"="open", "PORT"="PORT", "VISA resource name"="VISA resource name", "baud rate"="baud rate") -> ("错误输出"=w1628:errorcluster)  [unwired: 6 in, 3 out]
            n1438 = Unbundle By Name(w1628) -> ("status"=w1636:bool, "code"=→"1st Error to Convert":i32)
            n1439 = Not(x=w1636) -> (.not. x?=→"通信状态":bool)
          }
          frame "表格比对" {
            n1440 = Enqueue Element(queue=w1644, element=T6."读取数据" ("元素"), timeout in ms (-1)=1000 ("超时毫秒(-1)")) -> ()  [unwired: 1 in, 3 out]
            n1441 = Increment(x=w1648) -> (x+1=w1647:i32)
          }
          frame "读取数据" {
            # "设置测量时间间隔"
            # "1000设置超时时间和重发次数\n1011提取监测仪表时间\n1012设置监测仪表时间\n1014提取数采仪时间\n1015设置数采仪时间\n1061提取实时数据间隔\n1062设置实时数据间隔\n1072设置数采仪访问密码"
            # "6分钟掉线重连"
            n1442 = local write "查询数据发送"(FALSE ("数据正在发送")) -> ()
            n1443 = global write "全局 数据发送重叠.vi" "掉线指示灯"(FALSE ("数据发送重叠")) -> ()
            n1444 = property on="TCP服务端掉线计数" class="DigNum (严格)"("Value"=0 ("TCP服务端掉线计数")) -> ()  [unwired: 2 in, 2 out]
            n1445 = local read "数据发送通道"() -> (w1659:enum16{"TCP", "VISA"})
            n1446 = call "VISATCP组合选择发送.vi"("数据发送通道"=w1659, "命令"="read", "error in (no error)"=w1657) -> ("读取缓冲区"=w1656:string, "错误输出"=w1655:errorcluster)  [unwired: 9 in, 2 out]
            n1447 = call "读取数据处理 (子VI).vi"("data out"=w1656) -> ("系统编码ST"=→"系统编码ST":string, "命令编码CN"=w1672:string, "设备编码MN"=→"设备编码MN":string, "密码PW"=→"密码PW":string, "数据"=w1653:string, "拆分包及应答Flag"=→"拆分包及应答Flag":string, "时间QN"=w1675:string)  [unwired: 6 in, 2 out]
            "命令编码CN" <- w1672
            "数据" <- w1653
            "时间QN" <- w1675
            n1448 = Empty String/Path?(string/path=w1656) -> (empty?=w1665:bool)
            n1449 = local read "实时小时数据上传"() -> (w1664:bool)
            n1450 = case shown="假" w1665 {
              tunnel: w1656 -> [w1692 _]
              frame False {
                n1451 = global write "全局1.vi" "数据输出"(w1692) -> ()
                n1452 = call "数据记录.vi"("写入字段"=w1692) -> ("连接的字符串"=→"读取报文显示":string)  [unwired: 10 in]
                "数据输出" <- w1692
              }
              frame True {
              }
            }
            n1453 = local read "核查数据上传"() -> (w1663:bool)
            n1454 = Not(x=w1664) -> (.not. x?=w1662:bool)
            n1455 = Not(x=w1663) -> (.not. x?=w1661:bool)
            n1456 = And(x=w1662, y=w1661) -> (x .and. y?=w1660:bool)
            n1457 = Search/Split String(string=w1675, search string/char (-)="QN=" ("搜索字符串/字符(-)")) -> (match + rest of string=w1673:string)  [unwired: 1 in, 2 out]
            n1458 = case shown="真" w1660 {
              tunnel: w1672 -> [_ w1690]
              tunnel: ["" ("命令编码CN") w1687] -> w1666
              frame False {
              }
              frame True {
                n1459 = Search/Split String(string=w1690, search string/char (-)="CN=" ("搜索字符串/字符(-)")) -> (match + rest of string=w1688:string)  [unwired: 1 in, 2 out]
                n1460 = String Subset(string=w1688, offset (0)=3 ("偏移量(0)")) -> (substring=w1687:string)  [unwired: 1 in]
              }
            }
            n1461 = String Subset(string=w1673, offset (0)=3 ("偏移量(0)")) -> (substring=→"QN":string)  [unwired: 1 in]
            n1462 = call "读取数据解析(子VI).vi"("数据"=w1653, "命令编码CN"=w1666, "队列输入"=w1671) -> ("实时数据发送时间间隔/min"=w1650:i32, "元素"=w1668:T6, "设置超时时间/min"=→"设置超时时间/min":i32, "队列输出"=w1669:refnum<queue>, "table"=w1651:string)  [unwired: 4 in]
            n1463 = local write "table元素"(w1651) -> ()
            n1464 = global write "实时数据发送间隔全局.vi" "实时数据发送间隔"(w1650) -> ()
            n1465 = local write "实时数据发送时间间隔/min"(w1650) -> ()
            n1466 = Enqueue Element(queue=w1669, element=w1668, timeout in ms (-1)=1000 ("超时毫秒(-1)")) -> ()  [unwired: 1 in, 3 out]
          }
          frame "发送数据" {
            # "table输入，选择命令编码、发送哪些数据"
            n1467 = local read "table元素"() -> (w1698:string)
            n1468 = case shown="\"报警信息\", \"操作日志\", \"核查数据\", \"空白测试\", \"跨度核查\", \"零点核查\", \"实时数据\", \"提取集成干预\", \"提取加标回收\", \"提取平行样\", \"提取实时数据\", \"提取小时数据\", \"提取仪器参数\", \"仪器参数\"" w1698 {
              tunnel: w1697 -> [w1709 w1713 w1715 w1722]
              tunnel: [w1707 w1712 w1716 w1720] -> w1695
              tunnel: [w1708 w1711 w1717 w1721] -> w1696
              frame "", Default {
                n1469 = global write "全局1.vi" "枚举"(w1709) -> ()
                n1470 = Increment(x=w1709) -> (x+1=w1708:i32)
                n1471 = Greater Or Equal?(x=w1708, y=3) -> (x >= y?=w1707:bool)
              }
              frame "反控命令" {
                n1472 = global write "全局 反控命令枚举.vi" "反控命令枚举"(w1713) -> ()
                n1473 = Increment(x=w1713) -> (x+1=w1711:i32)
                n1474 = Greater Or Equal?(x=w1711, y=2) -> (x >= y?=w1712:bool)
              }
              frame "超标留样返回", "提取监测仪表时间", "提取经纬度环境信息", "提取现场系统信息" {
                n1475 = global write "全局1.vi" "枚举"(w1715) -> ()
                n1476 = Increment(x=w1715) -> (x+1=w1717:i32)
                n1477 = Greater Or Equal?(x=w1717, y=3) -> (x >= y?=w1716:bool)
              }
              frame "报警信息", "操作日志", "核查数据", "空白测试", "跨度核查", "零点核查", "实时数据", "提取集成干预", "提取加标回收", "提取平行样", "提取实时数据", "提取小时数据", "提取仪器参数", "仪器参数" {
                n1478 = global read "全局 小时数据发送次数.vi" "小时数据发送次数"() -> (w1724:i32)
                n1479 = global read "全局 数据数组大小.vi" "数据数组大小"() -> (w1719:i32)
                n1480 = Greater Or Equal?(x=w1724, y=w1719) -> (x >= y?=w1725:bool)
                n1481 = case shown="真" w1725 {
                  tunnel: w1722 -> [w1730 w1737]
                  tunnel: [w1730 w1731] -> w1726
                  frame False {
                  }
                  frame True {
                    n1482 = global read "全局 小时数据发送次数.vi" "小时数据发送次数"() -> (w1736:i32)
                    n1483 = global read "全局 数据数组大小.vi" "数据数组大小"() -> (w1733:i32)
                    n1484 = Equal To 0?(x=w1736) -> (x = 0?=w1735:bool)
                    n1485 = Equal To 0?(x=w1733) -> (x = 0?=w1734:bool)
                    n1486 = And(x=w1735, y=w1734) -> (x .and. y?=w1732:bool)
                    n1487 = case shown="真" w1732 {
                      tunnel: w1737 -> [w1739 _]
                      tunnel: [w1738 0 ("索引")] -> w1731
                      frame False {
                        n1488 = Increment(x=w1739) -> (x+1=w1738:i32)
                      }
                      frame True {
                      }
                    }
                  }
                }
                n1489 = global write "全局1.vi" "枚举"(w1726) -> ()
                n1490 = Equal To 0?(x=w1726) -> (x = 0?=w1727:bool)
                n1491 = case shown="真" w1727 {
                  tunnel: w1726 -> [w1728 _]
                  tunnel: [w1728 1] -> w1721
                  frame False {
                  }
                  frame True {
                  }
                }
                n1492 = Greater Or Equal?(x=w1721, y=2) -> (x >= y?=w1720:bool)
              }
            }
            n1493 = flat-sequence {
              tunnel: "table元素" -> [w1752]
              tunnel: w1704 -> [w1751]
              tunnel: [w1747] -> w1703
              tunnel: [w1756] -> w1701
              tunnel: w1703 -> [w1756]
              tunnel: w1702 -> [w1755]
              tunnel: w1695 -> [w1754]
              frame #0 {
                # "数据记录"
                # "数据编码"
                n1494 = local read "MN"() -> (w1744:string)
                n1495 = local read "QN"() -> (w1750:string)
                n1496 = local read "PW"() -> (w1743:string)
                n1497 = call "数据编码.vi"("table输入"=w1752, "错误常量 2"=w1751, "QN"=w1750, "MN"=w1744, "PW"=w1743) -> ("错误常量"=w1749:errorcluster, "通讯包字符串"=w1748:string)  [unwired: 9 in]
                n1498 = local read "数据发送通道"() -> (w1746:enum16{"TCP", "VISA"})
                n1499 = call "数据记录.vi"("写入字段"=w1748) -> ("连接的字符串"=→"发送报文显示":string)  [unwired: 10 in]
                n1500 = call "VISATCP组合选择发送.vi"("数据发送通道"=w1746, "命令"="write", "error in (no error)"=w1749, "写入缓冲区"=w1748) -> ("错误输出"=w1747:errorcluster)  [unwired: 8 in, 3 out]
              }
              frame #1 {
                n1501 = case shown="真" w1754 {
                  tunnel: w1755 -> [w1757 w1769]
                  frame False {
                    n1502 = Enqueue Element(queue=w1757, element=T6."发送数据" ("元素")) -> ()  [unwired: 2 in, 3 out]
                  }
                  frame True {
                    n1503 = local read "TCP服务端掉线计数"() -> (w1764:i32)
                    n1504 = Obtain Queue(name (unnamed)="重发掉线数据" ("名称（未命名）"), element data type=T13."水样测试") -> (queue out=w1762:refnum<queue>, error out=w1763:errorcluster)  [unwired: 3 in, 1 out]
                    n1505 = Get Queue Status(queue=w1762, error in (no error)=w1763) -> (# elements in queue=w1766:i32)  [unwired: 1 in, 7 out]
                    n1506 = Not Equal To 0?(x=w1766) -> (x != 0?=w1767:bool)
                    n1507 = Greater Or Equal?(x=w1764, y=1) -> (x >= y?=w1768:bool)
                    n1508 = And(x=w1767, y=w1768) -> (x .and. y?=w1760:bool)
                    n1509 = case shown="真" w1760 {
                      tunnel: [T6."读取数据" ("元素") T6."表格比对" ("元素")] -> w1770
                      frame False {
                      }
                      frame True {
                      }
                    }
                    n1510 = Enqueue Element(queue=w1769, element=w1770) -> ()  [unwired: 2 in, 3 out]
                  }
                }
              }
            }
            n1511 = case shown="假" w1695 {
              tunnel: w1696 -> [w1741 _]
              tunnel: [w1741 1 ("索引")] -> w1700
              frame False {
              }
              frame True {
              }
            }
            "查询数据发送" <- TRUE
          }
          frame "数据处理" {
            n1512 = local write "空闲时间"(0.0 ("空闲时间")) -> ()
            n1513 = local read "心跳包"() -> (w1781:bool)
            n1514 = Equal?(x=w1779, y="实时数据") -> (x = y?=w1777:bool)
            n1515 = case shown="假" w1781 {
              tunnel: w1785 -> [w1788 _]
              tunnel: w1779 -> [w1787 _]
              frame False {
                n1516 = call "插入单条数据.vi"("table输入"=w1787, "插入数据"=w1788) -> ()  [unwired: 8 in, 2 out]
              }
              frame True {
              }
            }
            n1517 = Select(t=0, s=w1777, f=w1775) -> (s? t:f=w1776:i32)
            n1518 = Enqueue Element(queue=w1784, element=T6."表格比对" ("元素"), timeout in ms (-1)=1000 ("超时毫秒(-1)")) -> ()  [unwired: 1 in, 3 out]
          }
        }
      }
      frame Error {
        n1519 = Unbundle By Name(w1792) -> ("code"=w1791:i32)
        n1520 = case shown="0, 默认" w1791 {
          tunnel: w1792 -> [w1797 w1807 w1836 w1860]
          tunnel: [w1803 w1820 w1849 w1860] -> w1796
          tunnel: w1790 -> [w1804 w1815 w1844 w1857]
          frame 0, Default {
            n1521 = Flush Queue(queue=w1804) -> (queue out=w1802:refnum<queue>)  [unwired: 1 in, 2 out]
            n1522 = global write "全局 数据发送重叠.vi" "掉线指示灯"(TRUE ("掉线指示灯")) -> ()
            n1523 = local read "数据发送通道"() -> (w1799:enum16{"TCP", "VISA"})
            n1524 = Enqueue Element(queue=w1802, element=T6."初始化" ("元素"), timeout in ms (-1)=1000 ("超时毫秒(-1)")) -> ()  [unwired: 1 in, 3 out]
            n1525 = call "VISATCP组合选择发送.vi"("数据发送通道"=w1799, "命令"="close", "error in (no error)"=w1797) -> ("错误输出"=w1798:errorcluster)  [unwired: 9 in, 3 out]
            n1526 = call <vilib>:"Clear Errors.vi"("error in (no error)"=w1798) -> ("error out"=w1803:errorcluster)  [unwired: 5 in, 1 out]
          }
          frame 63 {
            # "TCP服务器端口掉线"
            n1527 = Flush Queue(queue=w1815) -> (queue out=w1816:refnum<queue>)  [unwired: 1 in, 2 out]
            n1528 = global write "全局 数据发送重叠.vi" "掉线指示灯"(TRUE ("掉线指示灯")) -> ()
            n1529 = property on="TCP服务端掉线计数" class="DigNum (严格)"() -> ("Value"=w1814:i32)  [unwired: 2 in, 2 out]
            n1530 = property on="TCP服务端掉线计数" class="DigNum (严格)"() -> ("Value"=w1819:i32)  [unwired: 2 in, 2 out]
            n1531 = local read "数据发送通道"() -> (w1809:enum16{"TCP", "VISA"})
            n1532 = Increment(x=w1819) -> (x+1=w1817:i32)
            n1533 = Less Or Equal?(x=w1814, y=1) -> (x <= y?=w1812:bool)
            n1534 = Enqueue Element(queue=w1816, element=T6."初始化" ("元素"), timeout in ms (-1)=1000 ("超时毫秒(-1)")) -> ()  [unwired: 1 in, 3 out]
            n1535 = case shown="真" w1812 {
              frame False {
                n1536 = local write "TCP掉线时间节点"("TCP掉线时间节点") -> ()
                n1537 = global write "全局 数据发送重叠.vi" "TCP掉线时间节点"("TCP掉线时间节点") -> ()
              }
              frame True {
                n1538 = call <vilib>:"Application Directory.vi"() -> ("Application Directory"=w1831:path)
                n1539 = Get Date/Time In Seconds() -> (seconds since 1Jan1904=w1833:timestamp)
                n1540 = Build Path(base path=w1831, name or relative path="data\\Set.ini" ("名称或相对路径")) -> (appended path=w1832:path)
                n1541 = Format Date/Time String(time format string (%c)="%Y%m%d%H%M%S%3u" ("时间格式字符串(%c)"), seconds (now)=w1833) -> (date/time string=w1835:string)  [unwired: 1 in]
                n1542 = call "格式时间字符串.vi"("字符串"=w1835) -> ("连接的字符串"=w1823:string)  [unwired: 10 in]
                n1543 = call <vilib>:"Open Config Data.vi"("configuration file path"=w1832) -> ("error out"=w1828:errorcluster, "refnum"=w1829:T8)  [unwired: 8 in, 1 out]
                n1544 = local write "TCP掉线时间节点"(w1823) -> ()
                n1545 = call-poly <vilib>:"Write Key.vi"("section"="掉线时间存储", "error in (no error)"=w1828, "value"=w1823, "key"="掉线时间", "refnum"=w1829) -> ("error out"=w1826:errorcluster, "refnum out"=w1827:T8)  [unwired: 4 in, 1 out]
                n1546 = call <vilib>:"Close Config Data.vi"("error in (no error)"=w1826, "refnum"=w1827) -> ()  [unwired: 8 in, 2 out]
              }
            }
            n1547 = property on="TCP服务端掉线计数" class="DigNum (严格)"("Value"=w1817) -> ()  [unwired: 2 in, 2 out]
            n1548 = call "VISATCP组合选择发送.vi"("数据发送通道"=w1809, "命令"="close", "error in (no error)"=w1807) -> ("错误输出"=w1808:errorcluster)  [unwired: 9 in, 3 out]
            n1549 = call <vilib>:"Clear Errors.vi"("error in (no error)"=w1808) -> ("error out"=w1820:errorcluster)  [unwired: 5 in, 1 out]
          }
          frame 54 {
            # "TCP服务器端口掉线"
            n1550 = Flush Queue(queue=w1844) -> (queue out=w1845:refnum<queue>)  [unwired: 1 in, 2 out]
            n1551 = global write "全局 数据发送重叠.vi" "掉线指示灯"(TRUE ("掉线指示灯")) -> ()
            n1552 = property on="TCP服务端掉线计数" class="DigNum (严格)"() -> ("Value"=w1843:i32)  [unwired: 2 in, 2 out]
            n1553 = property on="TCP服务端掉线计数" class="DigNum (严格)"() -> ("Value"=w1848:i32)  [unwired: 2 in, 2 out]
            n1554 = local read "数据发送通道"() -> (w1838:enum16{"TCP", "VISA"})
            n1555 = Increment(x=w1848) -> (x+1=w1846:i32)
            n1556 = Less Or Equal?(x=w1843, y=1) -> (x <= y?=w1841:bool)
            n1557 = Enqueue Element(queue=w1845, element=T6."初始化" ("元素"), timeout in ms (-1)=1000 ("超时毫秒(-1)")) -> ()  [unwired: 1 in, 3 out]
            n1558 = case shown="真" w1841 {
              frame False {
                n1559 = local read "TCP掉线时间节点"() -> (w1851:string)
                n1560 = local write "TCP掉线时间节点"(w1851) -> ()
                n1561 = global write "全局 数据发送重叠.vi" "TCP掉线时间节点"(w1851) -> ()
              }
              frame True {
                n1562 = Get Date/Time In Seconds() -> (seconds since 1Jan1904=w1853:timestamp)
                n1563 = Format Date/Time String(time format string (%c)="%Y%m%d%H%M%S%3u" ("时间格式字符串(%c)"), seconds (now)=w1853) -> (date/time string=w1855:string)  [unwired: 1 in]
                n1564 = call "格式时间字符串.vi"("字符串"=w1855) -> ("连接的字符串"=w1852:string)  [unwired: 10 in]
                n1565 = local write "TCP掉线时间节点"(w1852) -> ()
              }
            }
            n1566 = property on="TCP服务端掉线计数" class="DigNum (严格)"("Value"=w1846) -> ()  [unwired: 2 in, 2 out]
            n1567 = call "VISATCP组合选择发送.vi"("数据发送通道"=w1838, "命令"="close", "error in (no error)"=w1836) -> ("错误输出"=w1837:errorcluster)  [unwired: 9 in, 3 out]
            n1568 = call <vilib>:"Clear Errors.vi"("error in (no error)"=w1837) -> ("error out"=w1849:errorcluster)  [unwired: 5 in, 1 out]
          }
          frame 56 {
            n1569 = Flush Queue(queue=w1857) -> (queue out=w1858:refnum<queue>)  [unwired: 1 in, 2 out]
            n1570 = Enqueue Element(queue=w1858, element=T6."读取数据" ("元素"), timeout in ms (-1)=1000 ("超时毫秒(-1)")) -> ()  [unwired: 1 in, 3 out]
          }
        }
        n1571 = call <vilib>:"Clear Errors.vi"("error in (no error)"=w1796) -> ("error out"=w1795:errorcluster)  [unwired: 5 in, 1 out]
      }
    }
    n1572 = Wait (ms)(milliseconds to wait=u32 300 ("等待时间（毫秒）")) -> ()  [unwired: 1 out]
  }
  n1573 = flat-sequence {
    frame #0 {
      w1875 = "数据发送协议"
      w1882 = "线程一自主部署站点保存"
      w1898 = "数据发送通道" ("section")
      (unwired) path "C:/LabVIEW Project/builds/平台数据发送系统" ("Application Directory")
      w1948 = "" ("参数")
      w1861 = FALSE ("数据发送中断")
      w1919 = 0 ("数值")
      # "版本改动:增加了远程反控命令，和仪器端双向通讯，modbus TCP读写"
      # "ST参数选择"
      n1574 = property class="VI"() -> ("Panel"=w1952:refnum<vi>)  [unwired: 2 in, 2 out]
      n1575 = global write "全局 实时数据参数.vi" "参数"(w1948) -> ()
      n1576 = local write "核查数据上传"(w1861) -> ()
      n1577 = local write "查询数据发送"(w1861) -> ()
      n1578 = local write "心跳包"(w1861) -> ()
      n1579 = global write "全局 小时数据发送次数.vi" "小时数据发送次数"(w1919) -> ()
      n1580 = local write "实时小时数据上传"(w1861) -> ()
      n1581 = local write "系统状态改变"(w1861) -> ()
      n1582 = property class="Pnl"(reference=w1952) -> ("Panes[]"=w1951:refnum<vi>[])  [unwired: 1 in, 2 out]
      n1583 = global write "全局 实时数据参数.vi" "data"(string[][] [] ("data")) -> ()
      n1584 = property on="窗格" class="Pane"("Origin"=T11 {"Horizontal"=0, "Vertical"=0} ("原点")) -> ()  [unwired: 2 in, 2 out]
      n1585 = local write "空闲时间"(0.0 ("try")) -> ()
      n1586 = global write "全局1.vi" "枚举"(enum16{"返回请求应答", "上传数据", "返回执行结果"}."返回请求应答" ("枚举")) -> ()
      n1587 = global write "全局 实时数据参数.vi" "连接的字符串"(w1948) -> ()
      n1588 = call <vilib>:"Application Directory.vi"() -> ("Application Directory"=w1946:path)
      n1589 = for {
        tunnel: w1951 -> [w1963] mode=indexing
        tunnel: u32 15592941 ("窗格颜色") -> [w1964]
        n1590 = property class="Pane"(reference=w1963, "PaneColor"=w1964) -> ()  [unwired: 1 in, 2 out]
      }
      n1591 = Build Path(base path=w1946, name or relative path="data\\Set.ini" ("名称或相对路径")) -> (appended path=w1944:path)
      n1592 = call <vilib>:"Open Config Data.vi"("configuration file path"=w1944) -> ("error out"=w1942:errorcluster, "refnum"=w1943:T8)  [unwired: 8 in, 1 out]
      n1593 = call <vilib>:"Application Directory.vi"() -> ("Application Directory"=w1909:path)
      n1594 = call-poly <vilib>:"Read Key.vi"("section"=w1882, "error in (no error)"=w1942, "key"="站点名称", "refnum"=w1943) -> ("error out"=w1939:errorcluster, "value"=w1896:string, "refnum out"=w1940:T8)  [unwired: 4 in, 1 out]
      n1595 = call <vilib>:"Application Directory.vi"() -> ("Application Directory"=w1865:path)
      n1596 = call <vilib>:"Application Directory.vi"() -> ("Application Directory"=w1905:path)
      n1597 = call <vilib>:"Recursive File List.vi"("pattern"="*.exe", "Folder Path"=w1909) -> ("All Files in Dir"=w1917:path[])  [unwired: 5 in, 4 out]
      n1598 = Build Path(base path=w1865, name or relative path="data\\sys.ini" ("名称或相对路径")) -> (appended path=w1863:path)
      n1599 = local write "站点名称"(w1896) -> ()
      n1600 = Build Path(base path=w1905, name or relative path="data\\background.jpg" ("名称或相对路径")) -> (appended path=w1904:path)
      n1601 = call <vilib>:"Open Config Data.vi"("configuration file path"=w1863) -> ("error out"=w1869:errorcluster, "refnum"=w1868:T8)  [unwired: 8 in, 1 out]
      n1602 = Index Array(array=w1917) -> (element=w1916:path)  [unwired: 1 in]
      n1603 = Get Date/Time In Seconds() -> (seconds since 1Jan1904=w1956:timestamp)
      n1604 = call <vilib>:"Read JPEG File.vi"("path to JPEG file"=w1904) -> ("error out"=w1902:errorcluster, "image data"=w1903:T14)  [unwired: 8 in, 1 out]
      n1605 = vi-ref "断电保存全局.vi"() -> (w1867:refnum<vi>)
      n1606 = Format Date/Time String(time format string (%c)="%Y%m%d%H%M%S%3u" ("时间格式字符串(%c)"), seconds (now)=w1956) -> (date/time string=w1955:string)  [unwired: 1 in]
      n1607 = call-poly <vilib>:"Read Key.vi"("section"=w1882, "error in (no error)"=w1939, "key"="站点设备", "refnum"=w1940) -> ("error out"=w1936:errorcluster, "value"=w1895:string, "refnum out"=w1937:T8)  [unwired: 4 in, 1 out]
      n1608 = File/Directory Info(path=w1916) -> (last mod=w1915:timestamp)  [unwired: 1 in, 6 out]
      n1609 = call <vilib>:"FileVersionInfo.vi"("Application Path in"=w1916) -> ("error out"=w1901:errorcluster, "File Version Info"=w1912:string)  [unwired: 7 in, 2 out]
      n1610 = call <userlib>:"Read Panel from INI__ogtk.vi"("error in (no error)"=w1869, "VI ref"=w1867, "refnum"=w1868) -> ("error out"=w1862:errorcluster, "refnum out"=w1866:T8)  [unwired: 7 in]
      n1611 = property on="窗格" class="Pane"("BackgroundImage"=w1903) -> ()  [unwired: 2 in, 2 out]
      n1612 = Format Date/Time String(time format string (%c)="\n%Y%m%d%H%M" ("时间格式字符串(%c)"), seconds (now)=w1915) -> (date/time string=w1911:string)  [unwired: 1 in]
      n1613 = local write "站点设备"(w1895) -> ()
      n1614 = case shown="错误" w1862 {
        frame No Error {
        }
        frame Error {
          n1615 = global write "断电保存全局.vi" "判断数据反馈"(TRUE ("判断数据反馈")) -> ()
        }
      }
      n1616 = Search and Replace String(input string=w1955, search string="." ("搜索字符串")) -> (result string=w1953:string)  [unwired: 6 in, 3 out]
      n1617 = call <vilib>:"Close Config Data.vi"("error in (no error)"=w1862, "refnum"=w1866) -> ()  [unwired: 8 in, 2 out]
      n1618 = call-poly <vilib>:"Read Key.vi"("section"=w1882, "error in (no error)"=w1936, "key"="IP", "refnum"=w1937) -> ("error out"=w1933:errorcluster, "value"=w1894:string, "refnum out"=w1934:T8)  [unwired: 4 in, 1 out]
      n1619 = Concatenate Strings("V" ("字符串"), w1912, w1911) -> (→"软件版本":string)
      n1620 = local write "QN"(w1953) -> ()
      n1621 = call <vilib>:"Simple Error Handler.vi"("error in (no error)"=w1901) -> ()  [unwired: 4 in, 5 out]
      n1622 = call <vilib>:"Simple Error Handler.vi"("error in (no error)"=w1902) -> ()  [unwired: 4 in, 5 out]
      n1623 = local write "IP"(w1894) -> ()
      n1624 = call-poly <vilib>:"Read Key.vi"("section"=w1882, "error in (no error)"=w1933, "key"="PORT", "refnum"=w1934) -> ("error out"=w1929:errorcluster, "value"=w1893:string, "refnum out"=w1930:T8)  [unwired: 4 in, 1 out]
      n1625 = call <vilib>:"Application Directory.vi"() -> ("Application Directory"=w1908:path)
      n1626 = local write "PORT"(w1893) -> ()
      n1627 = call "查询启动项.vi"("启动文件路径"=w1908) -> ("包含启动项"=w1907:bool)  [unwired: 9 in, 1 out]
      n1628 = call-poly <vilib>:"Read Key.vi"("section"=w1882, "error in (no error)"=w1929, "key"="MN", "refnum"=w1930) -> ("error out"=w1889:errorcluster, "value"=w1892:string, "refnum out"=w1890:T8)  [unwired: 4 in, 1 out]
      n1629 = local write "MN"(w1892) -> ()
      n1630 = local write "开机启动"(w1907) -> ()
      n1631 = call-poly <vilib>:"Read Key.vi"("section"=w1882, "error in (no error)"=w1889, "key"="PW", "refnum"=w1890) -> ("error out"=w1887:errorcluster, "value"=w1891:string, "refnum out"=w1888:T8)  [unwired: 4 in, 1 out]
      n1632 = local write "PW"(w1891) -> ()
      n1633 = call-poly <vilib>:"Read Key.vi"("section"=w1882, "error in (no error)"=w1887, "key"="VISA", "refnum"=w1888) -> ("error out"=w1883:errorcluster, "value"=w1885:string, "refnum out"=w1884:T8)  [unwired: 4 in, 1 out]
      n1634 = local write "VISA resource name"(w1885) -> ()
      n1635 = call-poly <vilib>:"Read Key.vi"("section"=w1882, "error in (no error)"=w1883, "key"="BAUDRATE", "refnum"=w1884) -> ("error out"=w1878:errorcluster, "value"=w1880:i32, "refnum out"=w1879:T8)  [unwired: 4 in, 1 out]
      n1636 = local write "baud rate"(w1880) -> ()
      n1637 = call-poly <vilib>:"Read Key.vi"("section"="系统编码选择", "error in (no error)"=w1878, "key"="系统编码", "refnum"=w1879) -> ("error out"=w1923:errorcluster, "value"=w1925:string, "refnum out"=w1924:T8)  [unwired: 4 in, 1 out]
      n1638 = local write "系统编码选择框"(w1925) -> ()
      n1639 = call-poly <vilib>:"Read Key.vi"("section"="掉线时间存储", "error in (no error)"=w1923, "key"="掉线时间", "refnum"=w1924) -> ("error out"=w1899:errorcluster, "value"=w1920:string, "refnum out"=w1900:T8)  [unwired: 4 in, 1 out]
      n1640 = global write "全局 数据发送重叠.vi" "TCP掉线时间节点"(w1920) -> ()
      n1641 = local write "TCP掉线时间节点"(w1920) -> ()
      n1642 = call-poly <vilib>:"Read Key.vi"("section"=w1898, "error in (no error)"=w1899, "key"=w1898, "refnum"=w1900) -> ("error out"=w1876:errorcluster, "value"=w1897:i32, "refnum out"=w1877:T8)  [unwired: 4 in, 1 out]
      n1643 = local write "数据发送通道"(w1897) -> ()
      n1644 = call-poly <vilib>:"Read Key.vi"("section"=w1875, "error in (no error)"=w1876, "key"=w1875, "refnum"=w1877) -> ("error out"=w1873:errorcluster, "value"=w1871:i32, "found?"=w1872:bool, "refnum out"=w1874:T8)  [unwired: 4 in]
      n1645 = case shown="假" w1872 {
        tunnel: w1871 -> [_ w1962]
        tunnel: [1 ("value") w1962] -> w1870
        frame False {
        }
        frame True {
        }
      }
      n1646 = local write "数据发送协议"(w1870) -> ()
      n1647 = call <vilib>:"Close Config Data.vi"("error in (no error)"=w1873, "refnum"=w1874) -> ()  [unwired: 8 in, 2 out]
      "TCP服务端掉线计数" <- w1919
    }
  }
  n1648 = property class="VI"(reference=w29) -> ("Name"=w30:string)  [unwired: 1 in, 2 out]
  n1649 = Open VI Reference(type specifier VI Refnum (for type only)=refnum<vi> refnum, vi path=w30, options=128 ("选项")) -> (vi reference=w32:refnum<vi>, error out=w34:errorcluster)  [unwired: 3 in]
  n1650 = call-by-ref "?"(reference=w32, error in=w34) -> (reference out=w36:refnum<vi>, error out=w35:errorcluster)  [unwired: 11 in, 1 out]
  n1651 = Close Reference(reference=w36, error in (no error)=w35) -> ()  [unwired: 1 out]
